vi "Modules - Communications V1.vi"() -> ()   [LabVIEW 2019]
uses:
  Controls/UDP - Command.ctl
  Controls/Communications - State.ctl
  Controls/FTDI - Communication.ctl
  Controls/eFGV States.ctl
  Controls/Communications - Data Structure.ctl
  Controls/Communication - Write Data.ctl
  Controls/UDP - Communication.ctl
  Controls/UDP - Event.ctl
  Controls/UDP - Status.ctl
  Controls/Global - Hold.vi
  Controls/Global - Handle V1.vi
  Controls/Global - IP Address.vi
  <vilib>/Instr/_visa.llb/VISA Serial Break (Instr).vi
  Controls/Global - Device.vi
  Controls/Global - Comport.vi
  Controls/Global - Data UDP.vi
  Controls/Global - Done.vi
  Controls/Global - Channel.vi
  Controls/Global - Unit.vi
  Controls/Global - Rendezvous.vi
panel:
  out "8":T1
  out "Prev 8":bool
  out "Success8":bool
  out "8":T2
  out "loop 8":i32
  out "9":T1
  out "Prev 9":bool
  out "Success9":bool
  out "9":T2
  out "loop 9":i32
  out "10":T1
  out "Prev 10":bool
  out "Success10":bool
  out "10":T2
  out "loop 10":i32
  out "11":T1
  out "Prev 11":bool
  out "Success11":bool
  out "11":T2
  out "loop 11":i32
  out "12":T1
  out "Prev 12":bool
  out "Success12":bool
  out "12":T2
  out "loop 12":i32
  out "13":T1
  out "Prev 13":bool
  out "Success13":bool
  out "13":T2
  out "loop 13":i32
  out "14":T1
  out "Prev 14":bool
  out "Success14":bool
  out "14":T2
  out "loop 14":i32
  out "15":T1
  out "Prev15":bool
  out "Success15":bool
  out "15":T2
  out "loop 15":i32
  out "4":T1
  out "Prev 4":bool
  out "Success4":bool
  out "5":T2
  out "loop 4":i32
  out "5":T1
  out "Prev 5":bool
  out "Success5":bool
  out "5":T2
  out "loop 5":i32
  out "6":T1
  out "Prev 6":bool
  out "Success6":bool
  out "6":T2
  out "loop 6":i32
  out "7":T1
  out "Prev 7":bool
  out "Success7":bool
  out "7":T2
  out "loop 7":i32
  out "UI loop":i32
  out "Success3":bool
  out "Success2":bool
  out "Success1":bool
  out "Success0":bool
  in  "stop":bool
  out "Prev 3":bool
  out "Prev 2":bool
  out "Prev 1":bool
  out "Prev 0":bool
  out "loop 3":i32
  out "loop 2":i32
  out "loop 1":i32
  in  "Enable Termination\nChar (T)":bool=TRUE
  in  "Break":bool
  out "loop 0":i32
  out "3":T2
  out "2":T2
  out "1":T2
  out "0":T2
  out "3":T1
  out "2":T1
  out "1":T1
  out "0":T1
  out "Device":string[](array[string])
  out "SN":string[](array[string])
  out "Stop":bool=TRUE
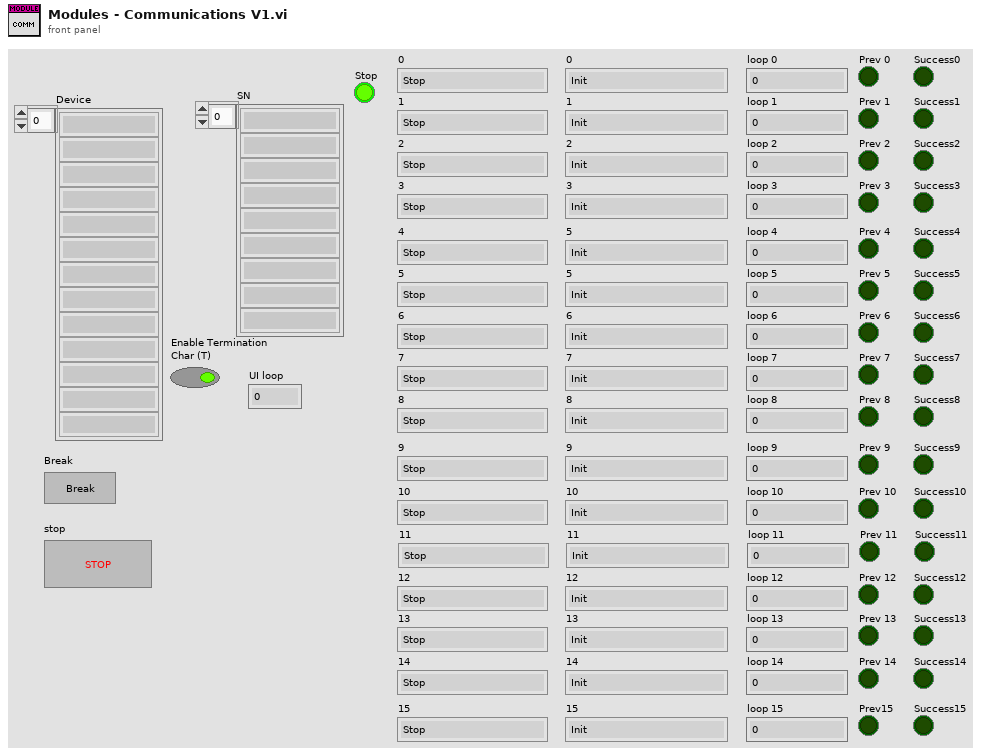
[diagram p1: front panel]
types:
  T1 = typedef "UDP - Command.ctl" = enum16{"Stop", "Jog Up", "Jog Down", "Ramp Up", "Ramp Down", "PID Target", "PID Ramp", "Disp Run", "Read Ch Data", "Zero Channel", "Zero Disp", "Read Sensor", "Write Sensor", "Read ADC", "Write ADC", "Read PID", "Write PID", "Read Test", "Write Test", "Read System", "Write System", "Read Datalog", "Read Datalog Sensor"}
  T2 = typedef "Communications - State.ctl" = enum16{"Init", "Idle", "Command", "Get IP Address", "Release Rendezvous", "Feedback", "Close"}
  T3 = enum32{"Invalid", "Standard", "Closed", "Hidden", "Minimized", "Maximized"}
  T4 = typedef "FTDI - Communication.ctl" = cluster{"IP":string, "CMD":T1, "Port":string, "Datalog?":bool, "Float":dbl}
  T5 = typedef "eFGV States.ctl" = enum16{"Init", "Read", "Write", "Exit"}
  T6 = typedef "Communications - Data Structure.ctl" = cluster{"UDP CMD":T4, "Unit?":bool, "Read Unit":bool[], "Trig?":bool, "UDP Info":cluster{"IP Address":string, "port":string, "UDP ref":refnum<k16>}[], "DataLogger":bool[], "VISA Ref":refnum<event-registration>, "Float":sgl, "Data":T7, "UDP Event Ref":refnum<event-registration>, "UDP ref":refnum<k16>, "Read Sensor":u8}
  T7 = typedef "Communication - Write Data.ctl" = cluster{"Test":cluster{"Target Load":sgl, "Target Disp":sgl, "Rate":sgl, "Speed":sgl}, "Sensor":cluster{"Name":string[], "Unit":string[], "Decimal Point":u8[], "Ch Log":u8[], "H Alarm":u8[], "L Alarm":u8[], "H Limit":sgl[], "L Limit":sgl[], "Filter":u8[], "Gain":u8[], "Calib Type":u32[]}, "PID":cluster{"SP":sgl, "PV":sgl, "kP":sgl, "kI":sgl, "kD":sgl, "FF":sgl, "Err Band":sgl, "Max":i32, "Min":i32, "Ts":u32, "Out":i32, "Mode":u8}, "ADC":cluster{"Active Ch":u8[], "Filter Type":u8, "Post Filter":u8[], "Gain":u8[], "FS":u16, "IntOC":u8, "IntFC":u8, "SysOC":u8, "Cofficient":dbl[], "K":dbl[], "Max":i32}, "System":cluster{"Out Type":u8, "Inverse":u8, "Monitor":u8, "Reserve":u8, "ACC Time":u32, "Pulse Rev":u32, "Stroke":u32, "Auto Off":u32, "Gear Ratio":sgl, "Pitch":sgl, "Max Speed":u32, "Jog Speed":u32, "Disp Coff":sgl, "Max Load":u32}, "Index":enum16{"Ch1", "Ch2", "Ch3", "Ch4", "Ch5", "Ch6", "Ch7", "Ch8", "Ch9", "Ch10", "Ch11", "Ch12", "Ch13", "Ch14", "Ch15", "Ch16"}, "Datalog":enum16{"Ch1-Ch16", "Ch17-Ch32", "Ch32-Ch48", "Ch49-Ch64", "Empty"}}
  T8 = typedef "UDP - Event.ctl" = u16
  T9 = typedef "UDP - Status.ctl" = u16
  T10 = cluster{"Channels":cluster{"Ch1":sgl, "Ch2":sgl, "Ch3":sgl, "Ch4":sgl, "Ch5":sgl, "Ch6":sgl, "Ch7":sgl, "Ch8":sgl, "Ch9":sgl, "Ch10":sgl, "Ch11":sgl, "Ch12":sgl, "Ch13":sgl, "Ch14":sgl, "Ch15":sgl, "Ch16":sgl}, "Event":T8, "Status":T9, "IP":string}
  T11 = cluster{"Name":string[], "Unit":string[], "Decimal Point":u8[], "Ch Log":u8[], "H Alarm":u8[], "L Alarm":u8[], "H Limit":sgl[], "L Limit":sgl[], "Filter":u8[], "Gain":u8[], "Calib Type":u32[]}
  T12 = cluster{"Ch1 Unit":string, "Ch2 Unit":string, "Ch1 Decimal":u8, "Ch2 Decimal":u8, "Ch1 Cal Type":u8, "Ch2 Cal Type":u8}
  T13 = cluster{"Ch1 Status":u8, "Ch2 Status":u8, "DO":bool[], "DI":bool[], "Ch1 Data":sgl, "Ch2 Data":sgl}
  T14 = cluster{"Channels":cluster{"Ch1":sgl, "Ch2":sgl, "Ch3":sgl, "Ch4":sgl, "Ch5":sgl, "Ch6":sgl, "Ch7":sgl, "Ch8":sgl, "Ch9":sgl, "Ch10":sgl, "Ch11":sgl, "Ch12":sgl, "Ch13":sgl, "Ch14":sgl, "Ch15":sgl, "Ch16":sgl}, "Event":T8, "Status":T9, "IP":string}[]
  T15 = cluster{"Name":string[], "Unit":string[], "Decimal Point":u8[], "Ch Log":u8[], "H Alarm":u8[], "L Alarm":u8[], "H Limit":sgl[], "L Limit":sgl[], "Filter":u8[], "Gain":u8[], "Calib Type":u32[]}[]
  T16 = typedef "Rendezvous RefNum" = refnum<k1>
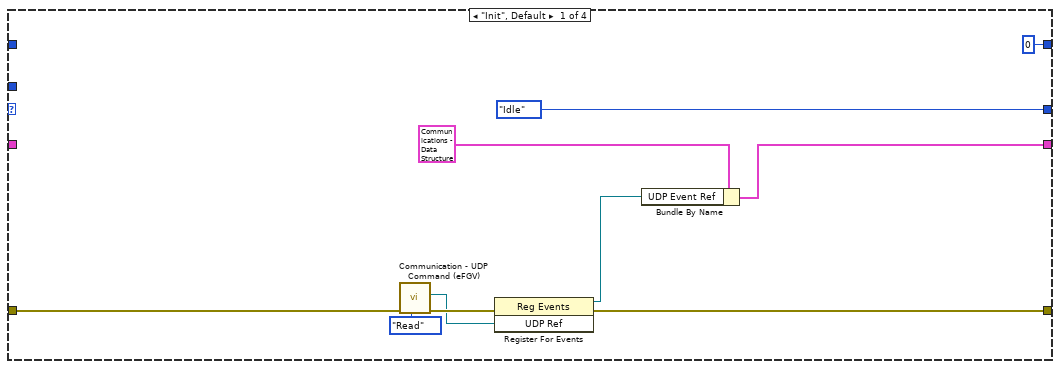
[diagram p2: hidden frame]
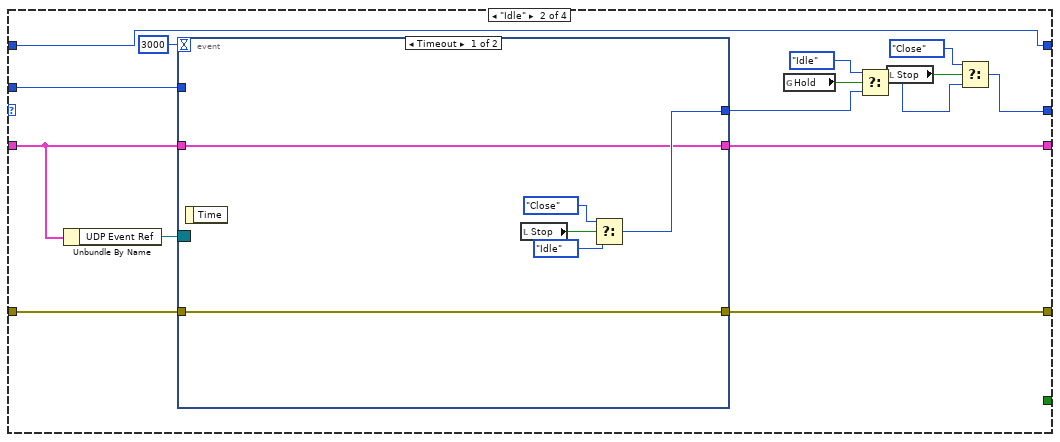
[diagram p3: hidden frame]
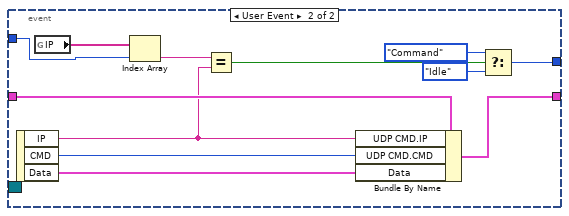
[diagram p4: hidden frame]
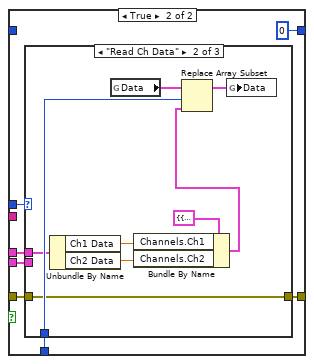
[diagram p6: hidden frame]
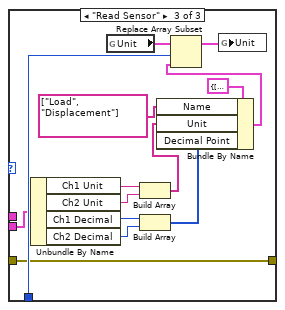
[diagram p8: hidden frame]
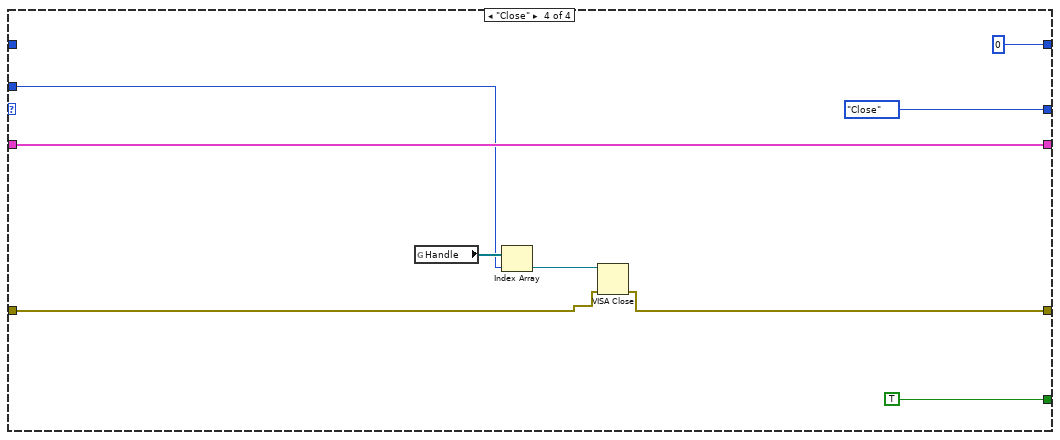
[diagram p9: hidden frame]
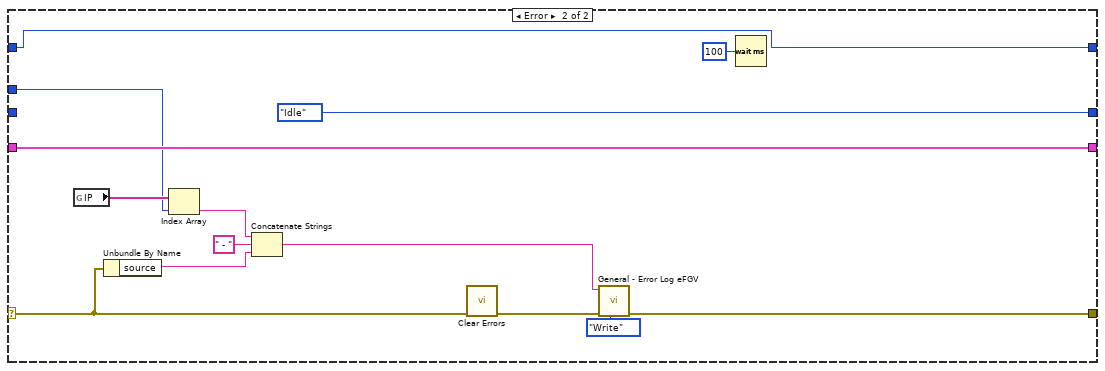
[diagram p10: hidden frame]
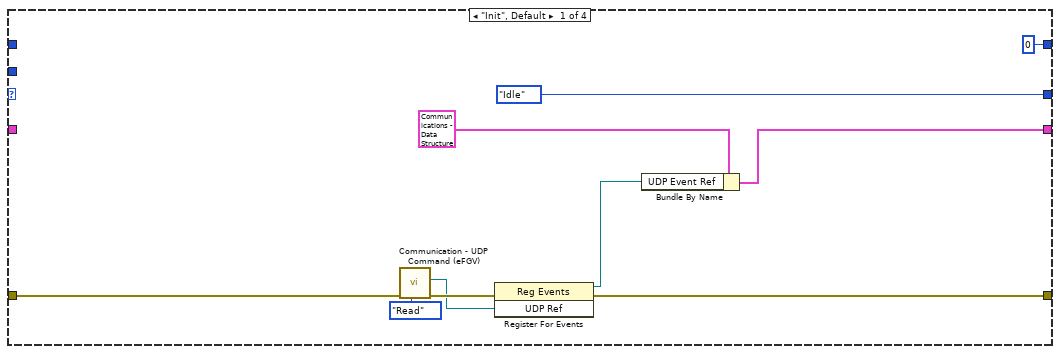
[diagram p11: hidden frame]
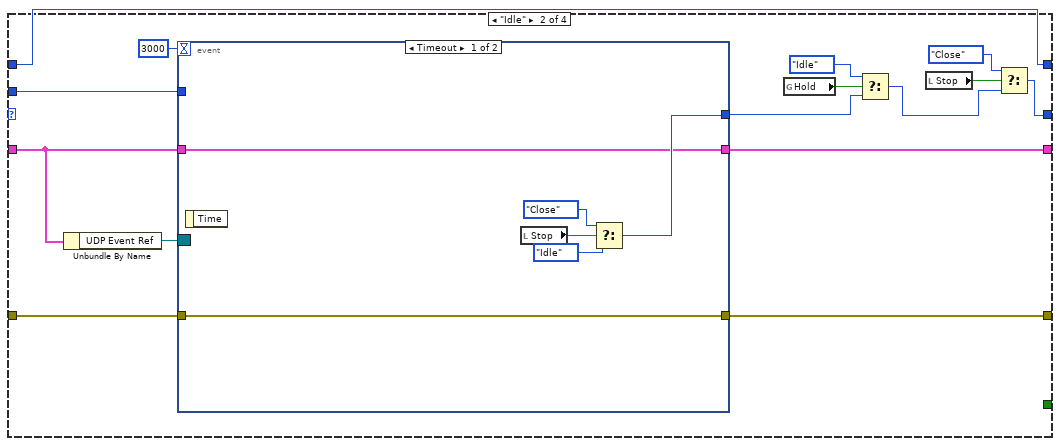
[diagram p12: hidden frame]
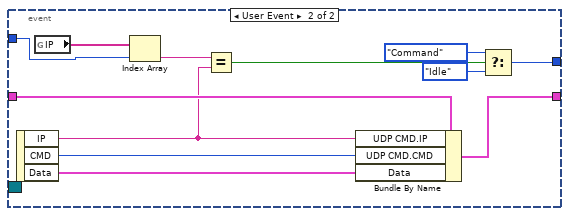
[diagram p13: hidden frame]
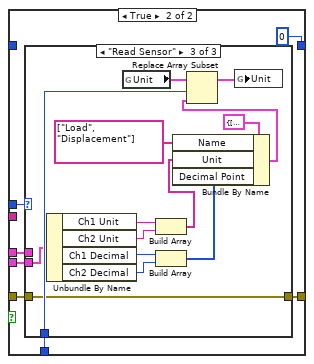
[diagram p15: hidden frame]
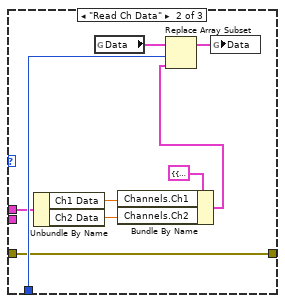
[diagram p17: hidden frame]
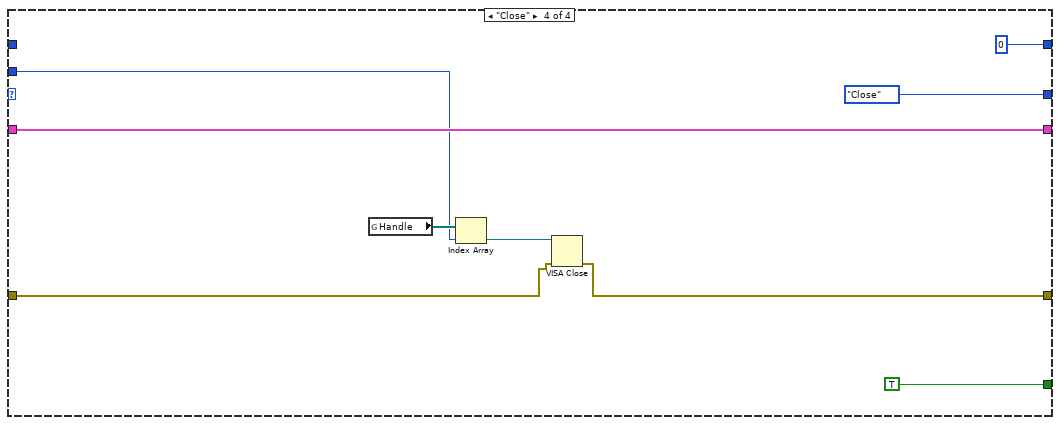
[diagram p18: hidden frame]
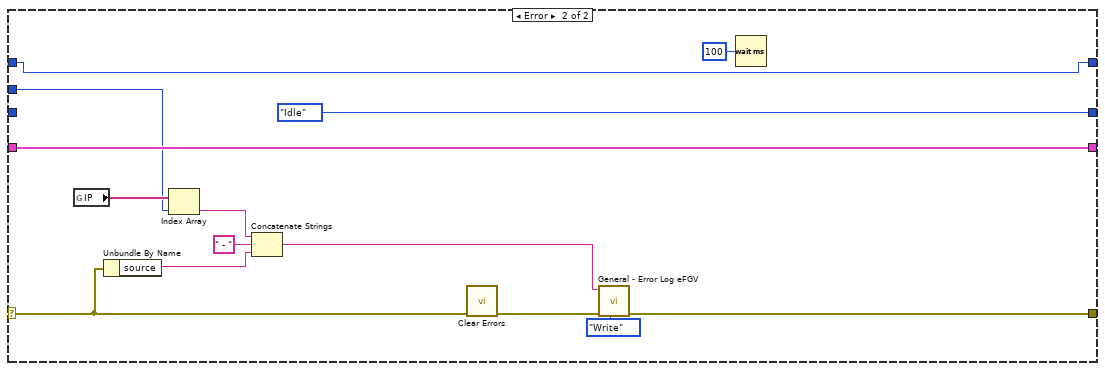
[diagram p19: hidden frame]
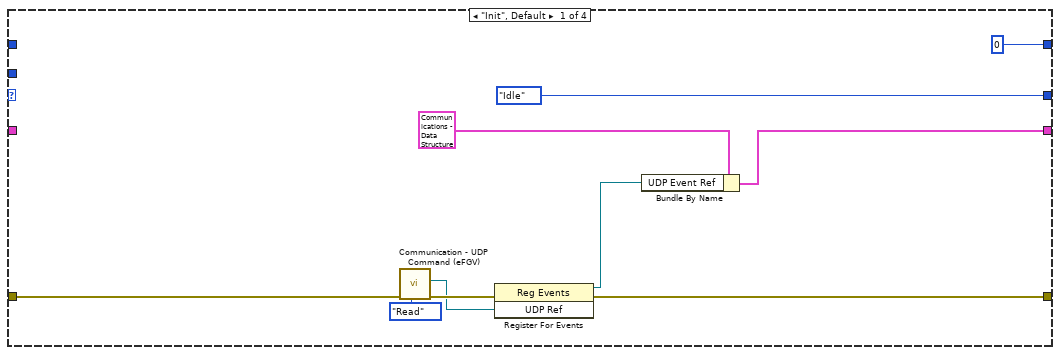
[diagram p20: hidden frame]
diagram:
  (unwired) Communications_-_State."Init"
  (unwired) Communications_-_State."Init"
  (unwired) Communications_-_State."Init"
  (unwired) Communications_-_State."Init"
  (unwired) Communications_-_State."Init"
  (unwired) Communications_-_State."Init"
  (unwired) Communications_-_State."Init"
  (unwired) Communications_-_State."Init"
  (unwired) Communications_-_State."Init"
  (unwired) Communications_-_State."Init"
  (unwired) Communications_-_State."Init"
  (unwired) Communications_-_State."Init"
  (unwired) Communications_-_State."Init"
  (unwired) Communications_-_State."Init"
  (unwired) Communications_-_State."Init"
  (unwired) Communications_-_State."Init"
  (unwired) T4 {"IP"="", "CMD"=enum."Stop", "Port"="", "Datalog?"=FALSE, "Float"=0.0}
  (unwired) Communications_-_State."Init"
  n1 = while {
    shift-right: [w68] -> _
    shift-left: errorcluster {"status"=FALSE, "code"=0, "source"=""} ("error IO") -> [w69]
    shift-right: [w66] -> _
    shift-left: Communications_-_State."Init" -> [w67]
    shift-right: [w64] -> _
    shift-left: _ -> [w63]
    tunnel: 0 ("index") -> [w62]
    shift-right: [w60] -> _
    shift-left: _ -> [w59]
    i -> [w61]
    stop <- w65 stop-if-true
    # "Queue Command Processing Loop"
    n2 = case shown="No Error" w69 {
      selector: w69 -> [w78 w212]
      tunnel: [w79 w206] -> w68
      tunnel: w67 -> [w77 _]
      tunnel: [w76 Communications_-_State."Idle"] -> w66
      tunnel: [w75 _] -> w65
      tunnel: [w74 w214] -> w64
      tunnel: w63 -> [w73 w214]
      tunnel: w62 -> [w72 w203]
      tunnel: [w71 w202] -> w60
      tunnel: w59 -> [w70 w202]
      frame No Error {
        n3 = case shown="\"Command\"" w77 {
          tunnel: [w83 w103 w138 w193] -> w79
          tunnel: w78 -> [w88 w102 w141 w197]
          tunnel: [Communications_-_State."Idle" w91 Communications_-_State."Idle" Communications_-_State."Close"] -> w76
          tunnel: [_ _ _ TRUE] -> w75
          tunnel: [w85 w101 w140 w199] -> w74
          tunnel: w73 -> [_ w100 w140 w199]
          tunnel: w72 -> [_ w95 w127 w195]
          tunnel: [0 ("index") w90 w126 0 ("index")] -> w71
          tunnel: w70 -> [_ w90 w125 _]
          frame "Init", Default {
            n4 = call "Communication - UDP Command (eFGV).vi"("Action"=eFGV_States."Read", "error in"=w88) -> ("error out"=w84:errorcluster, "UDP Ref"=w82:refnum<user-event>)  [unwired: 7 in, 1 out]
            n5 = register-events(error in=w84, w82) -> (reference out=w81:refnum<event-registration>, error out=w83:errorcluster)  [unwired: 1 in]
            n6 = Bundle By Name(cluster=T6 {"UDP CMD"={"IP"="", "CMD"=enum."Stop", "Port"="", "Datalog?"=FALSE, "Float"=0.0}, "Unit?"=FALSE, "Read Unit"=[], "Trig?"=FALSE, "UDP Info"=[], "DataLogger"=[], "VISA Ref"=refnum, "Float"=0.0, "Data"={"Test"={"Target Load"=0.0, "Target Disp"=0.0, "Rate"=0.0, "Speed"=0.0}, "Sensor"={"Name"=[], "Unit"=[], "Decimal Point"=[], "Ch Log"=[], "H Alarm"=[], "L Alarm"=[], "H Limit"=[], "L Limit"=[], "Filter"=[], "Gain"=[], "Calib Type"=[]}, "PID"={"SP"=-2.7823365e-08, "PV"=-3.023652e-13, "kP"=8.5432666e-24, "kI"=2.29252e-41, "kD"=1.570387e-38, "FF"=25.0, "Err Band"=0.0, "Max"=15, "Min"=-7, "Ts"=1886611780, "Out"=0, "Mode"=0}, "ADC"={"Active Ch"=[255, 255, 255, 0, 0, 0, 0, 0], "Filter Type"=2, "Post Filter"=[1, 1, 1, 1, 0, 200, 66, 184], "Gain"=[0, 0, 0, 0, 0, 122, 68, 0], "FS"=32, "IntOC"=0, "IntFC"=255, "SysOC"=255, "Cofficient"=[1.0, 1.0, 1.0, 1.0, 1.0, 1.0, 1.0, 1.0], "K"=[1.2450000047683716, 1.2450000047683716], "Max"=1048576}, "System"={"Out Type"=0, "Inverse"=0, "Monitor"=0, "Reserve"=0, "ACC Time"=0, "Pulse Rev"=0, "Stroke"=0, "Auto Off"=0, "Gear Ratio"=0.0, "Pitch"=0.0, "Max Speed"=0, "Jog Speed"=0, "Disp Coff"=0.0, "Max Load"=0}, "Index"=enum."Ch1", "Datalog"=enum."Empty"}, "UDP Event Ref"=refnum, "UDP ref"=refnum, "Read Sensor"=0}, "UDP Event Ref"=w81) -> (w85:T6)
          }
          frame "Idle" {
            n7 = Unbundle By Name(w100) -> ("UDP Event Ref"=w104:refnum<event-registration>)
            n8 = event shown="[0] Timeout" {
              selector: w104 -> [_ _]
              dyn-events: _ -> [_ _]
              timeout: 3000 -> [_ _]
              tunnel: [w110 w113] -> w98
              tunnel: [w107 _] -> w103
              tunnel: w102 -> [w107 _]
              tunnel: [w105 w122] -> w101
              tunnel: w100 -> [w105 w121]
              tunnel: w95 -> [_ w111]
              event Timeout {
                n9 = event-data() -> ()  [unwired: 1 in, 1 out]
                n10 = local read "Stop"() -> (w109:bool)
                n11 = Select(t=Communications_-_State."Close", s=w109, f=Communications_-_State."Idle") -> (s? t:f=w110:T2)
              }
              event User Event {
                n12 = event-data() -> ("IP"=w116:string, "CMD"=w120:T1, "Data"=w119:T7)  [unwired: 1 in]
                n13 = global read "Global - IP Address.vi" "IP"() -> (w118:string[])
                n14 = Index Array(array=w118, index=w111) -> (element=w117:string)
                n15 = Equal?(x=w117, y=w116) -> (x = y?=w115:bool)
                n16 = Bundle By Name(cluster=w121, "UDP CMD.IP"=w116, "UDP CMD.CMD"=w120, "Data"=w119) -> (w122:T6)
                n17 = Select(t=Communications_-_State."Command" ("f"), s=w115, f=Communications_-_State."Idle") -> (s? t:f=w113:T2)
              }
            }
            n18 = global read "Global - Hold.vi" "Hold"() -> (w99:bool)
            n19 = Select(t=Communications_-_State."Idle", s=w99, f=w98) -> (s? t:f=w92:T2)
            n20 = local read "Stop"() -> (w93:bool)
            n21 = Select(t=Communications_-_State."Close", s=w93, f=w92) -> (s? t:f=w91:T2)
          }
          frame "Command" {
            n22 = Unbundle By Name(w140) -> ("UDP CMD.CMD"=w137:T1, "Data"=w139:T7, "UDP CMD.IP"=w123:string)
            "0" <- w137
            n23 = global read "Global - Handle V1.vi" "Handle"() -> (w131:refnum<visa-resource-name>[])
            n24 = global read "Global - IP Address.vi" "IP"() -> (w132:string[])
            n25 = Search 1D Array(1D array=w132, element=w123) -> ()  [unwired: 1 in, 1 out]
            n26 = Index Array(array=w131, index=w127) -> (element=w133:refnum<visa-resource-name>)
            n27 = call "VISA - Write CMD.vi"("Index"=w127, "error in"=w141, "Data"=w139, "Action"=w137, "VISA ref"=w133) -> ("error out"=w129:errorcluster, "Data Unit"=w135:T12, "Data Channel"=w136:T13, "Success"=w134:bool, "Prev Data?"=→"Prev 0":bool)  [unwired: 2 out]
            "Success0" <- w134
            n28 = flat-sequence {
              tunnel: w127 -> [w147]
              tunnel: [w144] -> w130
              tunnel: w129 -> [w144]
              frame #0 {
                n29 = global read "Global - Done.vi" "Done"() -> (w146:bool[])
                n30 = Replace Array Subset(array=w146, new element=TRUE, index=w147) -> (w145:bool[])
                n31 = global write "Global - Done.vi" "Done"(w145) -> ()
              }
            }
            n32 = global write "Global - Data UDP.vi" "Loop 1"(TRUE ("Loop 1")) -> ()
            n33 = case shown="False" w134 {
              tunnel: w130 -> [w151 w166]
              tunnel: [w152 w165] -> w138
              tunnel: w137 -> [_ w167]
              tunnel: w136 -> [_ w164]
              tunnel: w135 -> [_ w163]
              tunnel: w127 -> [_ w162]
              tunnel: [w148 0 ("index")] -> w126
              tunnel: w125 -> [w153 _]
              tunnel: w123 -> [w149 _]
              frame False {
                n34 = Increment(x=w153) -> (x+1=w150:i32)
                n35 = case shown="0, Default" w150 {
                  selector: w150 -> [w154 _]
                  tunnel: [w155 w160] -> w152
                  tunnel: w151 -> [w155 w159]
                  tunnel: w149 -> [_ w157]
                  tunnel: [w154 0] -> w148
                  frame 0, Default {
                  }
                  frame 5 {
                    n36 = call "Communication - Reconnect eFGV.vi"("eFGV States"=eFGV_States."Write", "error in (no error)"=w159, "Reconnect In"=w157) -> ("error out"=w160:errorcluster)  [unwired: 6 in, 2 out]
                  }
                }
              }
              frame True {
                n37 = case shown="\"Read Ch Data\"" w167 {
                  tunnel: w166 -> [w168 w175 w190]
                  tunnel: [w168 w175 w190] -> w165
                  tunnel: w164 -> [_ w173 _]
                  tunnel: w163 -> [_ _ w186]
                  tunnel: w162 -> [_ w177 w191]
                  frame "Stop", Default {
                  }
                  frame "Read Ch Data" {
                    n38 = Unbundle By Name(w173) -> ("Ch1 Data"=w172:sgl, "Ch2 Data"=w171:sgl)
                    n39 = global read "Global - Channel.vi" "Data"() -> (w176:T14)
                    n40 = Bundle By Name(cluster=T10 {"Channels"={"Ch1"=0.0, "Ch2"=0.0, "Ch3"=0.0, "Ch4"=0.0, "Ch5"=0.0, "Ch6"=0.0, "Ch7"=0.0, "Ch8"=0.0, "Ch9"=0.0, "Ch10"=0.0, "Ch11"=0.0, "Ch12"=0.0, "Ch13"=0.0, "Ch14"=0.0, "Ch15"=0.0, "Ch16"=0.0}, "Event"=0, "Status"=0, "IP"=""} ("Data Channel"), "Channels.Ch1"=w172, "Channels.Ch2"=w171) -> (w170:T10)
                    n41 = Replace Array Subset(array=w176, new element=w170, index=w177) -> (w174:T14)
                    n42 = global write "Global - Channel.vi" "Data"(w174) -> ()
                  }
                  frame "Read Sensor" {
                    n43 = Unbundle By Name(w186) -> ("Ch1 Unit"=w185:string, "Ch2 Unit"=w184:string, "Ch1 Decimal"=w183:u8, "Ch2 Decimal"=w182:u8)
                    n44 = global read "Global - Unit.vi" "Unit"() -> (w188:T15)
                    n45 = Build Array(w185, w184) -> (w181:string[])
                    n46 = Build Array(w183, w182) -> (w180:u8[])
                    n47 = Bundle By Name(cluster=T11 {"Name"=[], "Unit"=[], "Decimal Point"=[], "Ch Log"=[], "H Alarm"=[], "L Alarm"=[], "H Limit"=[], "L Limit"=[], "Filter"=[], "Gain"=[], "Calib Type"=[]} ("Sensor"), "Name"=string[] ["Load", "Displacement"], "Unit"=w181, "Decimal Point"=w180) -> (w179:T11)
                    n48 = Replace Array Subset(array=w188, new element=w179, index=w191) -> (w189:T15)
                    n49 = global write "Global - Unit.vi" "Unit"(w189) -> ()
                  }
                }
              }
            }
          }
          frame "Close" {
            n50 = global read "Global - Handle V1.vi" "Handle"() -> (w196:refnum<visa-resource-name>[])
            n51 = Index Array(array=w196, index=w195) -> (element=w194:refnum<visa-resource-name>)
            n52 = VISA Close(VISA resource name=w194, error in (no error)=w197) -> (error out=w198:errorcluster)
            n53 = call <vilib>:"Clear Errors.vi"("error in (no error)"=w198) -> ("error out"=w193:errorcluster)  [unwired: 5 in, 1 out]
          }
        }
      }
      frame Error {
        n54 = global read "Global - IP Address.vi" "IP"() -> (w211:string[])
        n55 = Unbundle By Name(w212) -> ("source"=w208:string)
        n56 = Index Array(array=w211, index=w203) -> (element=w210:string)
        n57 = Concatenate Strings(w210, " - " ("string"), w208) -> (w204:string)
        n58 = call <vilib>:"Clear Errors.vi"("error in (no error)"=w212) -> ("error out"=w207:errorcluster)  [unwired: 5 in, 1 out]
        n59 = call "General - Error Log eFGV.vi"("eFGV States"=eFGV_States."Write", "error in (no error)"=w207, "Error In"=w204) -> ("error out"=w206:errorcluster)  [unwired: 6 in, 2 out]
        n60 = Wait (ms)(milliseconds to wait=u32 100) -> ()  [unwired: 1 out]
      }
    }
    "0" <- w67
    "loop 0" <- w61
  }
  n61 = while {
    shift-right: [w225] -> _
    shift-left: errorcluster {"status"=FALSE, "code"=0, "source"=""} ("error IO") -> [w226]
    shift-right: [w223] -> _
    shift-left: Communications_-_State."Init" -> [w224]
    shift-right: [w221] -> _
    shift-left: _ -> [w220]
    tunnel: 2 ("index") -> [w219]
    shift-right: [w217] -> _
    shift-left: _ -> [w216]
    i -> [w218]
    stop <- w222 stop-if-true
    # "Queue Command Processing Loop"
    n62 = case shown="No Error" w226 {
      selector: w226 -> [w235 w368]
      tunnel: [w236 w362] -> w225
      tunnel: w224 -> [w234 _]
      tunnel: [w233 Communications_-_State."Idle"] -> w223
      tunnel: [w232 _] -> w222
      tunnel: [w231 w370] -> w221
      tunnel: w220 -> [w230 w370]
      tunnel: w219 -> [w229 w359]
      tunnel: [w228 w358] -> w217
      tunnel: w216 -> [w227 w358]
      frame No Error {
        n63 = case shown="\"Command\"" w234 {
          tunnel: [w240 w260 w295 w352] -> w236
          tunnel: w235 -> [w245 w259 w298 w351]
          tunnel: [Communications_-_State."Idle" w248 Communications_-_State."Idle" Communications_-_State."Close"] -> w233
          tunnel: [_ _ _ TRUE] -> w232
          tunnel: [w242 w258 w297 w355] -> w231
          tunnel: w230 -> [_ w257 w297 w355]
          tunnel: w229 -> [_ w252 w284 w350]
          tunnel: [0 w247 w282 0] -> w228
          tunnel: w227 -> [_ w247 w281 _]
          frame "Init", Default {
            n64 = call "Communication - UDP Command (eFGV).vi"("Action"=eFGV_States."Read", "error in"=w245) -> ("error out"=w241:errorcluster, "UDP Ref"=w239:refnum<user-event>)  [unwired: 7 in, 1 out]
            n65 = register-events(error in=w241, w239) -> (reference out=w238:refnum<event-registration>, error out=w240:errorcluster)  [unwired: 1 in]
            n66 = Bundle By Name(cluster=T6 {"UDP CMD"={"IP"="", "CMD"=enum."Stop", "Port"="", "Datalog?"=FALSE, "Float"=0.0}, "Unit?"=FALSE, "Read Unit"=[], "Trig?"=FALSE, "UDP Info"=[], "DataLogger"=[], "VISA Ref"=refnum, "Float"=0.0, "Data"={"Test"={"Target Load"=0.0, "Target Disp"=0.0, "Rate"=0.0, "Speed"=0.0}, "Sensor"={"Name"=[], "Unit"=[], "Decimal Point"=[], "Ch Log"=[], "H Alarm"=[], "L Alarm"=[], "H Limit"=[], "L Limit"=[], "Filter"=[], "Gain"=[], "Calib Type"=[]}, "PID"={"SP"=-2.7823365e-08, "PV"=-3.023652e-13, "kP"=8.5432666e-24, "kI"=2.29252e-41, "kD"=1.570387e-38, "FF"=25.0, "Err Band"=0.0, "Max"=15, "Min"=-7, "Ts"=1886611780, "Out"=0, "Mode"=0}, "ADC"={"Active Ch"=[255, 255, 255, 0, 0, 0, 0, 0], "Filter Type"=2, "Post Filter"=[1, 1, 1, 1, 0, 200, 66, 184], "Gain"=[0, 0, 0, 0, 0, 122, 68, 0], "FS"=32, "IntOC"=0, "IntFC"=255, "SysOC"=255, "Cofficient"=[1.0, 1.0, 1.0, 1.0, 1.0, 1.0, 1.0, 1.0], "K"=[1.2450000047683716, 1.2450000047683716], "Max"=1048576}, "System"={"Out Type"=0, "Inverse"=0, "Monitor"=0, "Reserve"=0, "ACC Time"=0, "Pulse Rev"=0, "Stroke"=0, "Auto Off"=0, "Gear Ratio"=0.0, "Pitch"=0.0, "Max Speed"=0, "Jog Speed"=0, "Disp Coff"=0.0, "Max Load"=0}, "Index"=enum."Ch1", "Datalog"=enum."Empty"}, "UDP Event Ref"=refnum, "UDP ref"=refnum, "Read Sensor"=0}, "UDP Event Ref"=w238) -> (w242:T6)
          }
          frame "Idle" {
            n67 = Unbundle By Name(w257) -> ("UDP Event Ref"=w261:refnum<event-registration>)
            n68 = event shown="[0] Timeout" {
              selector: w261 -> [_ _]
              dyn-events: _ -> [_ _]
              timeout: 3000 -> [_ _]
              tunnel: [w267 w270] -> w255
              tunnel: [w264 _] -> w260
              tunnel: w259 -> [w264 _]
              tunnel: [w262 w279] -> w258
              tunnel: w257 -> [w262 w278]
              tunnel: w252 -> [_ w268]
              event Timeout {
                n69 = event-data() -> ()  [unwired: 1 in, 1 out]
                n70 = local read "Stop"() -> (w266:bool)
                n71 = Select(t=Communications_-_State."Close", s=w266, f=Communications_-_State."Idle") -> (s? t:f=w267:T2)
              }
              event User Event {
                n72 = event-data() -> ("IP"=w273:string, "CMD"=w277:T1, "Data"=w276:T7)  [unwired: 1 in]
                n73 = global read "Global - IP Address.vi" "IP"() -> (w275:string[])
                n74 = Index Array(array=w275, index=w268) -> (element=w274:string)
                n75 = Equal?(x=w274, y=w273) -> (x = y?=w272:bool)
                n76 = Bundle By Name(cluster=w278, "UDP CMD.IP"=w273, "UDP CMD.CMD"=w277, "Data"=w276) -> (w279:T6)
                n77 = Select(t=Communications_-_State."Command" ("f"), s=w272, f=Communications_-_State."Idle") -> (s? t:f=w270:T2)
              }
            }
            n78 = global read "Global - Hold.vi" "Hold"() -> (w256:bool)
            n79 = Select(t=Communications_-_State."Idle", s=w256, f=w255) -> (s? t:f=w249:T2)
            n80 = local read "Stop"() -> (w250:bool)
            n81 = Select(t=Communications_-_State."Close", s=w250, f=w249) -> (s? t:f=w248:T2)
          }
          frame "Command" {
            n82 = Unbundle By Name(w297) -> ("UDP CMD.CMD"=w294:T1, "Data"=w296:T7, "UDP CMD.IP"=w280:string)
            "2" <- w294
            n83 = global read "Global - Handle V1.vi" "Handle"() -> (w288:refnum<visa-resource-name>[])
            n84 = global read "Global - IP Address.vi" "IP"() -> (w289:string[])
            n85 = Search 1D Array(1D array=w289, element=w280) -> ()  [unwired: 1 in, 1 out]
            n86 = Index Array(array=w288, index=w284) -> (element=w290:refnum<visa-resource-name>)
            n87 = call "VISA - Write CMD.vi"("Index"=w284, "error in"=w298, "Data"=w296, "Action"=w294, "VISA ref"=w290) -> ("error out"=w286:errorcluster, "Data Unit"=w292:T12, "Data Channel"=w293:T13, "Success"=w291:bool, "Prev Data?"=→"Prev 2":bool)  [unwired: 2 out]
            "Success2" <- w291
            n88 = flat-sequence {
              tunnel: w284 -> [w304]
              tunnel: [w301] -> w287
              tunnel: w286 -> [w301]
              frame #0 {
                n89 = global read "Global - Done.vi" "Done"() -> (w303:bool[])
                n90 = Replace Array Subset(array=w303, new element=TRUE, index=w304) -> (w302:bool[])
                n91 = global write "Global - Done.vi" "Done"(w302) -> ()
              }
            }
            n92 = global write "Global - Data UDP.vi" "Loop 3"(TRUE ("Loop 3")) -> ()
            n93 = case shown="False" w291 {
              tunnel: w287 -> [w308 w323]
              tunnel: [w309 w322] -> w295
              tunnel: w294 -> [_ w324]
              tunnel: w293 -> [_ w321]
              tunnel: w292 -> [_ w320]
              tunnel: w284 -> [_ w319]
              tunnel: [w305 0] -> w282
              tunnel: w281 -> [w310 _]
              tunnel: w280 -> [w307 _]
              frame False {
                n94 = Increment(x=w310) -> (x+1=w306:i32)
                n95 = case shown="5" w306 {
                  selector: w306 -> [w311 _]
                  tunnel: [w312 w316] -> w309
                  tunnel: w308 -> [w312 w315]
                  tunnel: w307 -> [_ w314]
                  tunnel: [w311 0] -> w305
                  frame 0, Default {
                  }
                  frame 5 {
                    n96 = call "Communication - Reconnect eFGV.vi"("eFGV States"=eFGV_States."Write", "error in (no error)"=w315, "Reconnect In"=w314) -> ("error out"=w316:errorcluster)  [unwired: 6 in, 2 out]
                  }
                }
              }
              frame True {
                n97 = case shown="\"Read Sensor\"" w324 {
                  tunnel: w323 -> [w325 w332 w347]
                  tunnel: [w325 w332 w347] -> w322
                  tunnel: w321 -> [_ w330 _]
                  tunnel: w320 -> [_ _ w343]
                  tunnel: w319 -> [_ w334 w348]
                  frame "Stop", Default {
                  }
                  frame "Read Ch Data" {
                    n98 = Unbundle By Name(w330) -> ("Ch1 Data"=w329:sgl, "Ch2 Data"=w328:sgl)
                    n99 = global read "Global - Channel.vi" "Data"() -> (w333:T14)
                    n100 = Bundle By Name(cluster=T10 {"Channels"={"Ch1"=0.0, "Ch2"=0.0, "Ch3"=0.0, "Ch4"=0.0, "Ch5"=0.0, "Ch6"=0.0, "Ch7"=0.0, "Ch8"=0.0, "Ch9"=0.0, "Ch10"=0.0, "Ch11"=0.0, "Ch12"=0.0, "Ch13"=0.0, "Ch14"=0.0, "Ch15"=0.0, "Ch16"=0.0}, "Event"=0, "Status"=0, "IP"=""} ("Data Channel"), "Channels.Ch1"=w329, "Channels.Ch2"=w328) -> (w327:T10)
                    n101 = Replace Array Subset(array=w333, new element=w327, index=w334) -> (w331:T14)
                    n102 = global write "Global - Channel.vi" "Data"(w331) -> ()
                  }
                  frame "Read Sensor" {
                    n103 = Unbundle By Name(w343) -> ("Ch1 Unit"=w342:string, "Ch2 Unit"=w341:string, "Ch1 Decimal"=w340:u8, "Ch2 Decimal"=w339:u8)
                    n104 = global read "Global - Unit.vi" "Unit"() -> (w345:T15)
                    n105 = Build Array(w342, w341) -> (w338:string[])
                    n106 = Build Array(w340, w339) -> (w337:u8[])
                    n107 = Bundle By Name(cluster=T11 {"Name"=[], "Unit"=[], "Decimal Point"=[], "Ch Log"=[], "H Alarm"=[], "L Alarm"=[], "H Limit"=[], "L Limit"=[], "Filter"=[], "Gain"=[], "Calib Type"=[]} ("Sensor"), "Name"=string[] ["Load", "Displacement"], "Unit"=w338, "Decimal Point"=w337) -> (w336:T11)
                    n108 = Replace Array Subset(array=w345, new element=w336, index=w348) -> (w346:T15)
                    n109 = global write "Global - Unit.vi" "Unit"(w346) -> ()
                  }
                }
              }
            }
          }
          frame "Close" {
            n110 = global read "Global - Handle V1.vi" "Handle"() -> (w354:refnum<visa-resource-name>[])
            n111 = Index Array(array=w354, index=w350) -> (element=w353:refnum<visa-resource-name>)
            n112 = VISA Close(VISA resource name=w353, error in (no error)=w351) -> (error out=w352:errorcluster)
          }
        }
      }
      frame Error {
        n113 = global read "Global - IP Address.vi" "IP"() -> (w367:string[])
        n114 = Unbundle By Name(w368) -> ("source"=w364:string)
        n115 = Index Array(array=w367, index=w359) -> (element=w366:string)
        n116 = Concatenate Strings(w366, " - " ("string"), w364) -> (w360:string)
        n117 = call <vilib>:"Clear Errors.vi"("error in (no error)"=w368) -> ("error out"=w363:errorcluster)  [unwired: 5 in, 1 out]
        n118 = call "General - Error Log eFGV.vi"("eFGV States"=eFGV_States."Write", "error in (no error)"=w363, "Error In"=w360) -> ("error out"=w362:errorcluster)  [unwired: 6 in, 2 out]
        n119 = Wait (ms)(milliseconds to wait=u32 100) -> ()  [unwired: 1 out]
      }
    }
    "2" <- w224
    "loop 2" <- w218
  }
  n120 = while {
    shift-right: [w381] -> _
    shift-left: errorcluster {"status"=FALSE, "code"=0, "source"=""} ("error IO") -> [w382]
    shift-right: [w379] -> _
    shift-left: Communications_-_State."Init" -> [w380]
    shift-right: [w377] -> _
    shift-left: _ -> [w376]
    tunnel: 4 ("index") -> [w375]
    shift-right: [w373] -> _
    shift-left: _ -> [w372]
    i -> [w374]
    stop <- w378 stop-if-true
    # "Queue Command Processing Loop"
    n121 = case shown="No Error" w382 {
      selector: w382 -> [w391 w525]
      tunnel: [w392 w519] -> w381
      tunnel: w380 -> [w390 _]
      tunnel: [w389 Communications_-_State."Idle"] -> w379
      tunnel: [w388 _] -> w378
      tunnel: [w387 w527] -> w377
      tunnel: w376 -> [w386 w527]
      tunnel: w375 -> [w385 w516]
      tunnel: [w384 w515] -> w373
      tunnel: w372 -> [w383 w515]
      frame No Error {
        n122 = case shown="\"Command\"" w390 {
          tunnel: [w396 w416 w451 w506] -> w392
          tunnel: w391 -> [w401 w415 w454 w510]
          tunnel: [Communications_-_State."Idle" w404 Communications_-_State."Idle" Communications_-_State."Close"] -> w389
          tunnel: [_ _ _ TRUE] -> w388
          tunnel: [w398 w414 w453 w512] -> w387
          tunnel: w386 -> [_ w413 w453 w512]
          tunnel: w385 -> [_ w408 w440 w508]
          tunnel: [0 ("index") w403 w439 0 ("index")] -> w384
          tunnel: w383 -> [_ w403 w438 _]
          frame "Init", Default {
            n123 = call "Communication - UDP Command (eFGV).vi"("Action"=eFGV_States."Read", "error in"=w401) -> ("error out"=w397:errorcluster, "UDP Ref"=w395:refnum<user-event>)  [unwired: 7 in, 1 out]
            n124 = register-events(error in=w397, w395) -> (reference out=w394:refnum<event-registration>, error out=w396:errorcluster)  [unwired: 1 in]
            n125 = Bundle By Name(cluster=T6 {"UDP CMD"={"IP"="", "CMD"=enum."Stop", "Port"="", "Datalog?"=FALSE, "Float"=0.0}, "Unit?"=FALSE, "Read Unit"=[], "Trig?"=FALSE, "UDP Info"=[], "DataLogger"=[], "VISA Ref"=refnum, "Float"=0.0, "Data"={"Test"={"Target Load"=0.0, "Target Disp"=0.0, "Rate"=0.0, "Speed"=0.0}, "Sensor"={"Name"=[], "Unit"=[], "Decimal Point"=[], "Ch Log"=[], "H Alarm"=[], "L Alarm"=[], "H Limit"=[], "L Limit"=[], "Filter"=[], "Gain"=[], "Calib Type"=[]}, "PID"={"SP"=-2.7823365e-08, "PV"=-3.023652e-13, "kP"=8.5432666e-24, "kI"=2.29252e-41, "kD"=1.570387e-38, "FF"=25.0, "Err Band"=0.0, "Max"=15, "Min"=-7, "Ts"=1886611780, "Out"=0, "Mode"=0}, "ADC"={"Active Ch"=[255, 255, 255, 0, 0, 0, 0, 0], "Filter Type"=2, "Post Filter"=[1, 1, 1, 1, 0, 200, 66, 184], "Gain"=[0, 0, 0, 0, 0, 122, 68, 0], "FS"=32, "IntOC"=0, "IntFC"=255, "SysOC"=255, "Cofficient"=[1.0, 1.0, 1.0, 1.0, 1.0, 1.0, 1.0, 1.0], "K"=[1.2450000047683716, 1.2450000047683716], "Max"=1048576}, "System"={"Out Type"=0, "Inverse"=0, "Monitor"=0, "Reserve"=0, "ACC Time"=0, "Pulse Rev"=0, "Stroke"=0, "Auto Off"=0, "Gear Ratio"=0.0, "Pitch"=0.0, "Max Speed"=0, "Jog Speed"=0, "Disp Coff"=0.0, "Max Load"=0}, "Index"=enum."Ch1", "Datalog"=enum."Empty"}, "UDP Event Ref"=refnum, "UDP ref"=refnum, "Read Sensor"=0}, "UDP Event Ref"=w394) -> (w398:T6)
          }
          frame "Idle" {
            n126 = Unbundle By Name(w413) -> ("UDP Event Ref"=w417:refnum<event-registration>)
            n127 = event shown="[0] Timeout" {
              selector: w417 -> [_ _]
              dyn-events: _ -> [_ _]
              timeout: 3000 -> [_ _]
              tunnel: [w423 w426] -> w411
              tunnel: [w420 _] -> w416
              tunnel: w415 -> [w420 _]
              tunnel: [w418 w435] -> w414
              tunnel: w413 -> [w418 w434]
              tunnel: w408 -> [_ w424]
              event Timeout {
                n128 = event-data() -> ()  [unwired: 1 in, 1 out]
                n129 = local read "Stop"() -> (w422:bool)
                n130 = Select(t=Communications_-_State."Close", s=w422, f=Communications_-_State."Idle") -> (s? t:f=w423:T2)
              }
              event User Event {
                n131 = event-data() -> ("IP"=w429:string, "CMD"=w433:T1, "Data"=w432:T7)  [unwired: 1 in]
                n132 = global read "Global - IP Address.vi" "IP"() -> (w431:string[])
                n133 = Index Array(array=w431, index=w424) -> (element=w430:string)
                n134 = Equal?(x=w430, y=w429) -> (x = y?=w428:bool)
                n135 = Bundle By Name(cluster=w434, "UDP CMD.IP"=w429, "UDP CMD.CMD"=w433, "Data"=w432) -> (w435:T6)
                n136 = Select(t=Communications_-_State."Command" ("f"), s=w428, f=Communications_-_State."Idle") -> (s? t:f=w426:T2)
              }
            }
            n137 = global read "Global - Hold.vi" "Hold"() -> (w412:bool)
            n138 = Select(t=Communications_-_State."Idle", s=w412, f=w411) -> (s? t:f=w405:T2)
            n139 = local read "Stop"() -> (w406:bool)
            n140 = Select(t=Communications_-_State."Close", s=w406, f=w405) -> (s? t:f=w404:T2)
          }
          frame "Command" {
            n141 = Unbundle By Name(w453) -> ("UDP CMD.CMD"=w450:T1, "Data"=w452:T7, "UDP CMD.IP"=w436:string)
            "4" <- w450
            n142 = global read "Global - Handle V1.vi" "Handle"() -> (w444:refnum<visa-resource-name>[])
            n143 = global read "Global - IP Address.vi" "IP"() -> (w445:string[])
            n144 = Search 1D Array(1D array=w445, element=w436) -> ()  [unwired: 1 in, 1 out]
            n145 = Index Array(array=w444, index=w440) -> (element=w446:refnum<visa-resource-name>)
            n146 = call "VISA - Write CMD.vi"("Index"=w440, "error in"=w454, "Data"=w452, "Action"=w450, "VISA ref"=w446) -> ("error out"=w442:errorcluster, "Data Unit"=w448:T12, "Data Channel"=w449:T13, "Success"=w447:bool, "Prev Data?"=→"Prev 4":bool)  [unwired: 2 out]
            "Success4" <- w447
            n147 = flat-sequence {
              tunnel: w440 -> [w460]
              tunnel: [w457] -> w443
              tunnel: w442 -> [w457]
              frame #0 {
                n148 = global read "Global - Done.vi" "Done"() -> (w459:bool[])
                n149 = Replace Array Subset(array=w459, new element=TRUE, index=w460) -> (w458:bool[])
                n150 = global write "Global - Done.vi" "Done"(w458) -> ()
              }
            }
            n151 = global write "Global - Data UDP.vi" "Loop 5"(TRUE ("Loop 1")) -> ()
            n152 = case shown="False" w447 {
              tunnel: w443 -> [w464 w479]
              tunnel: [w465 w478] -> w451
              tunnel: w450 -> [_ w480]
              tunnel: w449 -> [_ w477]
              tunnel: w448 -> [_ w476]
              tunnel: w440 -> [_ w475]
              tunnel: [w461 0 ("index")] -> w439
              tunnel: w438 -> [w466 _]
              tunnel: w436 -> [w462 _]
              frame False {
                n153 = Increment(x=w466) -> (x+1=w463:i32)
                n154 = case shown="5" w463 {
                  selector: w463 -> [w467 _]
                  tunnel: [w468 w473] -> w465
                  tunnel: w464 -> [w468 w472]
                  tunnel: w462 -> [_ w470]
                  tunnel: [w467 0] -> w461
                  frame 0, Default {
                  }
                  frame 5 {
                    n155 = call "Communication - Reconnect eFGV.vi"("eFGV States"=eFGV_States."Write", "error in (no error)"=w472, "Reconnect In"=w470) -> ("error out"=w473:errorcluster)  [unwired: 6 in, 2 out]
                  }
                }
              }
              frame True {
                n156 = case shown="\"Read Ch Data\"" w480 {
                  tunnel: w479 -> [w481 w488 w503]
                  tunnel: [w481 w488 w503] -> w478
                  tunnel: w477 -> [_ w486 _]
                  tunnel: w476 -> [_ _ w499]
                  tunnel: w475 -> [_ w490 w504]
                  frame "Stop", Default {
                  }
                  frame "Read Ch Data" {
                    n157 = Unbundle By Name(w486) -> ("Ch1 Data"=w485:sgl, "Ch2 Data"=w484:sgl)
                    n158 = global read "Global - Channel.vi" "Data"() -> (w489:T14)
                    n159 = Bundle By Name(cluster=T10 {"Channels"={"Ch1"=0.0, "Ch2"=0.0, "Ch3"=0.0, "Ch4"=0.0, "Ch5"=0.0, "Ch6"=0.0, "Ch7"=0.0, "Ch8"=0.0, "Ch9"=0.0, "Ch10"=0.0, "Ch11"=0.0, "Ch12"=0.0, "Ch13"=0.0, "Ch14"=0.0, "Ch15"=0.0, "Ch16"=0.0}, "Event"=0, "Status"=0, "IP"=""} ("Data Channel"), "Channels.Ch1"=w485, "Channels.Ch2"=w484) -> (w483:T10)
                    n160 = Replace Array Subset(array=w489, new element=w483, index=w490) -> (w487:T14)
                    n161 = global write "Global - Channel.vi" "Data"(w487) -> ()
                  }
                  frame "Read Sensor" {
                    n162 = Unbundle By Name(w499) -> ("Ch1 Unit"=w498:string, "Ch2 Unit"=w497:string, "Ch1 Decimal"=w496:u8, "Ch2 Decimal"=w495:u8)
                    n163 = global read "Global - Unit.vi" "Unit"() -> (w501:T15)
                    n164 = Build Array(w498, w497) -> (w494:string[])
                    n165 = Build Array(w496, w495) -> (w493:u8[])
                    n166 = Bundle By Name(cluster=T11 {"Name"=[], "Unit"=[], "Decimal Point"=[], "Ch Log"=[], "H Alarm"=[], "L Alarm"=[], "H Limit"=[], "L Limit"=[], "Filter"=[], "Gain"=[], "Calib Type"=[]} ("Sensor"), "Name"=string[] ["Load", "Displacement"], "Unit"=w494, "Decimal Point"=w493) -> (w492:T11)
                    n167 = Replace Array Subset(array=w501, new element=w492, index=w504) -> (w502:T15)
                    n168 = global write "Global - Unit.vi" "Unit"(w502) -> ()
                  }
                }
              }
            }
          }
          frame "Close" {
            n169 = global read "Global - Handle V1.vi" "Handle"() -> (w509:refnum<visa-resource-name>[])
            n170 = Index Array(array=w509, index=w508) -> (element=w507:refnum<visa-resource-name>)
            n171 = VISA Close(VISA resource name=w507, error in (no error)=w510) -> (error out=w511:errorcluster)
            n172 = call <vilib>:"Clear Errors.vi"("error in (no error)"=w511) -> ("error out"=w506:errorcluster)  [unwired: 5 in, 1 out]
          }
        }
      }
      frame Error {
        n173 = global read "Global - IP Address.vi" "IP"() -> (w524:string[])
        n174 = Unbundle By Name(w525) -> ("source"=w521:string)
        n175 = Index Array(array=w524, index=w516) -> (element=w523:string)
        n176 = Concatenate Strings(w523, " - " ("string"), w521) -> (w517:string)
        n177 = call <vilib>:"Clear Errors.vi"("error in (no error)"=w525) -> ("error out"=w520:errorcluster)  [unwired: 5 in, 1 out]
        n178 = call "General - Error Log eFGV.vi"("eFGV States"=eFGV_States."Write", "error in (no error)"=w520, "Error In"=w517) -> ("error out"=w519:errorcluster)  [unwired: 6 in, 2 out]
        n179 = Wait (ms)(milliseconds to wait=u32 100) -> ()  [unwired: 1 out]
      }
    }
    "5" <- w380
    "loop 4" <- w374
  }
  n180 = while {
    shift-right: [w538] -> _
    shift-left: errorcluster {"status"=FALSE, "code"=0, "source"=""} ("error IO") -> [w539]
    shift-right: [w536] -> _
    shift-left: Communications_-_State."Init" -> [w537]
    shift-right: [w534] -> _
    shift-left: _ -> [w533]
    tunnel: 6 ("index") -> [w532]
    shift-right: [w530] -> _
    shift-left: _ -> [w529]
    i -> [w531]
    stop <- w535 stop-if-true
    # "Queue Command Processing Loop"
    n181 = case shown="No Error" w539 {
      selector: w539 -> [w548 w681]
      tunnel: [w549 w675] -> w538
      tunnel: w537 -> [w547 _]
      tunnel: [w546 Communications_-_State."Idle"] -> w536
      tunnel: [w545 _] -> w535
      tunnel: [w544 w683] -> w534
      tunnel: w533 -> [w543 w683]
      tunnel: w532 -> [w542 w672]
      tunnel: [w541 w671] -> w530
      tunnel: w529 -> [w540 w671]
      frame No Error {
        n182 = case shown="\"Command\"" w547 {
          tunnel: [w553 w573 w608 w665] -> w549
          tunnel: w548 -> [w558 w572 w611 w664]
          tunnel: [Communications_-_State."Idle" w561 Communications_-_State."Idle" Communications_-_State."Close"] -> w546
          tunnel: [_ _ _ TRUE] -> w545
          tunnel: [w555 w571 w610 w668] -> w544
          tunnel: w543 -> [_ w570 w610 w668]
          tunnel: w542 -> [_ w565 w597 w663]
          tunnel: [0 w560 w595 0] -> w541
          tunnel: w540 -> [_ w560 w594 _]
          frame "Init", Default {
            n183 = call "Communication - UDP Command (eFGV).vi"("Action"=eFGV_States."Read", "error in"=w558) -> ("error out"=w554:errorcluster, "UDP Ref"=w552:refnum<user-event>)  [unwired: 7 in, 1 out]
            n184 = register-events(error in=w554, w552) -> (reference out=w551:refnum<event-registration>, error out=w553:errorcluster)  [unwired: 1 in]
            n185 = Bundle By Name(cluster=T6 {"UDP CMD"={"IP"="", "CMD"=enum."Stop", "Port"="", "Datalog?"=FALSE, "Float"=0.0}, "Unit?"=FALSE, "Read Unit"=[], "Trig?"=FALSE, "UDP Info"=[], "DataLogger"=[], "VISA Ref"=refnum, "Float"=0.0, "Data"={"Test"={"Target Load"=0.0, "Target Disp"=0.0, "Rate"=0.0, "Speed"=0.0}, "Sensor"={"Name"=[], "Unit"=[], "Decimal Point"=[], "Ch Log"=[], "H Alarm"=[], "L Alarm"=[], "H Limit"=[], "L Limit"=[], "Filter"=[], "Gain"=[], "Calib Type"=[]}, "PID"={"SP"=-2.7823365e-08, "PV"=-3.023652e-13, "kP"=8.5432666e-24, "kI"=2.29252e-41, "kD"=1.570387e-38, "FF"=25.0, "Err Band"=0.0, "Max"=15, "Min"=-7, "Ts"=1886611780, "Out"=0, "Mode"=0}, "ADC"={"Active Ch"=[255, 255, 255, 0, 0, 0, 0, 0], "Filter Type"=2, "Post Filter"=[1, 1, 1, 1, 0, 200, 66, 184], "Gain"=[0, 0, 0, 0, 0, 122, 68, 0], "FS"=32, "IntOC"=0, "IntFC"=255, "SysOC"=255, "Cofficient"=[1.0, 1.0, 1.0, 1.0, 1.0, 1.0, 1.0, 1.0], "K"=[1.2450000047683716, 1.2450000047683716], "Max"=1048576}, "System"={"Out Type"=0, "Inverse"=0, "Monitor"=0, "Reserve"=0, "ACC Time"=0, "Pulse Rev"=0, "Stroke"=0, "Auto Off"=0, "Gear Ratio"=0.0, "Pitch"=0.0, "Max Speed"=0, "Jog Speed"=0, "Disp Coff"=0.0, "Max Load"=0}, "Index"=enum."Ch1", "Datalog"=enum."Empty"}, "UDP Event Ref"=refnum, "UDP ref"=refnum, "Read Sensor"=0}, "UDP Event Ref"=w551) -> (w555:T6)
          }
          frame "Idle" {
            n186 = Unbundle By Name(w570) -> ("UDP Event Ref"=w574:refnum<event-registration>)
            n187 = event shown="[0] Timeout" {
              selector: w574 -> [_ _]
              dyn-events: _ -> [_ _]
              timeout: 3000 -> [_ _]
              tunnel: [w580 w583] -> w568
              tunnel: [w577 _] -> w573
              tunnel: w572 -> [w577 _]
              tunnel: [w575 w592] -> w571
              tunnel: w570 -> [w575 w591]
              tunnel: w565 -> [_ w581]
              event Timeout {
                n188 = event-data() -> ()  [unwired: 1 in, 1 out]
                n189 = local read "Stop"() -> (w579:bool)
                n190 = Select(t=Communications_-_State."Close", s=w579, f=Communications_-_State."Idle") -> (s? t:f=w580:T2)
              }
              event User Event {
                n191 = event-data() -> ("IP"=w586:string, "CMD"=w590:T1, "Data"=w589:T7)  [unwired: 1 in]
                n192 = global read "Global - IP Address.vi" "IP"() -> (w588:string[])
                n193 = Index Array(array=w588, index=w581) -> (element=w587:string)
                n194 = Equal?(x=w587, y=w586) -> (x = y?=w585:bool)
                n195 = Bundle By Name(cluster=w591, "UDP CMD.IP"=w586, "UDP CMD.CMD"=w590, "Data"=w589) -> (w592:T6)
                n196 = Select(t=Communications_-_State."Command" ("f"), s=w585, f=Communications_-_State."Idle") -> (s? t:f=w583:T2)
              }
            }
            n197 = global read "Global - Hold.vi" "Hold"() -> (w569:bool)
            n198 = Select(t=Communications_-_State."Idle", s=w569, f=w568) -> (s? t:f=w562:T2)
            n199 = local read "Stop"() -> (w563:bool)
            n200 = Select(t=Communications_-_State."Close", s=w563, f=w562) -> (s? t:f=w561:T2)
          }
          frame "Command" {
            n201 = Unbundle By Name(w610) -> ("UDP CMD.CMD"=w607:T1, "Data"=w609:T7, "UDP CMD.IP"=w593:string)
            "6" <- w607
            n202 = global read "Global - Handle V1.vi" "Handle"() -> (w601:refnum<visa-resource-name>[])
            n203 = global read "Global - IP Address.vi" "IP"() -> (w602:string[])
            n204 = Search 1D Array(1D array=w602, element=w593) -> ()  [unwired: 1 in, 1 out]
            n205 = Index Array(array=w601, index=w597) -> (element=w603:refnum<visa-resource-name>)
            n206 = call "VISA - Write CMD.vi"("Index"=w597, "error in"=w611, "Data"=w609, "Action"=w607, "VISA ref"=w603) -> ("error out"=w599:errorcluster, "Data Unit"=w605:T12, "Data Channel"=w606:T13, "Success"=w604:bool, "Prev Data?"=→"Prev 6":bool)  [unwired: 2 out]
            "Success6" <- w604
            n207 = flat-sequence {
              tunnel: w597 -> [w617]
              tunnel: [w614] -> w600
              tunnel: w599 -> [w614]
              frame #0 {
                n208 = global read "Global - Done.vi" "Done"() -> (w616:bool[])
                n209 = Replace Array Subset(array=w616, new element=TRUE, index=w617) -> (w615:bool[])
                n210 = global write "Global - Done.vi" "Done"(w615) -> ()
              }
            }
            n211 = global write "Global - Data UDP.vi" "Loop 7"(TRUE ("Loop 3")) -> ()
            n212 = case shown="False" w604 {
              tunnel: w600 -> [w621 w636]
              tunnel: [w622 w635] -> w608
              tunnel: w607 -> [_ w637]
              tunnel: w606 -> [_ w634]
              tunnel: w605 -> [_ w633]
              tunnel: w597 -> [_ w632]
              tunnel: [w618 0] -> w595
              tunnel: w594 -> [w623 _]
              tunnel: w593 -> [w620 _]
              frame False {
                n213 = Increment(x=w623) -> (x+1=w619:i32)
                n214 = case shown="5" w619 {
                  selector: w619 -> [w624 _]
                  tunnel: [w625 w629] -> w622
                  tunnel: w621 -> [w625 w628]
                  tunnel: w620 -> [_ w627]
                  tunnel: [w624 0] -> w618
                  frame 0, Default {
                  }
                  frame 5 {
                    n215 = call "Communication - Reconnect eFGV.vi"("eFGV States"=eFGV_States."Write", "error in (no error)"=w628, "Reconnect In"=w627) -> ("error out"=w629:errorcluster)  [unwired: 6 in, 2 out]
                  }
                }
              }
              frame True {
                n216 = case shown="\"Read Sensor\"" w637 {
                  tunnel: w636 -> [w638 w645 w660]
                  tunnel: [w638 w645 w660] -> w635
                  tunnel: w634 -> [_ w643 _]
                  tunnel: w633 -> [_ _ w656]
                  tunnel: w632 -> [_ w647 w661]
                  frame "Stop", Default {
                  }
                  frame "Read Ch Data" {
                    n217 = Unbundle By Name(w643) -> ("Ch1 Data"=w642:sgl, "Ch2 Data"=w641:sgl)
                    n218 = global read "Global - Channel.vi" "Data"() -> (w646:T14)
                    n219 = Bundle By Name(cluster=T10 {"Channels"={"Ch1"=0.0, "Ch2"=0.0, "Ch3"=0.0, "Ch4"=0.0, "Ch5"=0.0, "Ch6"=0.0, "Ch7"=0.0, "Ch8"=0.0, "Ch9"=0.0, "Ch10"=0.0, "Ch11"=0.0, "Ch12"=0.0, "Ch13"=0.0, "Ch14"=0.0, "Ch15"=0.0, "Ch16"=0.0}, "Event"=0, "Status"=0, "IP"=""} ("Data Channel"), "Channels.Ch1"=w642, "Channels.Ch2"=w641) -> (w640:T10)
                    n220 = Replace Array Subset(array=w646, new element=w640, index=w647) -> (w644:T14)
                    n221 = global write "Global - Channel.vi" "Data"(w644) -> ()
                  }
                  frame "Read Sensor" {
                    n222 = Unbundle By Name(w656) -> ("Ch1 Unit"=w655:string, "Ch2 Unit"=w654:string, "Ch1 Decimal"=w653:u8, "Ch2 Decimal"=w652:u8)
                    n223 = global read "Global - Unit.vi" "Unit"() -> (w658:T15)
                    n224 = Build Array(w655, w654) -> (w651:string[])
                    n225 = Build Array(w653, w652) -> (w650:u8[])
                    n226 = Bundle By Name(cluster=T11 {"Name"=[], "Unit"=[], "Decimal Point"=[], "Ch Log"=[], "H Alarm"=[], "L Alarm"=[], "H Limit"=[], "L Limit"=[], "Filter"=[], "Gain"=[], "Calib Type"=[]} ("Sensor"), "Name"=string[] ["Load", "Displacement"], "Unit"=w651, "Decimal Point"=w650) -> (w649:T11)
                    n227 = Replace Array Subset(array=w658, new element=w649, index=w661) -> (w659:T15)
                    n228 = global write "Global - Unit.vi" "Unit"(w659) -> ()
                  }
                }
              }
            }
          }
          frame "Close" {
            n229 = global read "Global - Handle V1.vi" "Handle"() -> (w667:refnum<visa-resource-name>[])
            n230 = Index Array(array=w667, index=w663) -> (element=w666:refnum<visa-resource-name>)
            n231 = VISA Close(VISA resource name=w666, error in (no error)=w664) -> (error out=w665:errorcluster)
          }
        }
      }
      frame Error {
        n232 = global read "Global - IP Address.vi" "IP"() -> (w680:string[])
        n233 = Unbundle By Name(w681) -> ("source"=w677:string)
        n234 = Index Array(array=w680, index=w672) -> (element=w679:string)
        n235 = Concatenate Strings(w679, " - " ("string"), w677) -> (w673:string)
        n236 = call <vilib>:"Clear Errors.vi"("error in (no error)"=w681) -> ("error out"=w676:errorcluster)  [unwired: 5 in, 1 out]
        n237 = call "General - Error Log eFGV.vi"("eFGV States"=eFGV_States."Write", "error in (no error)"=w676, "Error In"=w673) -> ("error out"=w675:errorcluster)  [unwired: 6 in, 2 out]
        n238 = Wait (ms)(milliseconds to wait=u32 100) -> ()  [unwired: 1 out]
      }
    }
    "6" <- w537
    "loop 6" <- w531
  }
  n239 = while {
    shift-right: [w694] -> _
    shift-left: errorcluster {"status"=FALSE, "code"=0, "source"=""} ("error IO") -> [w695]
    shift-right: [w692] -> _
    shift-left: Communications_-_State."Init" -> [w693]
    shift-right: [w690] -> _
    shift-left: _ -> [w689]
    tunnel: 8 ("index") -> [w688]
    shift-right: [w686] -> _
    shift-left: _ -> [w685]
    i -> [w687]
    stop <- w691 stop-if-true
    # "Queue Command Processing Loop"
    n240 = case shown="No Error" w695 {
      selector: w695 -> [w704 w838]
      tunnel: [w705 w832] -> w694
      tunnel: w693 -> [w703 _]
      tunnel: [w702 Communications_-_State."Idle"] -> w692
      tunnel: [w701 _] -> w691
      tunnel: [w700 w840] -> w690
      tunnel: w689 -> [w699 w840]
      tunnel: w688 -> [w698 w829]
      tunnel: [w697 w828] -> w686
      tunnel: w685 -> [w696 w828]
      frame No Error {
        n241 = case shown="\"Command\"" w703 {
          tunnel: [w709 w729 w764 w819] -> w705
          tunnel: w704 -> [w714 w728 w767 w823]
          tunnel: [Communications_-_State."Idle" w717 Communications_-_State."Idle" Communications_-_State."Close"] -> w702
          tunnel: [_ _ _ TRUE] -> w701
          tunnel: [w711 w727 w766 w825] -> w700
          tunnel: w699 -> [_ w726 w766 w825]
          tunnel: w698 -> [_ w721 w753 w821]
          tunnel: [0 ("index") w716 w752 0 ("index")] -> w697
          tunnel: w696 -> [_ w716 w751 _]
          frame "Init", Default {
            n242 = call "Communication - UDP Command (eFGV).vi"("Action"=eFGV_States."Read", "error in"=w714) -> ("error out"=w710:errorcluster, "UDP Ref"=w708:refnum<user-event>)  [unwired: 7 in, 1 out]
            n243 = register-events(error in=w710, w708) -> (reference out=w707:refnum<event-registration>, error out=w709:errorcluster)  [unwired: 1 in]
            n244 = Bundle By Name(cluster=T6 {"UDP CMD"={"IP"="", "CMD"=enum."Stop", "Port"="", "Datalog?"=FALSE, "Float"=0.0}, "Unit?"=FALSE, "Read Unit"=[], "Trig?"=FALSE, "UDP Info"=[], "DataLogger"=[], "VISA Ref"=refnum, "Float"=0.0, "Data"={"Test"={"Target Load"=0.0, "Target Disp"=0.0, "Rate"=0.0, "Speed"=0.0}, "Sensor"={"Name"=[], "Unit"=[], "Decimal Point"=[], "Ch Log"=[], "H Alarm"=[], "L Alarm"=[], "H Limit"=[], "L Limit"=[], "Filter"=[], "Gain"=[], "Calib Type"=[]}, "PID"={"SP"=-2.7823365e-08, "PV"=-3.023652e-13, "kP"=8.5432666e-24, "kI"=2.29252e-41, "kD"=1.570387e-38, "FF"=25.0, "Err Band"=0.0, "Max"=15, "Min"=-7, "Ts"=1886611780, "Out"=0, "Mode"=0}, "ADC"={"Active Ch"=[255, 255, 255, 0, 0, 0, 0, 0], "Filter Type"=2, "Post Filter"=[1, 1, 1, 1, 0, 200, 66, 184], "Gain"=[0, 0, 0, 0, 0, 122, 68, 0], "FS"=32, "IntOC"=0, "IntFC"=255, "SysOC"=255, "Cofficient"=[1.0, 1.0, 1.0, 1.0, 1.0, 1.0, 1.0, 1.0], "K"=[1.2450000047683716, 1.2450000047683716], "Max"=1048576}, "System"={"Out Type"=0, "Inverse"=0, "Monitor"=0, "Reserve"=0, "ACC Time"=0, "Pulse Rev"=0, "Stroke"=0, "Auto Off"=0, "Gear Ratio"=0.0, "Pitch"=0.0, "Max Speed"=0, "Jog Speed"=0, "Disp Coff"=0.0, "Max Load"=0}, "Index"=enum."Ch1", "Datalog"=enum."Empty"}, "UDP Event Ref"=refnum, "UDP ref"=refnum, "Read Sensor"=0}, "UDP Event Ref"=w707) -> (w711:T6)
          }
          frame "Idle" {
            n245 = Unbundle By Name(w726) -> ("UDP Event Ref"=w730:refnum<event-registration>)
            n246 = event shown="[0] Timeout" {
              selector: w730 -> [_ _]
              dyn-events: _ -> [_ _]
              timeout: 3000 -> [_ _]
              tunnel: [w736 w739] -> w724
              tunnel: [w733 _] -> w729
              tunnel: w728 -> [w733 _]
              tunnel: [w731 w748] -> w727
              tunnel: w726 -> [w731 w747]
              tunnel: w721 -> [_ w737]
              event Timeout {
                n247 = event-data() -> ()  [unwired: 1 in, 1 out]
                n248 = local read "Stop"() -> (w735:bool)
                n249 = Select(t=Communications_-_State."Close", s=w735, f=Communications_-_State."Idle") -> (s? t:f=w736:T2)
              }
              event User Event {
                n250 = event-data() -> ("IP"=w742:string, "CMD"=w746:T1, "Data"=w745:T7)  [unwired: 1 in]
                n251 = global read "Global - IP Address.vi" "IP"() -> (w744:string[])
                n252 = Index Array(array=w744, index=w737) -> (element=w743:string)
                n253 = Equal?(x=w743, y=w742) -> (x = y?=w741:bool)
                n254 = Bundle By Name(cluster=w747, "UDP CMD.IP"=w742, "UDP CMD.CMD"=w746, "Data"=w745) -> (w748:T6)
                n255 = Select(t=Communications_-_State."Command" ("f"), s=w741, f=Communications_-_State."Idle") -> (s? t:f=w739:T2)
              }
            }
            n256 = global read "Global - Hold.vi" "Hold"() -> (w725:bool)
            n257 = Select(t=Communications_-_State."Idle", s=w725, f=w724) -> (s? t:f=w718:T2)
            n258 = local read "Stop"() -> (w719:bool)
            n259 = Select(t=Communications_-_State."Close", s=w719, f=w718) -> (s? t:f=w717:T2)
          }
          frame "Command" {
            n260 = Unbundle By Name(w766) -> ("UDP CMD.CMD"=w763:T1, "Data"=w765:T7, "UDP CMD.IP"=w749:string)
            "8" <- w763
            n261 = global read "Global - Handle V1.vi" "Handle"() -> (w757:refnum<visa-resource-name>[])
            n262 = global read "Global - IP Address.vi" "IP"() -> (w758:string[])
            n263 = Search 1D Array(1D array=w758, element=w749) -> ()  [unwired: 1 in, 1 out]
            n264 = Index Array(array=w757, index=w753) -> (element=w759:refnum<visa-resource-name>)
            n265 = call "VISA - Write CMD.vi"("Index"=w753, "error in"=w767, "Data"=w765, "Action"=w763, "VISA ref"=w759) -> ("error out"=w755:errorcluster, "Data Unit"=w761:T12, "Data Channel"=w762:T13, "Success"=w760:bool, "Prev Data?"=→"Prev 8":bool)  [unwired: 2 out]
            "Success8" <- w760
            n266 = flat-sequence {
              tunnel: w753 -> [w773]
              tunnel: [w770] -> w756
              tunnel: w755 -> [w770]
              frame #0 {
                n267 = global read "Global - Done.vi" "Done"() -> (w772:bool[])
                n268 = Replace Array Subset(array=w772, new element=TRUE, index=w773) -> (w771:bool[])
                n269 = global write "Global - Done.vi" "Done"(w771) -> ()
              }
            }
            n270 = global write "Global - Data UDP.vi" "Loop 9"(TRUE ("Loop 1")) -> ()
            n271 = case shown="False" w760 {
              tunnel: w756 -> [w777 w792]
              tunnel: [w778 w791] -> w764
              tunnel: w763 -> [_ w793]
              tunnel: w762 -> [_ w790]
              tunnel: w761 -> [_ w789]
              tunnel: w753 -> [_ w788]
              tunnel: [w774 0 ("index")] -> w752
              tunnel: w751 -> [w779 _]
              tunnel: w749 -> [w775 _]
              frame False {
                n272 = Increment(x=w779) -> (x+1=w776:i32)
                n273 = case shown="0, Default" w776 {
                  selector: w776 -> [w780 _]
                  tunnel: [w781 w786] -> w778
                  tunnel: w777 -> [w781 w785]
                  tunnel: w775 -> [_ w783]
                  tunnel: [w780 0] -> w774
                  frame 0, Default {
                  }
                  frame 5 {
                    n274 = call "Communication - Reconnect eFGV.vi"("eFGV States"=eFGV_States."Write", "error in (no error)"=w785, "Reconnect In"=w783) -> ("error out"=w786:errorcluster)  [unwired: 6 in, 2 out]
                  }
                }
              }
              frame True {
                n275 = case shown="\"Read Ch Data\"" w793 {
                  tunnel: w792 -> [w794 w801 w816]
                  tunnel: [w794 w801 w816] -> w791
                  tunnel: w790 -> [_ w799 _]
                  tunnel: w789 -> [_ _ w812]
                  tunnel: w788 -> [_ w803 w817]
                  frame "Stop", Default {
                  }
                  frame "Read Ch Data" {
                    n276 = Unbundle By Name(w799) -> ("Ch1 Data"=w798:sgl, "Ch2 Data"=w797:sgl)
                    n277 = global read "Global - Channel.vi" "Data"() -> (w802:T14)
                    n278 = Bundle By Name(cluster=T10 {"Channels"={"Ch1"=0.0, "Ch2"=0.0, "Ch3"=0.0, "Ch4"=0.0, "Ch5"=0.0, "Ch6"=0.0, "Ch7"=0.0, "Ch8"=0.0, "Ch9"=0.0, "Ch10"=0.0, "Ch11"=0.0, "Ch12"=0.0, "Ch13"=0.0, "Ch14"=0.0, "Ch15"=0.0, "Ch16"=0.0}, "Event"=0, "Status"=0, "IP"=""} ("Data Channel"), "Channels.Ch1"=w798, "Channels.Ch2"=w797) -> (w796:T10)
                    n279 = Replace Array Subset(array=w802, new element=w796, index=w803) -> (w800:T14)
                    n280 = global write "Global - Channel.vi" "Data"(w800) -> ()
                  }
                  frame "Read Sensor" {
                    n281 = Unbundle By Name(w812) -> ("Ch1 Unit"=w811:string, "Ch2 Unit"=w810:string, "Ch1 Decimal"=w809:u8, "Ch2 Decimal"=w808:u8)
                    n282 = global read "Global - Unit.vi" "Unit"() -> (w814:T15)
                    n283 = Build Array(w811, w810) -> (w807:string[])
                    n284 = Build Array(w809, w808) -> (w806:u8[])
                    n285 = Bundle By Name(cluster=T11 {"Name"=[], "Unit"=[], "Decimal Point"=[], "Ch Log"=[], "H Alarm"=[], "L Alarm"=[], "H Limit"=[], "L Limit"=[], "Filter"=[], "Gain"=[], "Calib Type"=[]} ("Sensor"), "Name"=string[] ["Load", "Displacement"], "Unit"=w807, "Decimal Point"=w806) -> (w805:T11)
                    n286 = Replace Array Subset(array=w814, new element=w805, index=w817) -> (w815:T15)
                    n287 = global write "Global - Unit.vi" "Unit"(w815) -> ()
                  }
                }
              }
            }
          }
          frame "Close" {
            n288 = global read "Global - Handle V1.vi" "Handle"() -> (w822:refnum<visa-resource-name>[])
            n289 = Index Array(array=w822, index=w821) -> (element=w820:refnum<visa-resource-name>)
            n290 = VISA Close(VISA resource name=w820, error in (no error)=w823) -> (error out=w824:errorcluster)
            n291 = call <vilib>:"Clear Errors.vi"("error in (no error)"=w824) -> ("error out"=w819:errorcluster)  [unwired: 5 in, 1 out]
          }
        }
      }
      frame Error {
        n292 = global read "Global - IP Address.vi" "IP"() -> (w837:string[])
        n293 = Unbundle By Name(w838) -> ("source"=w834:string)
        n294 = Index Array(array=w837, index=w829) -> (element=w836:string)
        n295 = Concatenate Strings(w836, " - " ("string"), w834) -> (w830:string)
        n296 = call <vilib>:"Clear Errors.vi"("error in (no error)"=w838) -> ("error out"=w833:errorcluster)  [unwired: 5 in, 1 out]
        n297 = call "General - Error Log eFGV.vi"("eFGV States"=eFGV_States."Write", "error in (no error)"=w833, "Error In"=w830) -> ("error out"=w832:errorcluster)  [unwired: 6 in, 2 out]
        n298 = Wait (ms)(milliseconds to wait=u32 100) -> ()  [unwired: 1 out]
      }
    }
    "8" <- w693
    "loop 8" <- w687
  }
  n299 = while {
    shift-right: [w851] -> _
    shift-left: errorcluster {"status"=FALSE, "code"=0, "source"=""} ("error IO") -> [w852]
    shift-right: [w849] -> _
    shift-left: Communications_-_State."Init" -> [w850]
    shift-right: [w847] -> _
    shift-left: _ -> [w846]
    tunnel: 10 ("index") -> [w845]
    shift-right: [w843] -> _
    shift-left: _ -> [w842]
    i -> [w844]
    stop <- w848 stop-if-true
    # "Queue Command Processing Loop"
    n300 = case shown="No Error" w852 {
      selector: w852 -> [w861 w994]
      tunnel: [w862 w988] -> w851
      tunnel: w850 -> [w860 _]
      tunnel: [w859 Communications_-_State."Idle"] -> w849
      tunnel: [w858 _] -> w848
      tunnel: [w857 w996] -> w847
      tunnel: w846 -> [w856 w996]
      tunnel: w845 -> [w855 w985]
      tunnel: [w854 w984] -> w843
      tunnel: w842 -> [w853 w984]
      frame No Error {
        n301 = case shown="\"Command\"" w860 {
          tunnel: [w866 w886 w921 w978] -> w862
          tunnel: w861 -> [w871 w885 w924 w977]
          tunnel: [Communications_-_State."Idle" w874 Communications_-_State."Idle" Communications_-_State."Close"] -> w859
          tunnel: [_ _ _ TRUE] -> w858
          tunnel: [w868 w884 w923 w981] -> w857
          tunnel: w856 -> [_ w883 w923 w981]
          tunnel: w855 -> [_ w878 w910 w976]
          tunnel: [0 w873 w908 0] -> w854
          tunnel: w853 -> [_ w873 w907 _]
          frame "Init", Default {
            n302 = call "Communication - UDP Command (eFGV).vi"("Action"=eFGV_States."Read", "error in"=w871) -> ("error out"=w867:errorcluster, "UDP Ref"=w865:refnum<user-event>)  [unwired: 7 in, 1 out]
            n303 = register-events(error in=w867, w865) -> (reference out=w864:refnum<event-registration>, error out=w866:errorcluster)  [unwired: 1 in]
            n304 = Bundle By Name(cluster=T6 {"UDP CMD"={"IP"="", "CMD"=enum."Stop", "Port"="", "Datalog?"=FALSE, "Float"=0.0}, "Unit?"=FALSE, "Read Unit"=[], "Trig?"=FALSE, "UDP Info"=[], "DataLogger"=[], "VISA Ref"=refnum, "Float"=0.0, "Data"={"Test"={"Target Load"=0.0, "Target Disp"=0.0, "Rate"=0.0, "Speed"=0.0}, "Sensor"={"Name"=[], "Unit"=[], "Decimal Point"=[], "Ch Log"=[], "H Alarm"=[], "L Alarm"=[], "H Limit"=[], "L Limit"=[], "Filter"=[], "Gain"=[], "Calib Type"=[]}, "PID"={"SP"=-2.7823365e-08, "PV"=-3.023652e-13, "kP"=8.5432666e-24, "kI"=2.29252e-41, "kD"=1.570387e-38, "FF"=25.0, "Err Band"=0.0, "Max"=15, "Min"=-7, "Ts"=1886611780, "Out"=0, "Mode"=0}, "ADC"={"Active Ch"=[255, 255, 255, 0, 0, 0, 0, 0], "Filter Type"=2, "Post Filter"=[1, 1, 1, 1, 0, 200, 66, 184], "Gain"=[0, 0, 0, 0, 0, 122, 68, 0], "FS"=32, "IntOC"=0, "IntFC"=255, "SysOC"=255, "Cofficient"=[1.0, 1.0, 1.0, 1.0, 1.0, 1.0, 1.0, 1.0], "K"=[1.2450000047683716, 1.2450000047683716], "Max"=1048576}, "System"={"Out Type"=0, "Inverse"=0, "Monitor"=0, "Reserve"=0, "ACC Time"=0, "Pulse Rev"=0, "Stroke"=0, "Auto Off"=0, "Gear Ratio"=0.0, "Pitch"=0.0, "Max Speed"=0, "Jog Speed"=0, "Disp Coff"=0.0, "Max Load"=0}, "Index"=enum."Ch1", "Datalog"=enum."Empty"}, "UDP Event Ref"=refnum, "UDP ref"=refnum, "Read Sensor"=0}, "UDP Event Ref"=w864) -> (w868:T6)
          }
          frame "Idle" {
            n305 = Unbundle By Name(w883) -> ("UDP Event Ref"=w887:refnum<event-registration>)
            n306 = event shown="[0] Timeout" {
              selector: w887 -> [_ _]
              dyn-events: _ -> [_ _]
              timeout: 3000 -> [_ _]
              tunnel: [w893 w896] -> w881
              tunnel: [w890 _] -> w886
              tunnel: w885 -> [w890 _]
              tunnel: [w888 w905] -> w884
              tunnel: w883 -> [w888 w904]
              tunnel: w878 -> [_ w894]
              event Timeout {
                n307 = event-data() -> ()  [unwired: 1 in, 1 out]
                n308 = local read "Stop"() -> (w892:bool)
                n309 = Select(t=Communications_-_State."Close", s=w892, f=Communications_-_State."Idle") -> (s? t:f=w893:T2)
              }
              event User Event {
                n310 = event-data() -> ("IP"=w899:string, "CMD"=w903:T1, "Data"=w902:T7)  [unwired: 1 in]
                n311 = global read "Global - IP Address.vi" "IP"() -> (w901:string[])
                n312 = Index Array(array=w901, index=w894) -> (element=w900:string)
                n313 = Equal?(x=w900, y=w899) -> (x = y?=w898:bool)
                n314 = Bundle By Name(cluster=w904, "UDP CMD.IP"=w899, "UDP CMD.CMD"=w903, "Data"=w902) -> (w905:T6)
                n315 = Select(t=Communications_-_State."Command" ("f"), s=w898, f=Communications_-_State."Idle") -> (s? t:f=w896:T2)
              }
            }
            n316 = global read "Global - Hold.vi" "Hold"() -> (w882:bool)
            n317 = Select(t=Communications_-_State."Idle", s=w882, f=w881) -> (s? t:f=w875:T2)
            n318 = local read "Stop"() -> (w876:bool)
            n319 = Select(t=Communications_-_State."Close", s=w876, f=w875) -> (s? t:f=w874:T2)
          }
          frame "Command" {
            n320 = Unbundle By Name(w923) -> ("UDP CMD.CMD"=w920:T1, "Data"=w922:T7, "UDP CMD.IP"=w906:string)
            "10" <- w920
            n321 = global read "Global - Handle V1.vi" "Handle"() -> (w914:refnum<visa-resource-name>[])
            n322 = global read "Global - IP Address.vi" "IP"() -> (w915:string[])
            n323 = Search 1D Array(1D array=w915, element=w906) -> ()  [unwired: 1 in, 1 out]
            n324 = Index Array(array=w914, index=w910) -> (element=w916:refnum<visa-resource-name>)
            n325 = call "VISA - Write CMD.vi"("Index"=w910, "error in"=w924, "Data"=w922, "Action"=w920, "VISA ref"=w916) -> ("error out"=w912:errorcluster, "Data Unit"=w918:T12, "Data Channel"=w919:T13, "Success"=w917:bool, "Prev Data?"=→"Prev 10":bool)  [unwired: 2 out]
            "Success10" <- w917
            n326 = flat-sequence {
              tunnel: w910 -> [w930]
              tunnel: [w927] -> w913
              tunnel: w912 -> [w927]
              frame #0 {
                n327 = global read "Global - Done.vi" "Done"() -> (w929:bool[])
                n328 = Replace Array Subset(array=w929, new element=TRUE, index=w930) -> (w928:bool[])
                n329 = global write "Global - Done.vi" "Done"(w928) -> ()
              }
            }
            n330 = global write "Global - Data UDP.vi" "Loop 11"(TRUE ("Loop 3")) -> ()
            n331 = case shown="False" w917 {
              tunnel: w913 -> [w934 w949]
              tunnel: [w935 w948] -> w921
              tunnel: w920 -> [_ w950]
              tunnel: w919 -> [_ w947]
              tunnel: w918 -> [_ w946]
              tunnel: w910 -> [_ w945]
              tunnel: [w931 0] -> w908
              tunnel: w907 -> [w936 _]
              tunnel: w906 -> [w933 _]
              frame False {
                n332 = Increment(x=w936) -> (x+1=w932:i32)
                n333 = case shown="5" w932 {
                  selector: w932 -> [w937 _]
                  tunnel: [w938 w942] -> w935
                  tunnel: w934 -> [w938 w941]
                  tunnel: w933 -> [_ w940]
                  tunnel: [w937 0] -> w931
                  frame 0, Default {
                  }
                  frame 5 {
                    n334 = call "Communication - Reconnect eFGV.vi"("eFGV States"=eFGV_States."Write", "error in (no error)"=w941, "Reconnect In"=w940) -> ("error out"=w942:errorcluster)  [unwired: 6 in, 2 out]
                  }
                }
              }
              frame True {
                n335 = case shown="\"Read Sensor\"" w950 {
                  tunnel: w949 -> [w951 w958 w973]
                  tunnel: [w951 w958 w973] -> w948
                  tunnel: w947 -> [_ w956 _]
                  tunnel: w946 -> [_ _ w969]
                  tunnel: w945 -> [_ w960 w974]
                  frame "Stop", Default {
                  }
                  frame "Read Ch Data" {
                    n336 = Unbundle By Name(w956) -> ("Ch1 Data"=w955:sgl, "Ch2 Data"=w954:sgl)
                    n337 = global read "Global - Channel.vi" "Data"() -> (w959:T14)
                    n338 = Bundle By Name(cluster=T10 {"Channels"={"Ch1"=0.0, "Ch2"=0.0, "Ch3"=0.0, "Ch4"=0.0, "Ch5"=0.0, "Ch6"=0.0, "Ch7"=0.0, "Ch8"=0.0, "Ch9"=0.0, "Ch10"=0.0, "Ch11"=0.0, "Ch12"=0.0, "Ch13"=0.0, "Ch14"=0.0, "Ch15"=0.0, "Ch16"=0.0}, "Event"=0, "Status"=0, "IP"=""} ("Data Channel"), "Channels.Ch1"=w955, "Channels.Ch2"=w954) -> (w953:T10)
                    n339 = Replace Array Subset(array=w959, new element=w953, index=w960) -> (w957:T14)
                    n340 = global write "Global - Channel.vi" "Data"(w957) -> ()
                  }
                  frame "Read Sensor" {
                    n341 = Unbundle By Name(w969) -> ("Ch1 Unit"=w968:string, "Ch2 Unit"=w967:string, "Ch1 Decimal"=w966:u8, "Ch2 Decimal"=w965:u8)
                    n342 = global read "Global - Unit.vi" "Unit"() -> (w971:T15)
                    n343 = Build Array(w968, w967) -> (w964:string[])
                    n344 = Build Array(w966, w965) -> (w963:u8[])
                    n345 = Bundle By Name(cluster=T11 {"Name"=[], "Unit"=[], "Decimal Point"=[], "Ch Log"=[], "H Alarm"=[], "L Alarm"=[], "H Limit"=[], "L Limit"=[], "Filter"=[], "Gain"=[], "Calib Type"=[]} ("Sensor"), "Name"=string[] ["Load", "Displacement"], "Unit"=w964, "Decimal Point"=w963) -> (w962:T11)
                    n346 = Replace Array Subset(array=w971, new element=w962, index=w974) -> (w972:T15)
                    n347 = global write "Global - Unit.vi" "Unit"(w972) -> ()
                  }
                }
              }
            }
          }
          frame "Close" {
            n348 = global read "Global - Handle V1.vi" "Handle"() -> (w980:refnum<visa-resource-name>[])
            n349 = Index Array(array=w980, index=w976) -> (element=w979:refnum<visa-resource-name>)
            n350 = VISA Close(VISA resource name=w979, error in (no error)=w977) -> (error out=w978:errorcluster)
          }
        }
      }
      frame Error {
        n351 = global read "Global - IP Address.vi" "IP"() -> (w993:string[])
        n352 = Unbundle By Name(w994) -> ("source"=w990:string)
        n353 = Index Array(array=w993, index=w985) -> (element=w992:string)
        n354 = Concatenate Strings(w992, " - " ("string"), w990) -> (w986:string)
        n355 = call <vilib>:"Clear Errors.vi"("error in (no error)"=w994) -> ("error out"=w989:errorcluster)  [unwired: 5 in, 1 out]
        n356 = call "General - Error Log eFGV.vi"("eFGV States"=eFGV_States."Write", "error in (no error)"=w989, "Error In"=w986) -> ("error out"=w988:errorcluster)  [unwired: 6 in, 2 out]
        n357 = Wait (ms)(milliseconds to wait=u32 100) -> ()  [unwired: 1 out]
      }
    }
    "10" <- w850
    "loop 10" <- w844
  }
  n358 = while {
    shift-right: [w1007] -> _
    shift-left: errorcluster {"status"=FALSE, "code"=0, "source"=""} ("error IO") -> [w1008]
    shift-right: [w1005] -> _
    shift-left: Communications_-_State."Init" -> [w1006]
    shift-right: [w1003] -> _
    shift-left: _ -> [w1002]
    tunnel: 12 ("index") -> [w1001]
    shift-right: [w999] -> _
    shift-left: _ -> [w998]
    i -> [w1000]
    stop <- w1004 stop-if-true
    # "Queue Command Processing Loop"
    n359 = case shown="No Error" w1008 {
      selector: w1008 -> [w1017 w1151]
      tunnel: [w1018 w1145] -> w1007
      tunnel: w1006 -> [w1016 _]
      tunnel: [w1015 Communications_-_State."Idle"] -> w1005
      tunnel: [w1014 _] -> w1004
      tunnel: [w1013 w1153] -> w1003
      tunnel: w1002 -> [w1012 w1153]
      tunnel: w1001 -> [w1011 w1142]
      tunnel: [w1010 w1141] -> w999
      tunnel: w998 -> [w1009 w1141]
      frame No Error {
        n360 = case shown="\"Command\"" w1016 {
          tunnel: [w1022 w1042 w1077 w1132] -> w1018
          tunnel: w1017 -> [w1027 w1041 w1080 w1136]
          tunnel: [Communications_-_State."Idle" w1030 Communications_-_State."Idle" Communications_-_State."Close"] -> w1015
          tunnel: [_ _ _ TRUE] -> w1014
          tunnel: [w1024 w1040 w1079 w1138] -> w1013
          tunnel: w1012 -> [_ w1039 w1079 w1138]
          tunnel: w1011 -> [_ w1034 w1066 w1134]
          tunnel: [0 ("index") w1029 w1065 0 ("index")] -> w1010
          tunnel: w1009 -> [_ w1029 w1064 _]
          frame "Init", Default {
            n361 = call "Communication - UDP Command (eFGV).vi"("Action"=eFGV_States."Read", "error in"=w1027) -> ("error out"=w1023:errorcluster, "UDP Ref"=w1021:refnum<user-event>)  [unwired: 7 in, 1 out]
            n362 = register-events(error in=w1023, w1021) -> (reference out=w1020:refnum<event-registration>, error out=w1022:errorcluster)  [unwired: 1 in]
            n363 = Bundle By Name(cluster=T6 {"UDP CMD"={"IP"="", "CMD"=enum."Stop", "Port"="", "Datalog?"=FALSE, "Float"=0.0}, "Unit?"=FALSE, "Read Unit"=[], "Trig?"=FALSE, "UDP Info"=[], "DataLogger"=[], "VISA Ref"=refnum, "Float"=0.0, "Data"={"Test"={"Target Load"=0.0, "Target Disp"=0.0, "Rate"=0.0, "Speed"=0.0}, "Sensor"={"Name"=[], "Unit"=[], "Decimal Point"=[], "Ch Log"=[], "H Alarm"=[], "L Alarm"=[], "H Limit"=[], "L Limit"=[], "Filter"=[], "Gain"=[], "Calib Type"=[]}, "PID"={"SP"=-2.7823365e-08, "PV"=-3.023652e-13, "kP"=8.5432666e-24, "kI"=2.29252e-41, "kD"=1.570387e-38, "FF"=25.0, "Err Band"=0.0, "Max"=15, "Min"=-7, "Ts"=1886611780, "Out"=0, "Mode"=0}, "ADC"={"Active Ch"=[255, 255, 255, 0, 0, 0, 0, 0], "Filter Type"=2, "Post Filter"=[1, 1, 1, 1, 0, 200, 66, 184], "Gain"=[0, 0, 0, 0, 0, 122, 68, 0], "FS"=32, "IntOC"=0, "IntFC"=255, "SysOC"=255, "Cofficient"=[1.0, 1.0, 1.0, 1.0, 1.0, 1.0, 1.0, 1.0], "K"=[1.2450000047683716, 1.2450000047683716], "Max"=1048576}, "System"={"Out Type"=0, "Inverse"=0, "Monitor"=0, "Reserve"=0, "ACC Time"=0, "Pulse Rev"=0, "Stroke"=0, "Auto Off"=0, "Gear Ratio"=0.0, "Pitch"=0.0, "Max Speed"=0, "Jog Speed"=0, "Disp Coff"=0.0, "Max Load"=0}, "Index"=enum."Ch1", "Datalog"=enum."Empty"}, "UDP Event Ref"=refnum, "UDP ref"=refnum, "Read Sensor"=0}, "UDP Event Ref"=w1020) -> (w1024:T6)
          }
          frame "Idle" {
            n364 = Unbundle By Name(w1039) -> ("UDP Event Ref"=w1043:refnum<event-registration>)
            n365 = event shown="[0] Timeout" {
              selector: w1043 -> [_ _]
              dyn-events: _ -> [_ _]
              timeout: 3000 -> [_ _]
              tunnel: [w1049 w1052] -> w1037
              tunnel: [w1046 _] -> w1042
              tunnel: w1041 -> [w1046 _]
              tunnel: [w1044 w1061] -> w1040
              tunnel: w1039 -> [w1044 w1060]
              tunnel: w1034 -> [_ w1050]
              event Timeout {
                n366 = event-data() -> ()  [unwired: 1 in, 1 out]
                n367 = local read "Stop"() -> (w1048:bool)
                n368 = Select(t=Communications_-_State."Close", s=w1048, f=Communications_-_State."Idle") -> (s? t:f=w1049:T2)
              }
              event User Event {
                n369 = event-data() -> ("IP"=w1055:string, "CMD"=w1059:T1, "Data"=w1058:T7)  [unwired: 1 in]
                n370 = global read "Global - IP Address.vi" "IP"() -> (w1057:string[])
                n371 = Index Array(array=w1057, index=w1050) -> (element=w1056:string)
                n372 = Equal?(x=w1056, y=w1055) -> (x = y?=w1054:bool)
                n373 = Bundle By Name(cluster=w1060, "UDP CMD.IP"=w1055, "UDP CMD.CMD"=w1059, "Data"=w1058) -> (w1061:T6)
                n374 = Select(t=Communications_-_State."Command" ("f"), s=w1054, f=Communications_-_State."Idle") -> (s? t:f=w1052:T2)
              }
            }
            n375 = global read "Global - Hold.vi" "Hold"() -> (w1038:bool)
            n376 = Select(t=Communications_-_State."Idle", s=w1038, f=w1037) -> (s? t:f=w1031:T2)
            n377 = local read "Stop"() -> (w1032:bool)
            n378 = Select(t=Communications_-_State."Close", s=w1032, f=w1031) -> (s? t:f=w1030:T2)
          }
          frame "Command" {
            n379 = Unbundle By Name(w1079) -> ("UDP CMD.CMD"=w1076:T1, "Data"=w1078:T7, "UDP CMD.IP"=w1062:string)
            "12" <- w1076
            n380 = global read "Global - Handle V1.vi" "Handle"() -> (w1070:refnum<visa-resource-name>[])
            n381 = global read "Global - IP Address.vi" "IP"() -> (w1071:string[])
            n382 = Search 1D Array(1D array=w1071, element=w1062) -> ()  [unwired: 1 in, 1 out]
            n383 = Index Array(array=w1070, index=w1066) -> (element=w1072:refnum<visa-resource-name>)
            n384 = call "VISA - Write CMD.vi"("Index"=w1066, "error in"=w1080, "Data"=w1078, "Action"=w1076, "VISA ref"=w1072) -> ("error out"=w1068:errorcluster, "Data Unit"=w1074:T12, "Data Channel"=w1075:T13, "Success"=w1073:bool, "Prev Data?"=→"Prev 12":bool)  [unwired: 2 out]
            "Success12" <- w1073
            n385 = flat-sequence {
              tunnel: w1066 -> [w1086]
              tunnel: [w1083] -> w1069
              tunnel: w1068 -> [w1083]
              frame #0 {
                n386 = global read "Global - Done.vi" "Done"() -> (w1085:bool[])
                n387 = Replace Array Subset(array=w1085, new element=TRUE, index=w1086) -> (w1084:bool[])
                n388 = global write "Global - Done.vi" "Done"(w1084) -> ()
              }
            }
            n389 = global write "Global - Data UDP.vi" "Loop 13"(TRUE ("Loop 1")) -> ()
            n390 = case shown="False" w1073 {
              tunnel: w1069 -> [w1090 w1105]
              tunnel: [w1091 w1104] -> w1077
              tunnel: w1076 -> [_ w1106]
              tunnel: w1075 -> [_ w1103]
              tunnel: w1074 -> [_ w1102]
              tunnel: w1066 -> [_ w1101]
              tunnel: [w1087 0 ("index")] -> w1065
              tunnel: w1064 -> [w1092 _]
              tunnel: w1062 -> [w1088 _]
              frame False {
                n391 = Increment(x=w1092) -> (x+1=w1089:i32)
                n392 = case shown="5" w1089 {
                  selector: w1089 -> [w1093 _]
                  tunnel: [w1094 w1099] -> w1091
                  tunnel: w1090 -> [w1094 w1098]
                  tunnel: w1088 -> [_ w1096]
                  tunnel: [w1093 0] -> w1087
                  frame 0, Default {
                  }
                  frame 5 {
                    n393 = call "Communication - Reconnect eFGV.vi"("eFGV States"=eFGV_States."Write", "error in (no error)"=w1098, "Reconnect In"=w1096) -> ("error out"=w1099:errorcluster)  [unwired: 6 in, 2 out]
                  }
                }
              }
              frame True {
                n394 = case shown="\"Read Ch Data\"" w1106 {
                  tunnel: w1105 -> [w1107 w1114 w1129]
                  tunnel: [w1107 w1114 w1129] -> w1104
                  tunnel: w1103 -> [_ w1112 _]
                  tunnel: w1102 -> [_ _ w1125]
                  tunnel: w1101 -> [_ w1116 w1130]
                  frame "Stop", Default {
                  }
                  frame "Read Ch Data" {
                    n395 = Unbundle By Name(w1112) -> ("Ch1 Data"=w1111:sgl, "Ch2 Data"=w1110:sgl)
                    n396 = global read "Global - Channel.vi" "Data"() -> (w1115:T14)
                    n397 = Bundle By Name(cluster=T10 {"Channels"={"Ch1"=0.0, "Ch2"=0.0, "Ch3"=0.0, "Ch4"=0.0, "Ch5"=0.0, "Ch6"=0.0, "Ch7"=0.0, "Ch8"=0.0, "Ch9"=0.0, "Ch10"=0.0, "Ch11"=0.0, "Ch12"=0.0, "Ch13"=0.0, "Ch14"=0.0, "Ch15"=0.0, "Ch16"=0.0}, "Event"=0, "Status"=0, "IP"=""} ("Data Channel"), "Channels.Ch1"=w1111, "Channels.Ch2"=w1110) -> (w1109:T10)
                    n398 = Replace Array Subset(array=w1115, new element=w1109, index=w1116) -> (w1113:T14)
                    n399 = global write "Global - Channel.vi" "Data"(w1113) -> ()
                  }
                  frame "Read Sensor" {
                    n400 = Unbundle By Name(w1125) -> ("Ch1 Unit"=w1124:string, "Ch2 Unit"=w1123:string, "Ch1 Decimal"=w1122:u8, "Ch2 Decimal"=w1121:u8)
                    n401 = global read "Global - Unit.vi" "Unit"() -> (w1127:T15)
                    n402 = Build Array(w1124, w1123) -> (w1120:string[])
                    n403 = Build Array(w1122, w1121) -> (w1119:u8[])
                    n404 = Bundle By Name(cluster=T11 {"Name"=[], "Unit"=[], "Decimal Point"=[], "Ch Log"=[], "H Alarm"=[], "L Alarm"=[], "H Limit"=[], "L Limit"=[], "Filter"=[], "Gain"=[], "Calib Type"=[]} ("Sensor"), "Name"=string[] ["Load", "Displacement"], "Unit"=w1120, "Decimal Point"=w1119) -> (w1118:T11)
                    n405 = Replace Array Subset(array=w1127, new element=w1118, index=w1130) -> (w1128:T15)
                    n406 = global write "Global - Unit.vi" "Unit"(w1128) -> ()
                  }
                }
              }
            }
          }
          frame "Close" {
            n407 = global read "Global - Handle V1.vi" "Handle"() -> (w1135:refnum<visa-resource-name>[])
            n408 = Index Array(array=w1135, index=w1134) -> (element=w1133:refnum<visa-resource-name>)
            n409 = VISA Close(VISA resource name=w1133, error in (no error)=w1136) -> (error out=w1137:errorcluster)
            n410 = call <vilib>:"Clear Errors.vi"("error in (no error)"=w1137) -> ("error out"=w1132:errorcluster)  [unwired: 5 in, 1 out]
          }
        }
      }
      frame Error {
        n411 = global read "Global - IP Address.vi" "IP"() -> (w1150:string[])
        n412 = Unbundle By Name(w1151) -> ("source"=w1147:string)
        n413 = Index Array(array=w1150, index=w1142) -> (element=w1149:string)
        n414 = Concatenate Strings(w1149, " - " ("string"), w1147) -> (w1143:string)
        n415 = call <vilib>:"Clear Errors.vi"("error in (no error)"=w1151) -> ("error out"=w1146:errorcluster)  [unwired: 5 in, 1 out]
        n416 = call "General - Error Log eFGV.vi"("eFGV States"=eFGV_States."Write", "error in (no error)"=w1146, "Error In"=w1143) -> ("error out"=w1145:errorcluster)  [unwired: 6 in, 2 out]
        n417 = Wait (ms)(milliseconds to wait=u32 100) -> ()  [unwired: 1 out]
      }
    }
    "12" <- w1006
    "loop 12" <- w1000
  }
  n418 = while {
    shift-right: [w1164] -> _
    shift-left: errorcluster {"status"=FALSE, "code"=0, "source"=""} ("error IO") -> [w1165]
    shift-right: [w1162] -> _
    shift-left: Communications_-_State."Init" -> [w1163]
    shift-right: [w1160] -> _
    shift-left: _ -> [w1159]
    tunnel: 14 ("index") -> [w1158]
    shift-right: [w1156] -> _
    shift-left: _ -> [w1155]
    i -> [w1157]
    stop <- w1161 stop-if-true
    # "Queue Command Processing Loop"
    n419 = case shown="No Error" w1165 {
      selector: w1165 -> [w1174 w1307]
      tunnel: [w1175 w1301] -> w1164
      tunnel: w1163 -> [w1173 _]
      tunnel: [w1172 Communications_-_State."Idle"] -> w1162
      tunnel: [w1171 _] -> w1161
      tunnel: [w1170 w1309] -> w1160
      tunnel: w1159 -> [w1169 w1309]
      tunnel: w1158 -> [w1168 w1298]
      tunnel: [w1167 w1297] -> w1156
      tunnel: w1155 -> [w1166 w1297]
      frame No Error {
        n420 = case shown="\"Command\"" w1173 {
          tunnel: [w1179 w1199 w1234 w1291] -> w1175
          tunnel: w1174 -> [w1184 w1198 w1237 w1290]
          tunnel: [Communications_-_State."Idle" w1187 Communications_-_State."Idle" Communications_-_State."Close"] -> w1172
          tunnel: [_ _ _ TRUE] -> w1171
          tunnel: [w1181 w1197 w1236 w1294] -> w1170
          tunnel: w1169 -> [_ w1196 w1236 w1294]
          tunnel: w1168 -> [_ w1191 w1223 w1289]
          tunnel: [0 w1186 w1221 0] -> w1167
          tunnel: w1166 -> [_ w1186 w1220 _]
          frame "Init", Default {
            n421 = call "Communication - UDP Command (eFGV).vi"("Action"=eFGV_States."Read", "error in"=w1184) -> ("error out"=w1180:errorcluster, "UDP Ref"=w1178:refnum<user-event>)  [unwired: 7 in, 1 out]
            n422 = register-events(error in=w1180, w1178) -> (reference out=w1177:refnum<event-registration>, error out=w1179:errorcluster)  [unwired: 1 in]
            n423 = Bundle By Name(cluster=T6 {"UDP CMD"={"IP"="", "CMD"=enum."Stop", "Port"="", "Datalog?"=FALSE, "Float"=0.0}, "Unit?"=FALSE, "Read Unit"=[], "Trig?"=FALSE, "UDP Info"=[], "DataLogger"=[], "VISA Ref"=refnum, "Float"=0.0, "Data"={"Test"={"Target Load"=0.0, "Target Disp"=0.0, "Rate"=0.0, "Speed"=0.0}, "Sensor"={"Name"=[], "Unit"=[], "Decimal Point"=[], "Ch Log"=[], "H Alarm"=[], "L Alarm"=[], "H Limit"=[], "L Limit"=[], "Filter"=[], "Gain"=[], "Calib Type"=[]}, "PID"={"SP"=-2.7823365e-08, "PV"=-3.023652e-13, "kP"=8.5432666e-24, "kI"=2.29252e-41, "kD"=1.570387e-38, "FF"=25.0, "Err Band"=0.0, "Max"=15, "Min"=-7, "Ts"=1886611780, "Out"=0, "Mode"=0}, "ADC"={"Active Ch"=[255, 255, 255, 0, 0, 0, 0, 0], "Filter Type"=2, "Post Filter"=[1, 1, 1, 1, 0, 200, 66, 184], "Gain"=[0, 0, 0, 0, 0, 122, 68, 0], "FS"=32, "IntOC"=0, "IntFC"=255, "SysOC"=255, "Cofficient"=[1.0, 1.0, 1.0, 1.0, 1.0, 1.0, 1.0, 1.0], "K"=[1.2450000047683716, 1.2450000047683716], "Max"=1048576}, "System"={"Out Type"=0, "Inverse"=0, "Monitor"=0, "Reserve"=0, "ACC Time"=0, "Pulse Rev"=0, "Stroke"=0, "Auto Off"=0, "Gear Ratio"=0.0, "Pitch"=0.0, "Max Speed"=0, "Jog Speed"=0, "Disp Coff"=0.0, "Max Load"=0}, "Index"=enum."Ch1", "Datalog"=enum."Empty"}, "UDP Event Ref"=refnum, "UDP ref"=refnum, "Read Sensor"=0}, "UDP Event Ref"=w1177) -> (w1181:T6)
          }
          frame "Idle" {
            n424 = Unbundle By Name(w1196) -> ("UDP Event Ref"=w1200:refnum<event-registration>)
            n425 = event shown="[0] Timeout" {
              selector: w1200 -> [_ _]
              dyn-events: _ -> [_ _]
              timeout: 3000 -> [_ _]
              tunnel: [w1206 w1209] -> w1194
              tunnel: [w1203 _] -> w1199
              tunnel: w1198 -> [w1203 _]
              tunnel: [w1201 w1218] -> w1197
              tunnel: w1196 -> [w1201 w1217]
              tunnel: w1191 -> [_ w1207]
              event Timeout {
                n426 = event-data() -> ()  [unwired: 1 in, 1 out]
                n427 = local read "Stop"() -> (w1205:bool)
                n428 = Select(t=Communications_-_State."Close", s=w1205, f=Communications_-_State."Idle") -> (s? t:f=w1206:T2)
              }
              event User Event {
                n429 = event-data() -> ("IP"=w1212:string, "CMD"=w1216:T1, "Data"=w1215:T7)  [unwired: 1 in]
                n430 = global read "Global - IP Address.vi" "IP"() -> (w1214:string[])
                n431 = Index Array(array=w1214, index=w1207) -> (element=w1213:string)
                n432 = Equal?(x=w1213, y=w1212) -> (x = y?=w1211:bool)
                n433 = Bundle By Name(cluster=w1217, "UDP CMD.IP"=w1212, "UDP CMD.CMD"=w1216, "Data"=w1215) -> (w1218:T6)
                n434 = Select(t=Communications_-_State."Command" ("f"), s=w1211, f=Communications_-_State."Idle") -> (s? t:f=w1209:T2)
              }
            }
            n435 = global read "Global - Hold.vi" "Hold"() -> (w1195:bool)
            n436 = Select(t=Communications_-_State."Idle", s=w1195, f=w1194) -> (s? t:f=w1188:T2)
            n437 = local read "Stop"() -> (w1189:bool)
            n438 = Select(t=Communications_-_State."Close", s=w1189, f=w1188) -> (s? t:f=w1187:T2)
          }
          frame "Command" {
            n439 = Unbundle By Name(w1236) -> ("UDP CMD.CMD"=w1233:T1, "Data"=w1235:T7, "UDP CMD.IP"=w1219:string)
            "14" <- w1233
            n440 = global read "Global - Handle V1.vi" "Handle"() -> (w1227:refnum<visa-resource-name>[])
            n441 = global read "Global - IP Address.vi" "IP"() -> (w1228:string[])
            n442 = Search 1D Array(1D array=w1228, element=w1219) -> ()  [unwired: 1 in, 1 out]
            n443 = Index Array(array=w1227, index=w1223) -> (element=w1229:refnum<visa-resource-name>)
            n444 = call "VISA - Write CMD.vi"("Index"=w1223, "error in"=w1237, "Data"=w1235, "Action"=w1233, "VISA ref"=w1229) -> ("error out"=w1225:errorcluster, "Data Unit"=w1231:T12, "Data Channel"=w1232:T13, "Success"=w1230:bool, "Prev Data?"=→"Prev 14":bool)  [unwired: 2 out]
            "Success14" <- w1230
            n445 = flat-sequence {
              tunnel: w1223 -> [w1243]
              tunnel: [w1240] -> w1226
              tunnel: w1225 -> [w1240]
              frame #0 {
                n446 = global read "Global - Done.vi" "Done"() -> (w1242:bool[])
                n447 = Replace Array Subset(array=w1242, new element=TRUE, index=w1243) -> (w1241:bool[])
                n448 = global write "Global - Done.vi" "Done"(w1241) -> ()
              }
            }
            n449 = global write "Global - Data UDP.vi" "Loop 15"(TRUE ("Loop 3")) -> ()
            n450 = case shown="False" w1230 {
              tunnel: w1226 -> [w1247 w1262]
              tunnel: [w1248 w1261] -> w1234
              tunnel: w1233 -> [_ w1263]
              tunnel: w1232 -> [_ w1260]
              tunnel: w1231 -> [_ w1259]
              tunnel: w1223 -> [_ w1258]
              tunnel: [w1244 0] -> w1221
              tunnel: w1220 -> [w1249 _]
              tunnel: w1219 -> [w1246 _]
              frame False {
                n451 = Increment(x=w1249) -> (x+1=w1245:i32)
                n452 = case shown="5" w1245 {
                  selector: w1245 -> [w1250 _]
                  tunnel: [w1251 w1255] -> w1248
                  tunnel: w1247 -> [w1251 w1254]
                  tunnel: w1246 -> [_ w1253]
                  tunnel: [w1250 0] -> w1244
                  frame 0, Default {
                  }
                  frame 5 {
                    n453 = call "Communication - Reconnect eFGV.vi"("eFGV States"=eFGV_States."Write", "error in (no error)"=w1254, "Reconnect In"=w1253) -> ("error out"=w1255:errorcluster)  [unwired: 6 in, 2 out]
                  }
                }
              }
              frame True {
                n454 = case shown="\"Read Sensor\"" w1263 {
                  tunnel: w1262 -> [w1264 w1271 w1286]
                  tunnel: [w1264 w1271 w1286] -> w1261
                  tunnel: w1260 -> [_ w1269 _]
                  tunnel: w1259 -> [_ _ w1282]
                  tunnel: w1258 -> [_ w1273 w1287]
                  frame "Stop", Default {
                  }
                  frame "Read Ch Data" {
                    n455 = Unbundle By Name(w1269) -> ("Ch1 Data"=w1268:sgl, "Ch2 Data"=w1267:sgl)
                    n456 = global read "Global - Channel.vi" "Data"() -> (w1272:T14)
                    n457 = Bundle By Name(cluster=T10 {"Channels"={"Ch1"=0.0, "Ch2"=0.0, "Ch3"=0.0, "Ch4"=0.0, "Ch5"=0.0, "Ch6"=0.0, "Ch7"=0.0, "Ch8"=0.0, "Ch9"=0.0, "Ch10"=0.0, "Ch11"=0.0, "Ch12"=0.0, "Ch13"=0.0, "Ch14"=0.0, "Ch15"=0.0, "Ch16"=0.0}, "Event"=0, "Status"=0, "IP"=""} ("Data Channel"), "Channels.Ch1"=w1268, "Channels.Ch2"=w1267) -> (w1266:T10)
                    n458 = Replace Array Subset(array=w1272, new element=w1266, index=w1273) -> (w1270:T14)
                    n459 = global write "Global - Channel.vi" "Data"(w1270) -> ()
                  }
                  frame "Read Sensor" {
                    n460 = Unbundle By Name(w1282) -> ("Ch1 Unit"=w1281:string, "Ch2 Unit"=w1280:string, "Ch1 Decimal"=w1279:u8, "Ch2 Decimal"=w1278:u8)
                    n461 = global read "Global - Unit.vi" "Unit"() -> (w1284:T15)
                    n462 = Build Array(w1281, w1280) -> (w1277:string[])
                    n463 = Build Array(w1279, w1278) -> (w1276:u8[])
                    n464 = Bundle By Name(cluster=T11 {"Name"=[], "Unit"=[], "Decimal Point"=[], "Ch Log"=[], "H Alarm"=[], "L Alarm"=[], "H Limit"=[], "L Limit"=[], "Filter"=[], "Gain"=[], "Calib Type"=[]} ("Sensor"), "Name"=string[] ["Load", "Displacement"], "Unit"=w1277, "Decimal Point"=w1276) -> (w1275:T11)
                    n465 = Replace Array Subset(array=w1284, new element=w1275, index=w1287) -> (w1285:T15)
                    n466 = global write "Global - Unit.vi" "Unit"(w1285) -> ()
                  }
                }
              }
            }
          }
          frame "Close" {
            n467 = global read "Global - Handle V1.vi" "Handle"() -> (w1293:refnum<visa-resource-name>[])
            n468 = Index Array(array=w1293, index=w1289) -> (element=w1292:refnum<visa-resource-name>)
            n469 = VISA Close(VISA resource name=w1292, error in (no error)=w1290) -> (error out=w1291:errorcluster)
          }
        }
      }
      frame Error {
        n470 = global read "Global - IP Address.vi" "IP"() -> (w1306:string[])
        n471 = Unbundle By Name(w1307) -> ("source"=w1303:string)
        n472 = Index Array(array=w1306, index=w1298) -> (element=w1305:string)
        n473 = Concatenate Strings(w1305, " - " ("string"), w1303) -> (w1299:string)
        n474 = call <vilib>:"Clear Errors.vi"("error in (no error)"=w1307) -> ("error out"=w1302:errorcluster)  [unwired: 5 in, 1 out]
        n475 = call "General - Error Log eFGV.vi"("eFGV States"=eFGV_States."Write", "error in (no error)"=w1302, "Error In"=w1299) -> ("error out"=w1301:errorcluster)  [unwired: 6 in, 2 out]
        n476 = Wait (ms)(milliseconds to wait=u32 100) -> ()  [unwired: 1 out]
      }
    }
    "14" <- w1163
    "loop 14" <- w1157
  }
  n477 = control-ref of="This VI"() -> (w44:refnum<vi>)
  n478 = invoke class="VI" method="FP.Open"(reference=w44, "Activate"=TRUE ("Activate?"), "State"=T3."Minimized") -> ()  [unwired: 2 in, 5 out]
  n479 = local write "Stop"(FALSE ("Stop")) -> ()
  n480 = while {
    shift-right: [w1319] -> w1
    shift-left: errorcluster {"status"=FALSE, "code"=0, "source"=""} ("error IO") -> [w1320]
    shift-right: [w1317] -> _
    shift-left: Communications_-_State."Init" -> [w1318]
    shift-right: [w1316] -> _
    shift-left: _ -> [w1315]
    shift-right: [w1313] -> _
    shift-left: _ -> [w1312]
    i -> [w1311]
    stop <- w1314 stop-if-true
    # "UI Loop"
    n481 = case shown="No Error" w1320 {
      selector: w1320 -> [w1328 w1509]
      tunnel: [w1329 w1510] -> w1319
      tunnel: w1318 -> [w1327 _]
      tunnel: [w1326 Communications_-_State."Idle"] -> w1317
      tunnel: [w1325 w1515] -> w1316
      tunnel: w1315 -> [w1324 w1515]
      tunnel: [w1323 _] -> w1314
      tunnel: [w1322 w1514] -> w1313
      tunnel: w1312 -> [w1321 w1514]
      frame No Error {
        n482 = case shown="\"Close\"" w1327 {
          tunnel: [w1330 w1348 w1379 w1456 w1483 w1491] -> w1329
          tunnel: w1328 -> [w1334 w1347 w1393 w1458 w1482 w1492]
          tunnel: [Communications_-_State."Get IP Address" w1346 Communications_-_State."Command" w1451 Communications_-_State."Idle" Communications_-_State."Close"] -> w1326
          tunnel: [w1337 w1344 w1396 w1459 w1486 w1496] -> w1325
          tunnel: w1324 -> [_ w1345 w1396 w1459 w1486 w1496]
          tunnel: [_ _ _ _ _ w1494] -> w1323
          tunnel: [T6 {"UDP CMD"={"IP"="", "CMD"=enum."Stop", "Port"="", "Datalog?"=FALSE, "Float"=0.0}, "Unit?"=FALSE, "Read Unit"=[], "Trig?"=FALSE, "UDP Info"=[], "DataLogger"=[], "VISA Ref"=refnum, "Float"=0.0, "Data"={"Test"={"Target Load"=0.0, "Target Disp"=0.0, "Rate"=0.0, "Speed"=0.0}, "Sensor"={"Name"=[], "Unit"=[], "Decimal Point"=[], "Ch Log"=[], "H Alarm"=[], "L Alarm"=[], "H Limit"=[], "L Limit"=[], "Filter"=[], "Gain"=[], "Calib Type"=[]}, "PID"={"SP"=-2.7823365e-08, "PV"=-3.023652e-13, "kP"=8.5432666e-24, "kI"=2.29252e-41, "kD"=1.570387e-38, "FF"=25.0, "Err Band"=0.0, "Max"=15, "Min"=-7, "Ts"=1886611780, "Out"=0, "Mode"=0}, "ADC"={"Active Ch"=[255, 255, 255, 0, 0, 0, 0, 0], "Filter Type"=2, "Post Filter"=[1, 1, 1, 1, 0, 200, 66, 184], "Gain"=[0, 0, 0, 0, 0, 122, 68, 0], "FS"=32, "IntOC"=0, "IntFC"=255, "SysOC"=255, "Cofficient"=[1.0, 1.0, 1.0, 1.0, 1.0, 1.0, 1.0, 1.0], "K"=[1.2450000047683716, 1.2450000047683716], "Max"=1048576}, "System"={"Out Type"=0, "Inverse"=0, "Monitor"=0, "Reserve"=0, "ACC Time"=0, "Pulse Rev"=0, "Stroke"=0, "Auto Off"=0, "Gear Ratio"=0.0, "Pitch"=0.0, "Max Speed"=0, "Jog Speed"=0, "Disp Coff"=0.0, "Max Load"=0}, "Index"=enum."Ch1", "Datalog"=enum."Empty"}, "UDP Event Ref"=refnum, "UDP ref"=refnum, "Read Sensor"=0} w1343 w1381 w1450 w1485 w1493] -> w1322
          tunnel: w1321 -> [_ w1342 w1380 w1449 w1485 w1493]
          frame "Init", Default {
            w1333 = eFGV_States."Read" ("Action")
            n483 = call "Communication - Trigger Read IP Address(FGV).vi"("Action"=w1333, "error in"=w1334) -> ("error out"=w1335:errorcluster, "Trigger ref"=w1332:refnum<user-event>)  [unwired: 7 in, 1 out]
            n484 = call "General - Exit eFGV.vi"("eFGV States"=w1333, "error in (no error)"=w1335) -> ("error out"=w1339:errorcluster, "Exit"=w1338:refnum<user-event>)  [unwired: 7 in, 1 out]
            n485 = register-events(error in=w1339, w1338, w1332) -> (reference out=w1337:refnum<event-registration>, error out=w1330:errorcluster)  [unwired: 1 in]
            n486 = global write "Global - Hold.vi" "Hold"(FALSE ("Hold")) -> ()
          }
          frame "Idle" {
            n487 = event shown="[4] \"stop\": Value Change" {
              selector: w1345 -> [_ _ _ _ _]
              dyn-events: [_ _ _ _ _] -> w1344
              timeout: 1000 -> [_ _ _ _ _]
              tunnel: [w1355 w1362 w1363 w1370 w1377] -> w1348
              tunnel: w1347 -> [w1354 w1362 w1363 w1370 w1377]
              tunnel: [w1349 Communications_-_State."Get IP Address" Communications_-_State."Close" Communications_-_State."Idle" Communications_-_State."Close"] -> w1346
              tunnel: [w1356 w1360 w1364 w1369 w1376] -> w1343
              tunnel: w1342 -> [w1356 w1359 w1364 w1369 w1376]
              event Timeout {
                n488 = event-data() -> ()  [unwired: 1 in, 3 out]
                n489 = call "General - Exit eFGV.vi"("eFGV States"=eFGV_States."Read", "error in (no error)"=w1354) -> ("error out"=w1355:errorcluster, "Exit Out"=w1352:bool)  [unwired: 7 in, 1 out]
                n490 = Select(t=Communications_-_State."Close", s=w1352, f=Communications_-_State."Get IP Address") -> (s? t:f=w1349:T2)
              }
              event User Event {
                n491 = event-data() -> ()  [unwired: 1 in, 1 out]
                n492 = Bundle By Name(cluster=w1359, "Trig?"=TRUE) -> (w1360:T6)
                n493 = global write "Global - Hold.vi" "Hold"(FALSE ("Hold")) -> ()
              }
              event User Event {
                n494 = event-data() -> ()  [unwired: 1 in, 5 out]
              }
              event "Break": Value Change {
                n495 = event-data() -> ()  [unwired: 1 in, 6 out]
                n496 = global read "Global - Handle V1.vi" "Handle"() -> (w1366:refnum<visa-resource-name>[])
                n497 = global read "Global - IP Address.vi" "IP"() -> (w1367:string[])
                n498 = for {
                  tunnel: w1367 -> [w1373] mode=indexing
                  tunnel: w1366 -> [w1371] mode=indexing
                  n499 = Empty String/Path?(string/path=w1373) -> (empty?=w1372:bool)
                  n500 = case shown="False" w1372 {
                    tunnel: w1371 -> [w1374 _]
                    frame False {
                      n501 = call-poly <vilib>:"VISA Serial Break.vi"("VISA resource name"=w1374) -> ()  [unwired: 3 in, 2 out]
                    }
                    frame True {
                    }
                  }
                }
              }
              event "stop": Value Change {
                n502 = event-data() -> ()  [unwired: 1 in, 6 out]
              }
            }
          }
          frame "Get IP Address" {
            n503 = global read "Global - Comport.vi" "Port"() -> (w1384:string[])
            n504 = global read "Global - Data UDP.vi" "V1"() -> (w1378:bool)
            n505 = global read "Global - Handle V1.vi" "Handle"() -> (w1387:refnum<visa-resource-name>[])
            n506 = global read "Global - Device.vi" "Device"() -> (w1386:string[])
            n507 = call "Machine - Config File.vi"("Action"=enum16{"Write", "Read", "Read All", "Remove"}."Read All", "V1"=w1378, "error in (no error)"=w1393) -> ("error out"=w1394:errorcluster, "Value Out"=w1392:cluster{"IP/SN":string, "Key Value":string[]}[])  [unwired: 7 in]
            n508 = global read "Global - IP Address.vi" "IP"() -> (w1388:string[])
            n509 = for {
              tunnel: w1394 -> [w1420]
              tunnel: [w1421] -> w1379
              tunnel: [w1408] -> w1391 mode=indexing
              tunnel: [w1405] -> w1390 mode=indexing
              tunnel: w1392 -> [w1419] mode=indexing
              tunnel: [w1398] -> w1389 mode=indexing
              tunnel: w1388 -> [w1415]
              tunnel: w1387 -> [w1411]
              tunnel: w1386 -> [w1414]
              tunnel: [w1402] -> w1385 mode=indexing
              tunnel: w1384 -> [w1413]
              tunnel: [w1412] -> w1382 mode=indexing
              n510 = Unbundle By Name(w1419) -> ("IP/SN"=w1417:string, "Key Value"=w1418:string[])
              n511 = Search 1D Array(1D array=w1415, element=w1417) -> (index of element=w1410:i32)  [unwired: 1 in]
              n512 = Greater Or Equal To 0?(x=w1410) -> (x >= 0?=w1416:bool)
              n513 = case shown="False" w1416 {
                tunnel: [w1429 w1447] -> w1421
                tunnel: w1420 -> [w1430 w1447]
                tunnel: w1418 -> [w1433 _]
                tunnel: [w1431 w1442] -> w1399
                tunnel: [w1426 w1444] -> w1406
                tunnel: [w1423 w1435] -> w1400
                tunnel: w1417 -> [w1432 _]
                tunnel: [w1432 w1436] -> w1409
                tunnel: w1415 -> [_ w1446]
                tunnel: w1410 -> [_ w1441]
                tunnel: w1411 -> [_ w1445]
                tunnel: w1414 -> [_ w1443]
                tunnel: [w1428 w1439] -> w1403
                tunnel: w1413 -> [_ w1440]
                tunnel: [w1423 FALSE] -> w1412
                frame False {
                  n514 = Index Array(array=w1433) -> (element #1=w1428:string, element #2=w1431:string)  [unwired: 2 in]
                  n515 = Empty String/Path?(string/path=w1432) -> (empty?=w1434:bool)
                  n516 = call "VISA - Open Connection.vi"("Enable Termination\nChar (T)"="Enable Termination\nChar (T)", "error in"=w1430, "VISA resource name"=w1428) -> ("error out"=w1429:errorcluster, "VISA Ref"=w1426:refnum<visa-resource-name>)  [unwired: 7 in]
                  n517 = Not(x=w1434) -> (.not. x?=w1425:bool)
                  n518 = Empty String/Path?(string/path=w1426) -> (empty?=w1427:bool)
                  n519 = Not(x=w1427) -> (.not. x?=w1424:bool)
                  n520 = And(x=w1425, y=w1424) -> (x .and. y?=w1423:bool)
                }
                frame True {
                  n521 = Index Array(array=w1443, index=w1441) -> (element=w1442:string)
                  n522 = Index Array(array=w1446, index=w1441) -> (element=w1436:string)
                  n523 = Index Array(array=w1445, index=w1441) -> (element=w1444:refnum<visa-resource-name>)
                  n524 = Index Array(array=w1440, index=w1441) -> (element=w1439:string)
                  n525 = Empty String/Path?(string/path=w1436) -> (empty?=w1437:bool)
                  n526 = Not(x=w1437) -> (.not. x?=w1435:bool)
                }
              }
              n527 = Select(t=w1409, s=w1400, f="") -> (s? t:f=w1408:string)
              n528 = Select(t=w1406, s=w1400, f=refnum<visa-resource-name> refnum) -> (s? t:f=w1405:refnum<visa-resource-name>)
              n529 = Select(t=w1403, s=w1400, f="") -> (s? t:f=w1402:string)
              n530 = Select(t=w1399, s=w1400, f="") -> (s? t:f=w1398:string)
            }
            "SN" <- w1391
            "Device" <- w1389
            n531 = global write "Global - Handle V1.vi" "Handle"(w1390) -> ()
            n532 = global write "Global - Device.vi" "Device"(w1389) -> ()
            n533 = global write "Global - IP Address.vi" "IP"(w1391) -> ()
            n534 = global write "Global - Comport.vi" "Port"(w1385) -> ()
            n535 = Bundle By Name(cluster=w1380, "Read Unit"=w1382) -> (w1381:T6)
          }
          frame "Command" {
            n536 = Unbundle By Name(w1449) -> ("Trig?"=w1454:bool, "Read Unit"=w1457:bool[])
            n537 = global read "Global - IP Address.vi" "IP"() -> (w1448:string[])
            n538 = for {
              shift-right: [w1468] -> w1455
              shift-left: w1458 -> [w1470]
              tunnel: w1448 -> [w1467] mode=indexing
              tunnel: w1457 -> [w1466] mode=indexing
              i -> [w1469]
              n539 = Wait (ms)(milliseconds to wait=u32 1000) -> ()  [unwired: 1 out]
              n540 = case shown="True" w1466 {
                tunnel: w1470 -> [w1471 w1474]
                tunnel: w1469 -> [_ _]
                tunnel: [w1471 w1473] -> w1468
                tunnel: w1467 -> [_ w1472]
                frame False {
                }
                frame True {
                  n541 = case shown="\"True\", Default" w1472 {
                    selector: w1472 -> [_ w1476]
                    tunnel: w1474 -> [w1475 w1481]
                    tunnel: [w1475 w1480] -> w1473
                    frame "" {
                    }
                    frame "True", Default {
                      n542 = call "Communication - Send Command Read.vi"("Fron?"=TRUE, "Bypass?"=TRUE, "error in (no error)"=w1481, "Action"=UDP_-_Command."Read Sensor", "Device IP Address"=w1476) -> ("error out"=w1480:errorcluster)  [unwired: 6 in]
                    }
                  }
                }
              }
            }
            n543 = Select(t=Communications_-_State."Idle", s=w1454, f=Communications_-_State."Release Rendezvous") -> (s? t:f=w1451:T2)
            n544 = flat-sequence {
              tunnel: [w1463] -> w1456
              tunnel: w1455 -> [w1463]
              tunnel: w1449 -> [w1462]
              tunnel: [w1460] -> w1450
              frame #0 {
                n545 = global write "Global - Hold.vi" "Hold"(FALSE ("Hold")) -> ()
                n546 = Bundle By Name(cluster=w1462, "Trig?"=FALSE) -> (w1460:T6)
              }
            }
          }
          frame "Release Rendezvous" {
            n547 = disable-structure shown="Disabled" {
              disable-tunnel: [w1489 w1490] -> w1483
              disable-tunnel: w1482 -> [w1488 w1490]
              frame Disabled {
                n548 = global read "Global - Rendezvous.vi" "rendezvous"() -> (w1487:T16)
                n549 = call <vilib>:"Wait at Rendezvous.vi"("error in (no error)"=w1488, "rendezvous"=w1487) -> ("error out"=w1489:errorcluster)  [unwired: 3 in, 2 out]
              }
              frame Enabled {
              }
            }
          }
          frame "Close" {
            w1494 = TRUE
            n550 = disable-structure shown="Enabled" {
              disable-tunnel: w1492 -> [w1500 w1504]
              disable-tunnel: [w1497 w1504] -> w1491
              frame Disabled {
                n551 = global read "Global - Handle V1.vi" "Handle"() -> (w1499:refnum<visa-resource-name>[])
                n552 = for {
                  tunnel: w1499 -> [w1501] mode=indexing
                  shift-right: [w1502] -> w1498
                  shift-left: w1500 -> [w1503]
                  n553 = VISA Close(VISA resource name=w1501, error in (no error)=w1503) -> (error out=w1502:errorcluster)
                }
                n554 = call <vilib>:"Clear Errors.vi"("error in (no error)"=w1498) -> ("error out"=w1497:errorcluster)  [unwired: 5 in, 1 out]
              }
              frame Enabled {
              }
            }
            "Stop" <- w1494
          }
        }
      }
      frame Error {
        n555 = Unbundle By Name(w1509) -> ("source"=w1507:string)
        n556 = Concatenate Strings("UI Loop (Comm)" ("string"), " - " ("string"), w1507) -> (w1505:string)
        n557 = Wait (ms)(milliseconds to wait=u32 100) -> ()  [unwired: 1 out]
        n558 = call <vilib>:"Clear Errors.vi"("error in (no error)"=w1509) -> ("error out"=w1511:errorcluster)  [unwired: 5 in, 1 out]
        n559 = call "General - Error Log eFGV.vi"("eFGV States"=eFGV_States."Write", "error in (no error)"=w1511, "Error In"=w1505) -> ("error out"=w1510:errorcluster)  [unwired: 6 in, 2 out]
      }
    }
    "UI loop" <- w1311
  }
  n560 = while {
    shift-right: [w1526] -> _
    shift-left: errorcluster {"status"=FALSE, "code"=0, "source"=""} ("error IO") -> [w1527]
    shift-right: [w1524] -> _
    shift-left: Communications_-_State."Init" -> [w1525]
    shift-right: [w1522] -> _
    shift-left: _ -> [w1521]
    tunnel: 1 ("index") -> [w1520]
    shift-right: [w1518] -> _
    shift-left: _ -> [w1517]
    i -> [w1519]
    stop <- w1523 stop-if-true
    # "Queue Command Processing Loop"
    n561 = case shown="No Error" w1527 {
      selector: w1527 -> [w1536 w1669]
      tunnel: [w1537 w1664] -> w1526
      tunnel: w1525 -> [w1535 _]
      tunnel: [w1534 Communications_-_State."Idle"] -> w1524
      tunnel: [w1533 _] -> w1523
      tunnel: [w1532 w1671] -> w1522
      tunnel: w1521 -> [w1531 w1671]
      tunnel: w1520 -> [w1530 w1661]
      tunnel: [w1529 w1659] -> w1518
      tunnel: w1517 -> [w1528 w1659]
      frame No Error {
        n562 = case shown="\"Command\"" w1535 {
          tunnel: [w1541 w1561 w1596 w1653] -> w1537
          tunnel: w1536 -> [w1546 w1560 w1599 w1652]
          tunnel: [Communications_-_State."Idle" w1549 Communications_-_State."Idle" Communications_-_State."Close"] -> w1534
          tunnel: [_ _ _ TRUE] -> w1533
          tunnel: [w1543 w1559 w1598 w1656] -> w1532
          tunnel: w1531 -> [_ w1558 w1598 w1656]
          tunnel: w1530 -> [_ w1553 w1585 w1651]
          tunnel: [0 w1548 w1583 0] -> w1529
          tunnel: w1528 -> [_ w1548 w1582 _]
          frame "Init", Default {
            n563 = call "Communication - UDP Command (eFGV).vi"("Action"=eFGV_States."Read", "error in"=w1546) -> ("error out"=w1542:errorcluster, "UDP Ref"=w1540:refnum<user-event>)  [unwired: 7 in, 1 out]
            n564 = register-events(error in=w1542, w1540) -> (reference out=w1539:refnum<event-registration>, error out=w1541:errorcluster)  [unwired: 1 in]
            n565 = Bundle By Name(cluster=T6 {"UDP CMD"={"IP"="", "CMD"=enum."Stop", "Port"="", "Datalog?"=FALSE, "Float"=0.0}, "Unit?"=FALSE, "Read Unit"=[], "Trig?"=FALSE, "UDP Info"=[], "DataLogger"=[], "VISA Ref"=refnum, "Float"=0.0, "Data"={"Test"={"Target Load"=0.0, "Target Disp"=0.0, "Rate"=0.0, "Speed"=0.0}, "Sensor"={"Name"=[], "Unit"=[], "Decimal Point"=[], "Ch Log"=[], "H Alarm"=[], "L Alarm"=[], "H Limit"=[], "L Limit"=[], "Filter"=[], "Gain"=[], "Calib Type"=[]}, "PID"={"SP"=-2.7823365e-08, "PV"=-3.023652e-13, "kP"=8.5432666e-24, "kI"=2.29252e-41, "kD"=1.570387e-38, "FF"=25.0, "Err Band"=0.0, "Max"=15, "Min"=-7, "Ts"=1886611780, "Out"=0, "Mode"=0}, "ADC"={"Active Ch"=[255, 255, 255, 0, 0, 0, 0, 0], "Filter Type"=2, "Post Filter"=[1, 1, 1, 1, 0, 200, 66, 184], "Gain"=[0, 0, 0, 0, 0, 122, 68, 0], "FS"=32, "IntOC"=0, "IntFC"=255, "SysOC"=255, "Cofficient"=[1.0, 1.0, 1.0, 1.0, 1.0, 1.0, 1.0, 1.0], "K"=[1.2450000047683716, 1.2450000047683716], "Max"=1048576}, "System"={"Out Type"=0, "Inverse"=0, "Monitor"=0, "Reserve"=0, "ACC Time"=0, "Pulse Rev"=0, "Stroke"=0, "Auto Off"=0, "Gear Ratio"=0.0, "Pitch"=0.0, "Max Speed"=0, "Jog Speed"=0, "Disp Coff"=0.0, "Max Load"=0}, "Index"=enum."Ch1", "Datalog"=enum."Empty"}, "UDP Event Ref"=refnum, "UDP ref"=refnum, "Read Sensor"=0}, "UDP Event Ref"=w1539) -> (w1543:T6)
          }
          frame "Idle" {
            n566 = Unbundle By Name(w1558) -> ("UDP Event Ref"=w1562:refnum<event-registration>)
            n567 = event shown="[1] <UDP Ref>: User Event" {
              selector: w1562 -> [_ _]
              dyn-events: _ -> [_ _]
              timeout: 3000 -> [_ _]
              tunnel: [w1568 w1571] -> w1556
              tunnel: [w1565 _] -> w1561
              tunnel: w1560 -> [w1565 _]
              tunnel: [w1563 w1580] -> w1559
              tunnel: w1558 -> [w1563 w1579]
              tunnel: w1553 -> [_ w1569]
              event Timeout {
                n568 = event-data() -> ()  [unwired: 1 in, 1 out]
                n569 = local read "Stop"() -> (w1567:bool)
                n570 = Select(t=Communications_-_State."Close", s=w1567, f=Communications_-_State."Idle") -> (s? t:f=w1568:T2)
              }
              event User Event {
                n571 = event-data() -> ("IP"=w1574:string, "CMD"=w1578:T1, "Data"=w1577:T7)  [unwired: 1 in]
                n572 = global read "Global - IP Address.vi" "IP"() -> (w1576:string[])
                n573 = Index Array(array=w1576, index=w1569) -> (element=w1575:string)
                n574 = Equal?(x=w1575, y=w1574) -> (x = y?=w1573:bool)
                n575 = Bundle By Name(cluster=w1579, "UDP CMD.IP"=w1574, "UDP CMD.CMD"=w1578, "Data"=w1577) -> (w1580:T6)
                n576 = Select(t=Communications_-_State."Command" ("f"), s=w1573, f=Communications_-_State."Idle") -> (s? t:f=w1571:T2)
              }
            }
            n577 = global read "Global - Hold.vi" "Hold"() -> (w1557:bool)
            n578 = Select(t=Communications_-_State."Idle", s=w1557, f=w1556) -> (s? t:f=w1550:T2)
            n579 = local read "Stop"() -> (w1551:bool)
            n580 = Select(t=Communications_-_State."Close", s=w1551, f=w1550) -> (s? t:f=w1549:T2)
          }
          frame "Command" {
            n581 = Unbundle By Name(w1598) -> ("UDP CMD.CMD"=w1595:T1, "Data"=w1597:T7, "UDP CMD.IP"=w1581:string)
            "1" <- w1595
            n582 = global read "Global - Handle V1.vi" "Handle"() -> (w1589:refnum<visa-resource-name>[])
            n583 = global read "Global - IP Address.vi" "IP"() -> (w1590:string[])
            n584 = Search 1D Array(1D array=w1590, element=w1581) -> ()  [unwired: 1 in, 1 out]
            n585 = Index Array(array=w1589, index=w1585) -> (element=w1591:refnum<visa-resource-name>)
            n586 = call "VISA - Write CMD.vi"("Index"=w1585, "error in"=w1599, "Data"=w1597, "Action"=w1595, "VISA ref"=w1591) -> ("error out"=w1587:errorcluster, "Data Unit"=w1593:T12, "Data Channel"=w1594:T13, "Success"=w1592:bool, "Prev Data?"=→"Prev 1":bool)  [unwired: 2 out]
            "Success1" <- w1592
            n587 = flat-sequence {
              tunnel: w1585 -> [w1605]
              tunnel: [w1602] -> w1588
              tunnel: w1587 -> [w1602]
              frame #0 {
                n588 = global read "Global - Done.vi" "Done"() -> (w1604:bool[])
                n589 = Replace Array Subset(array=w1604, new element=TRUE, index=w1605) -> (w1603:bool[])
                n590 = global write "Global - Done.vi" "Done"(w1603) -> ()
              }
            }
            n591 = global write "Global - Data UDP.vi" "Loop 2"(TRUE ("Loop 2")) -> ()
            n592 = case shown="False" w1592 {
              tunnel: w1588 -> [w1609 w1624]
              tunnel: [w1610 w1623] -> w1596
              tunnel: w1595 -> [_ w1625]
              tunnel: w1594 -> [_ w1622]
              tunnel: w1593 -> [_ w1621]
              tunnel: w1585 -> [_ w1620]
              tunnel: [w1606 0] -> w1583
              tunnel: w1582 -> [w1611 _]
              tunnel: w1581 -> [w1608 _]
              frame False {
                n593 = Increment(x=w1611) -> (x+1=w1607:i32)
                n594 = case shown="5" w1607 {
                  selector: w1607 -> [w1612 _]
                  tunnel: [w1613 w1617] -> w1610
                  tunnel: w1609 -> [w1613 w1616]
                  tunnel: w1608 -> [_ w1615]
                  tunnel: [w1612 0] -> w1606
                  frame 0, Default {
                  }
                  frame 5 {
                    n595 = call "Communication - Reconnect eFGV.vi"("eFGV States"=eFGV_States."Write", "error in (no error)"=w1616, "Reconnect In"=w1615) -> ("error out"=w1617:errorcluster)  [unwired: 6 in, 2 out]
                  }
                }
              }
              frame True {
                n596 = case shown="\"Read Ch Data\"" w1625 {
                  tunnel: w1624 -> [w1626 w1633 w1648]
                  tunnel: [w1626 w1633 w1648] -> w1623
                  tunnel: w1622 -> [_ w1631 _]
                  tunnel: w1621 -> [_ _ w1644]
                  tunnel: w1620 -> [_ w1635 w1649]
                  frame "Stop", Default {
                  }
                  frame "Read Ch Data" {
                    n597 = Unbundle By Name(w1631) -> ("Ch1 Data"=w1630:sgl, "Ch2 Data"=w1629:sgl)
                    n598 = global read "Global - Channel.vi" "Data"() -> (w1634:T14)
                    n599 = Bundle By Name(cluster=T10 {"Channels"={"Ch1"=0.0, "Ch2"=0.0, "Ch3"=0.0, "Ch4"=0.0, "Ch5"=0.0, "Ch6"=0.0, "Ch7"=0.0, "Ch8"=0.0, "Ch9"=0.0, "Ch10"=0.0, "Ch11"=0.0, "Ch12"=0.0, "Ch13"=0.0, "Ch14"=0.0, "Ch15"=0.0, "Ch16"=0.0}, "Event"=0, "Status"=0, "IP"=""} ("Data Channel"), "Channels.Ch1"=w1630, "Channels.Ch2"=w1629) -> (w1628:T10)
                    n600 = Replace Array Subset(array=w1634, new element=w1628, index=w1635) -> (w1632:T14)
                    n601 = global write "Global - Channel.vi" "Data"(w1632) -> ()
                  }
                  frame "Read Sensor" {
                    n602 = Unbundle By Name(w1644) -> ("Ch1 Unit"=w1643:string, "Ch2 Unit"=w1642:string, "Ch1 Decimal"=w1641:u8, "Ch2 Decimal"=w1640:u8)
                    n603 = global read "Global - Unit.vi" "Unit"() -> (w1646:T15)
                    n604 = Build Array(w1643, w1642) -> (w1639:string[])
                    n605 = Build Array(w1641, w1640) -> (w1638:u8[])
                    n606 = Bundle By Name(cluster=T11 {"Name"=[], "Unit"=[], "Decimal Point"=[], "Ch Log"=[], "H Alarm"=[], "L Alarm"=[], "H Limit"=[], "L Limit"=[], "Filter"=[], "Gain"=[], "Calib Type"=[]} ("Sensor"), "Name"=string[] ["Load", "Displacement"], "Unit"=w1639, "Decimal Point"=w1638) -> (w1637:T11)
                    n607 = Replace Array Subset(array=w1646, new element=w1637, index=w1649) -> (w1647:T15)
                    n608 = global write "Global - Unit.vi" "Unit"(w1647) -> ()
                  }
                }
              }
            }
          }
          frame "Close" {
            n609 = global read "Global - Handle V1.vi" "Handle"() -> (w1655:refnum<visa-resource-name>[])
            n610 = Index Array(array=w1655, index=w1651) -> (element=w1654:refnum<visa-resource-name>)
            n611 = VISA Close(VISA resource name=w1654, error in (no error)=w1652) -> (error out=w1653:errorcluster)
          }
        }
      }
      frame Error {
        n612 = global read "Global - IP Address.vi" "IP"() -> (w1668:string[])
        n613 = Unbundle By Name(w1669) -> ("source"=w1666:string)
        n614 = Index Array(array=w1668, index=w1661) -> (element=w1667:string)
        n615 = Concatenate Strings(w1667, " - " ("string"), w1666) -> (w1662:string)
        n616 = call <vilib>:"Clear Errors.vi"("error in (no error)"=w1669) -> ("error out"=w1665:errorcluster)  [unwired: 5 in, 1 out]
        n617 = call "General - Error Log eFGV.vi"("eFGV States"=eFGV_States."Write", "error in (no error)"=w1665, "Error In"=w1662) -> ("error out"=w1664:errorcluster)  [unwired: 6 in, 2 out]
        n618 = Wait (ms)(milliseconds to wait=u32 100) -> ()  [unwired: 1 out]
      }
    }
    "1" <- w1525
    "loop 1" <- w1519
  }
  n619 = while {
    shift-right: [w1682] -> _
    shift-left: errorcluster {"status"=FALSE, "code"=0, "source"=""} ("error IO") -> [w1683]
    shift-right: [w1680] -> _
    shift-left: Communications_-_State."Init" -> [w1681]
    shift-right: [w1678] -> _
    shift-left: _ -> [w1677]
    tunnel: 3 ("index") -> [w1676]
    shift-right: [w1674] -> _
    shift-left: _ -> [w1673]
    i -> [w1675]
    stop <- w1679 stop-if-true
    # "Queue Command Processing Loop"
    n620 = case shown="No Error" w1683 {
      selector: w1683 -> [w1692 w1825]
      tunnel: [w1693 w1819] -> w1682
      tunnel: w1681 -> [w1691 _]
      tunnel: [w1690 Communications_-_State."Idle"] -> w1680
      tunnel: [w1689 _] -> w1679
      tunnel: [w1688 w1827] -> w1678
      tunnel: w1677 -> [w1687 w1827]
      tunnel: w1676 -> [w1686 w1816]
      tunnel: [w1685 w1815] -> w1674
      tunnel: w1673 -> [w1684 w1815]
      frame No Error {
        n621 = case shown="\"Command\"" w1691 {
          tunnel: [w1697 w1717 w1752 w1809] -> w1693
          tunnel: w1692 -> [w1702 w1716 w1755 w1808]
          tunnel: [Communications_-_State."Idle" w1705 Communications_-_State."Idle" Communications_-_State."Close"] -> w1690
          tunnel: [_ _ _ TRUE] -> w1689
          tunnel: [w1699 w1715 w1754 w1812] -> w1688
          tunnel: w1687 -> [_ w1714 w1754 w1812]
          tunnel: w1686 -> [_ w1709 w1741 w1807]
          tunnel: [0 w1704 w1739 0] -> w1685
          tunnel: w1684 -> [_ w1704 w1738 _]
          frame "Init", Default {
            n622 = call "Communication - UDP Command (eFGV).vi"("Action"=eFGV_States."Read", "error in"=w1702) -> ("error out"=w1698:errorcluster, "UDP Ref"=w1696:refnum<user-event>)  [unwired: 7 in, 1 out]
            n623 = register-events(error in=w1698, w1696) -> (reference out=w1695:refnum<event-registration>, error out=w1697:errorcluster)  [unwired: 1 in]
            n624 = Bundle By Name(cluster=T6 {"UDP CMD"={"IP"="", "CMD"=enum."Stop", "Port"="", "Datalog?"=FALSE, "Float"=0.0}, "Unit?"=FALSE, "Read Unit"=[], "Trig?"=FALSE, "UDP Info"=[], "DataLogger"=[], "VISA Ref"=refnum, "Float"=0.0, "Data"={"Test"={"Target Load"=0.0, "Target Disp"=0.0, "Rate"=0.0, "Speed"=0.0}, "Sensor"={"Name"=[], "Unit"=[], "Decimal Point"=[], "Ch Log"=[], "H Alarm"=[], "L Alarm"=[], "H Limit"=[], "L Limit"=[], "Filter"=[], "Gain"=[], "Calib Type"=[]}, "PID"={"SP"=-2.7823365e-08, "PV"=-3.023652e-13, "kP"=8.5432666e-24, "kI"=2.29252e-41, "kD"=1.570387e-38, "FF"=25.0, "Err Band"=0.0, "Max"=15, "Min"=-7, "Ts"=1886611780, "Out"=0, "Mode"=0}, "ADC"={"Active Ch"=[255, 255, 255, 0, 0, 0, 0, 0], "Filter Type"=2, "Post Filter"=[1, 1, 1, 1, 0, 200, 66, 184], "Gain"=[0, 0, 0, 0, 0, 122, 68, 0], "FS"=32, "IntOC"=0, "IntFC"=255, "SysOC"=255, "Cofficient"=[1.0, 1.0, 1.0, 1.0, 1.0, 1.0, 1.0, 1.0], "K"=[1.2450000047683716, 1.2450000047683716], "Max"=1048576}, "System"={"Out Type"=0, "Inverse"=0, "Monitor"=0, "Reserve"=0, "ACC Time"=0, "Pulse Rev"=0, "Stroke"=0, "Auto Off"=0, "Gear Ratio"=0.0, "Pitch"=0.0, "Max Speed"=0, "Jog Speed"=0, "Disp Coff"=0.0, "Max Load"=0}, "Index"=enum."Ch1", "Datalog"=enum."Empty"}, "UDP Event Ref"=refnum, "UDP ref"=refnum, "Read Sensor"=0}, "UDP Event Ref"=w1695) -> (w1699:T6)
          }
          frame "Idle" {
            n625 = Unbundle By Name(w1714) -> ("UDP Event Ref"=w1718:refnum<event-registration>)
            n626 = event shown="[0] Timeout" {
              selector: w1718 -> [_ _]
              dyn-events: _ -> [_ _]
              timeout: 3000 -> [_ _]
              tunnel: [w1724 w1727] -> w1712
              tunnel: [w1721 _] -> w1717
              tunnel: w1716 -> [w1721 _]
              tunnel: [w1719 w1736] -> w1715
              tunnel: w1714 -> [w1719 w1735]
              tunnel: w1709 -> [_ w1725]
              event Timeout {
                n627 = event-data() -> ()  [unwired: 1 in, 1 out]
                n628 = local read "Stop"() -> (w1723:bool)
                n629 = Select(t=Communications_-_State."Close", s=w1723, f=Communications_-_State."Idle") -> (s? t:f=w1724:T2)
              }
              event User Event {
                n630 = event-data() -> ("IP"=w1730:string, "CMD"=w1734:T1, "Data"=w1733:T7)  [unwired: 1 in]
                n631 = global read "Global - IP Address.vi" "IP"() -> (w1732:string[])
                n632 = Index Array(array=w1732, index=w1725) -> (element=w1731:string)
                n633 = Equal?(x=w1731, y=w1730) -> (x = y?=w1729:bool)
                n634 = Bundle By Name(cluster=w1735, "UDP CMD.IP"=w1730, "UDP CMD.CMD"=w1734, "Data"=w1733) -> (w1736:T6)
                n635 = Select(t=Communications_-_State."Command" ("f"), s=w1729, f=Communications_-_State."Idle") -> (s? t:f=w1727:T2)
              }
            }
            n636 = global read "Global - Hold.vi" "Hold"() -> (w1713:bool)
            n637 = Select(t=Communications_-_State."Idle", s=w1713, f=w1712) -> (s? t:f=w1706:T2)
            n638 = local read "Stop"() -> (w1707:bool)
            n639 = Select(t=Communications_-_State."Close", s=w1707, f=w1706) -> (s? t:f=w1705:T2)
          }
          frame "Command" {
            n640 = Unbundle By Name(w1754) -> ("UDP CMD.CMD"=w1751:T1, "Data"=w1753:T7, "UDP CMD.IP"=w1737:string)
            "3" <- w1751
            n641 = global read "Global - Handle V1.vi" "Handle"() -> (w1745:refnum<visa-resource-name>[])
            n642 = global read "Global - IP Address.vi" "IP"() -> (w1746:string[])
            n643 = Search 1D Array(1D array=w1746, element=w1737) -> ()  [unwired: 1 in, 1 out]
            n644 = Index Array(array=w1745, index=w1741) -> (element=w1747:refnum<visa-resource-name>)
            n645 = call "VISA - Write CMD.vi"("Index"=w1741, "error in"=w1755, "Data"=w1753, "Action"=w1751, "VISA ref"=w1747) -> ("error out"=w1743:errorcluster, "Data Unit"=w1749:T12, "Data Channel"=w1750:T13, "Success"=w1748:bool, "Prev Data?"=→"Prev 3":bool)  [unwired: 2 out]
            "Success3" <- w1748
            n646 = flat-sequence {
              tunnel: w1741 -> [w1761]
              tunnel: [w1758] -> w1744
              tunnel: w1743 -> [w1758]
              frame #0 {
                n647 = global read "Global - Done.vi" "Done"() -> (w1760:bool[])
                n648 = Replace Array Subset(array=w1760, new element=TRUE, index=w1761) -> (w1759:bool[])
                n649 = global write "Global - Done.vi" "Done"(w1759) -> ()
              }
            }
            n650 = global write "Global - Data UDP.vi" "Loop 4"(TRUE ("Loop 4")) -> ()
            n651 = case shown="False" w1748 {
              tunnel: w1744 -> [w1765 w1780]
              tunnel: [w1766 w1779] -> w1752
              tunnel: w1751 -> [_ w1781]
              tunnel: w1750 -> [_ w1778]
              tunnel: w1749 -> [_ w1777]
              tunnel: w1741 -> [_ w1776]
              tunnel: [w1762 0] -> w1739
              tunnel: w1738 -> [w1767 _]
              tunnel: w1737 -> [w1764 _]
              frame False {
                n652 = Increment(x=w1767) -> (x+1=w1763:i32)
                n653 = case shown="5" w1763 {
                  selector: w1763 -> [w1768 _]
                  tunnel: [w1769 w1773] -> w1766
                  tunnel: w1765 -> [w1769 w1772]
                  tunnel: w1764 -> [_ w1771]
                  tunnel: [w1768 0] -> w1762
                  frame 0, Default {
                  }
                  frame 5 {
                    n654 = call "Communication - Reconnect eFGV.vi"("eFGV States"=eFGV_States."Write", "error in (no error)"=w1772, "Reconnect In"=w1771) -> ("error out"=w1773:errorcluster)  [unwired: 6 in, 2 out]
                  }
                }
              }
              frame True {
                n655 = case shown="\"Read Ch Data\"" w1781 {
                  tunnel: w1780 -> [w1782 w1789 w1804]
                  tunnel: [w1782 w1789 w1804] -> w1779
                  tunnel: w1778 -> [_ w1787 _]
                  tunnel: w1777 -> [_ _ w1800]
                  tunnel: w1776 -> [_ w1791 w1805]
                  frame "Stop", Default {
                  }
                  frame "Read Ch Data" {
                    n656 = Unbundle By Name(w1787) -> ("Ch1 Data"=w1786:sgl, "Ch2 Data"=w1785:sgl)
                    n657 = global read "Global - Channel.vi" "Data"() -> (w1790:T14)
                    n658 = Bundle By Name(cluster=T10 {"Channels"={"Ch1"=0.0, "Ch2"=0.0, "Ch3"=0.0, "Ch4"=0.0, "Ch5"=0.0, "Ch6"=0.0, "Ch7"=0.0, "Ch8"=0.0, "Ch9"=0.0, "Ch10"=0.0, "Ch11"=0.0, "Ch12"=0.0, "Ch13"=0.0, "Ch14"=0.0, "Ch15"=0.0, "Ch16"=0.0}, "Event"=0, "Status"=0, "IP"=""} ("Data Channel"), "Channels.Ch1"=w1786, "Channels.Ch2"=w1785) -> (w1784:T10)
                    n659 = Replace Array Subset(array=w1790, new element=w1784, index=w1791) -> (w1788:T14)
                    n660 = global write "Global - Channel.vi" "Data"(w1788) -> ()
                  }
                  frame "Read Sensor" {
                    n661 = Unbundle By Name(w1800) -> ("Ch1 Unit"=w1799:string, "Ch2 Unit"=w1798:string, "Ch1 Decimal"=w1797:u8, "Ch2 Decimal"=w1796:u8)
                    n662 = global read "Global - Unit.vi" "Unit"() -> (w1802:T15)
                    n663 = Build Array(w1799, w1798) -> (w1795:string[])
                    n664 = Build Array(w1797, w1796) -> (w1794:u8[])
                    n665 = Bundle By Name(cluster=T11 {"Name"=[], "Unit"=[], "Decimal Point"=[], "Ch Log"=[], "H Alarm"=[], "L Alarm"=[], "H Limit"=[], "L Limit"=[], "Filter"=[], "Gain"=[], "Calib Type"=[]} ("Sensor"), "Name"=string[] ["Load", "Displacement"], "Unit"=w1795, "Decimal Point"=w1794) -> (w1793:T11)
                    n666 = Replace Array Subset(array=w1802, new element=w1793, index=w1805) -> (w1803:T15)
                    n667 = global write "Global - Unit.vi" "Unit"(w1803) -> ()
                  }
                }
              }
            }
          }
          frame "Close" {
            n668 = global read "Global - Handle V1.vi" "Handle"() -> (w1811:refnum<visa-resource-name>[])
            n669 = Index Array(array=w1811, index=w1807) -> (element=w1810:refnum<visa-resource-name>)
            n670 = VISA Close(VISA resource name=w1810, error in (no error)=w1808) -> (error out=w1809:errorcluster)
          }
        }
      }
      frame Error {
        n671 = global read "Global - IP Address.vi" "IP"() -> (w1824:string[])
        n672 = Unbundle By Name(w1825) -> ("source"=w1821:string)
        n673 = Index Array(array=w1824, index=w1816) -> (element=w1823:string)
        n674 = Concatenate Strings(w1823, " - " ("string"), w1821) -> (w1817:string)
        n675 = call <vilib>:"Clear Errors.vi"("error in (no error)"=w1825) -> ("error out"=w1820:errorcluster)  [unwired: 5 in, 1 out]
        n676 = call "General - Error Log eFGV.vi"("eFGV States"=eFGV_States."Write", "error in (no error)"=w1820, "Error In"=w1817) -> ("error out"=w1819:errorcluster)  [unwired: 6 in, 2 out]
        n677 = Wait (ms)(milliseconds to wait=u32 100) -> ()  [unwired: 1 out]
      }
    }
    "3" <- w1681
    "loop 3" <- w1675
  }
  n678 = while {
    shift-right: [w1838] -> _
    shift-left: errorcluster {"status"=FALSE, "code"=0, "source"=""} ("error IO") -> [w1839]
    shift-right: [w1836] -> _
    shift-left: Communications_-_State."Init" -> [w1837]
    shift-right: [w1834] -> _
    shift-left: _ -> [w1833]
    tunnel: 5 ("index") -> [w1832]
    shift-right: [w1830] -> _
    shift-left: _ -> [w1829]
    i -> [w1831]
    stop <- w1835 stop-if-true
    # "Queue Command Processing Loop"
    n679 = case shown="No Error" w1839 {
      selector: w1839 -> [w1848 w1981]
      tunnel: [w1849 w1976] -> w1838
      tunnel: w1837 -> [w1847 _]
      tunnel: [w1846 Communications_-_State."Idle"] -> w1836
      tunnel: [w1845 _] -> w1835
      tunnel: [w1844 w1983] -> w1834
      tunnel: w1833 -> [w1843 w1983]
      tunnel: w1832 -> [w1842 w1973]
      tunnel: [w1841 w1971] -> w1830
      tunnel: w1829 -> [w1840 w1971]
      frame No Error {
        n680 = case shown="\"Command\"" w1847 {
          tunnel: [w1853 w1873 w1908 w1965] -> w1849
          tunnel: w1848 -> [w1858 w1872 w1911 w1964]
          tunnel: [Communications_-_State."Idle" w1861 Communications_-_State."Idle" Communications_-_State."Close"] -> w1846
          tunnel: [_ _ _ TRUE] -> w1845
          tunnel: [w1855 w1871 w1910 w1968] -> w1844
          tunnel: w1843 -> [_ w1870 w1910 w1968]
          tunnel: w1842 -> [_ w1865 w1897 w1963]
          tunnel: [0 w1860 w1895 0] -> w1841
          tunnel: w1840 -> [_ w1860 w1894 _]
          frame "Init", Default {
            n681 = call "Communication - UDP Command (eFGV).vi"("Action"=eFGV_States."Read", "error in"=w1858) -> ("error out"=w1854:errorcluster, "UDP Ref"=w1852:refnum<user-event>)  [unwired: 7 in, 1 out]
            n682 = register-events(error in=w1854, w1852) -> (reference out=w1851:refnum<event-registration>, error out=w1853:errorcluster)  [unwired: 1 in]
            n683 = Bundle By Name(cluster=T6 {"UDP CMD"={"IP"="", "CMD"=enum."Stop", "Port"="", "Datalog?"=FALSE, "Float"=0.0}, "Unit?"=FALSE, "Read Unit"=[], "Trig?"=FALSE, "UDP Info"=[], "DataLogger"=[], "VISA Ref"=refnum, "Float"=0.0, "Data"={"Test"={"Target Load"=0.0, "Target Disp"=0.0, "Rate"=0.0, "Speed"=0.0}, "Sensor"={"Name"=[], "Unit"=[], "Decimal Point"=[], "Ch Log"=[], "H Alarm"=[], "L Alarm"=[], "H Limit"=[], "L Limit"=[], "Filter"=[], "Gain"=[], "Calib Type"=[]}, "PID"={"SP"=-2.7823365e-08, "PV"=-3.023652e-13, "kP"=8.5432666e-24, "kI"=2.29252e-41, "kD"=1.570387e-38, "FF"=25.0, "Err Band"=0.0, "Max"=15, "Min"=-7, "Ts"=1886611780, "Out"=0, "Mode"=0}, "ADC"={"Active Ch"=[255, 255, 255, 0, 0, 0, 0, 0], "Filter Type"=2, "Post Filter"=[1, 1, 1, 1, 0, 200, 66, 184], "Gain"=[0, 0, 0, 0, 0, 122, 68, 0], "FS"=32, "IntOC"=0, "IntFC"=255, "SysOC"=255, "Cofficient"=[1.0, 1.0, 1.0, 1.0, 1.0, 1.0, 1.0, 1.0], "K"=[1.2450000047683716, 1.2450000047683716], "Max"=1048576}, "System"={"Out Type"=0, "Inverse"=0, "Monitor"=0, "Reserve"=0, "ACC Time"=0, "Pulse Rev"=0, "Stroke"=0, "Auto Off"=0, "Gear Ratio"=0.0, "Pitch"=0.0, "Max Speed"=0, "Jog Speed"=0, "Disp Coff"=0.0, "Max Load"=0}, "Index"=enum."Ch1", "Datalog"=enum."Empty"}, "UDP Event Ref"=refnum, "UDP ref"=refnum, "Read Sensor"=0}, "UDP Event Ref"=w1851) -> (w1855:T6)
          }
          frame "Idle" {
            n684 = Unbundle By Name(w1870) -> ("UDP Event Ref"=w1874:refnum<event-registration>)
            n685 = event shown="[1] <UDP Ref>: User Event" {
              selector: w1874 -> [_ _]
              dyn-events: _ -> [_ _]
              timeout: 3000 -> [_ _]
              tunnel: [w1880 w1883] -> w1868
              tunnel: [w1877 _] -> w1873
              tunnel: w1872 -> [w1877 _]
              tunnel: [w1875 w1892] -> w1871
              tunnel: w1870 -> [w1875 w1891]
              tunnel: w1865 -> [_ w1881]
              event Timeout {
                n686 = event-data() -> ()  [unwired: 1 in, 1 out]
                n687 = local read "Stop"() -> (w1879:bool)
                n688 = Select(t=Communications_-_State."Close", s=w1879, f=Communications_-_State."Idle") -> (s? t:f=w1880:T2)
              }
              event User Event {
                n689 = event-data() -> ("IP"=w1886:string, "CMD"=w1890:T1, "Data"=w1889:T7)  [unwired: 1 in]
                n690 = global read "Global - IP Address.vi" "IP"() -> (w1888:string[])
                n691 = Index Array(array=w1888, index=w1881) -> (element=w1887:string)
                n692 = Equal?(x=w1887, y=w1886) -> (x = y?=w1885:bool)
                n693 = Bundle By Name(cluster=w1891, "UDP CMD.IP"=w1886, "UDP CMD.CMD"=w1890, "Data"=w1889) -> (w1892:T6)
                n694 = Select(t=Communications_-_State."Command" ("f"), s=w1885, f=Communications_-_State."Idle") -> (s? t:f=w1883:T2)
              }
            }
            n695 = global read "Global - Hold.vi" "Hold"() -> (w1869:bool)
            n696 = Select(t=Communications_-_State."Idle", s=w1869, f=w1868) -> (s? t:f=w1862:T2)
            n697 = local read "Stop"() -> (w1863:bool)
            n698 = Select(t=Communications_-_State."Close", s=w1863, f=w1862) -> (s? t:f=w1861:T2)
          }
          frame "Command" {
            n699 = Unbundle By Name(w1910) -> ("UDP CMD.CMD"=w1907:T1, "Data"=w1909:T7, "UDP CMD.IP"=w1893:string)
            "5" <- w1907
            n700 = global read "Global - Handle V1.vi" "Handle"() -> (w1901:refnum<visa-resource-name>[])
            n701 = global read "Global - IP Address.vi" "IP"() -> (w1902:string[])
            n702 = Search 1D Array(1D array=w1902, element=w1893) -> ()  [unwired: 1 in, 1 out]
            n703 = Index Array(array=w1901, index=w1897) -> (element=w1903:refnum<visa-resource-name>)
            n704 = call "VISA - Write CMD.vi"("Index"=w1897, "error in"=w1911, "Data"=w1909, "Action"=w1907, "VISA ref"=w1903) -> ("error out"=w1899:errorcluster, "Data Unit"=w1905:T12, "Data Channel"=w1906:T13, "Success"=w1904:bool, "Prev Data?"=→"Prev 5":bool)  [unwired: 2 out]
            "Success5" <- w1904
            n705 = flat-sequence {
              tunnel: w1897 -> [w1917]
              tunnel: [w1914] -> w1900
              tunnel: w1899 -> [w1914]
              frame #0 {
                n706 = global read "Global - Done.vi" "Done"() -> (w1916:bool[])
                n707 = Replace Array Subset(array=w1916, new element=TRUE, index=w1917) -> (w1915:bool[])
                n708 = global write "Global - Done.vi" "Done"(w1915) -> ()
              }
            }
            n709 = global write "Global - Data UDP.vi" "Loop 6"(TRUE ("Loop 2")) -> ()
            n710 = case shown="False" w1904 {
              tunnel: w1900 -> [w1921 w1936]
              tunnel: [w1922 w1935] -> w1908
              tunnel: w1907 -> [_ w1937]
              tunnel: w1906 -> [_ w1934]
              tunnel: w1905 -> [_ w1933]
              tunnel: w1897 -> [_ w1932]
              tunnel: [w1918 0] -> w1895
              tunnel: w1894 -> [w1923 _]
              tunnel: w1893 -> [w1920 _]
              frame False {
                n711 = Increment(x=w1923) -> (x+1=w1919:i32)
                n712 = case shown="5" w1919 {
                  selector: w1919 -> [w1924 _]
                  tunnel: [w1925 w1929] -> w1922
                  tunnel: w1921 -> [w1925 w1928]
                  tunnel: w1920 -> [_ w1927]
                  tunnel: [w1924 0] -> w1918
                  frame 0, Default {
                  }
                  frame 5 {
                    n713 = call "Communication - Reconnect eFGV.vi"("eFGV States"=eFGV_States."Write", "error in (no error)"=w1928, "Reconnect In"=w1927) -> ("error out"=w1929:errorcluster)  [unwired: 6 in, 2 out]
                  }
                }
              }
              frame True {
                n714 = case shown="\"Read Ch Data\"" w1937 {
                  tunnel: w1936 -> [w1938 w1945 w1960]
                  tunnel: [w1938 w1945 w1960] -> w1935
                  tunnel: w1934 -> [_ w1943 _]
                  tunnel: w1933 -> [_ _ w1956]
                  tunnel: w1932 -> [_ w1947 w1961]
                  frame "Stop", Default {
                  }
                  frame "Read Ch Data" {
                    n715 = Unbundle By Name(w1943) -> ("Ch1 Data"=w1942:sgl, "Ch2 Data"=w1941:sgl)
                    n716 = global read "Global - Channel.vi" "Data"() -> (w1946:T14)
                    n717 = Bundle By Name(cluster=T10 {"Channels"={"Ch1"=0.0, "Ch2"=0.0, "Ch3"=0.0, "Ch4"=0.0, "Ch5"=0.0, "Ch6"=0.0, "Ch7"=0.0, "Ch8"=0.0, "Ch9"=0.0, "Ch10"=0.0, "Ch11"=0.0, "Ch12"=0.0, "Ch13"=0.0, "Ch14"=0.0, "Ch15"=0.0, "Ch16"=0.0}, "Event"=0, "Status"=0, "IP"=""} ("Data Channel"), "Channels.Ch1"=w1942, "Channels.Ch2"=w1941) -> (w1940:T10)
                    n718 = Replace Array Subset(array=w1946, new element=w1940, index=w1947) -> (w1944:T14)
                    n719 = global write "Global - Channel.vi" "Data"(w1944) -> ()
                  }
                  frame "Read Sensor" {
                    n720 = Unbundle By Name(w1956) -> ("Ch1 Unit"=w1955:string, "Ch2 Unit"=w1954:string, "Ch1 Decimal"=w1953:u8, "Ch2 Decimal"=w1952:u8)
                    n721 = global read "Global - Unit.vi" "Unit"() -> (w1958:T15)
                    n722 = Build Array(w1955, w1954) -> (w1951:string[])
                    n723 = Build Array(w1953, w1952) -> (w1950:u8[])
                    n724 = Bundle By Name(cluster=T11 {"Name"=[], "Unit"=[], "Decimal Point"=[], "Ch Log"=[], "H Alarm"=[], "L Alarm"=[], "H Limit"=[], "L Limit"=[], "Filter"=[], "Gain"=[], "Calib Type"=[]} ("Sensor"), "Name"=string[] ["Load", "Displacement"], "Unit"=w1951, "Decimal Point"=w1950) -> (w1949:T11)
                    n725 = Replace Array Subset(array=w1958, new element=w1949, index=w1961) -> (w1959:T15)
                    n726 = global write "Global - Unit.vi" "Unit"(w1959) -> ()
                  }
                }
              }
            }
          }
          frame "Close" {
            n727 = global read "Global - Handle V1.vi" "Handle"() -> (w1967:refnum<visa-resource-name>[])
            n728 = Index Array(array=w1967, index=w1963) -> (element=w1966:refnum<visa-resource-name>)
            n729 = VISA Close(VISA resource name=w1966, error in (no error)=w1964) -> (error out=w1965:errorcluster)
          }
        }
      }
      frame Error {
        n730 = global read "Global - IP Address.vi" "IP"() -> (w1980:string[])
        n731 = Unbundle By Name(w1981) -> ("source"=w1978:string)
        n732 = Index Array(array=w1980, index=w1973) -> (element=w1979:string)
        n733 = Concatenate Strings(w1979, " - " ("string"), w1978) -> (w1974:string)
        n734 = call <vilib>:"Clear Errors.vi"("error in (no error)"=w1981) -> ("error out"=w1977:errorcluster)  [unwired: 5 in, 1 out]
        n735 = call "General - Error Log eFGV.vi"("eFGV States"=eFGV_States."Write", "error in (no error)"=w1977, "Error In"=w1974) -> ("error out"=w1976:errorcluster)  [unwired: 6 in, 2 out]
        n736 = Wait (ms)(milliseconds to wait=u32 100) -> ()  [unwired: 1 out]
      }
    }
    "5" <- w1837
    "loop 5" <- w1831
  }
  n737 = while {
    shift-right: [w1994] -> _
    shift-left: errorcluster {"status"=FALSE, "code"=0, "source"=""} ("error IO") -> [w1995]
    shift-right: [w1992] -> _
    shift-left: Communications_-_State."Init" -> [w1993]
    shift-right: [w1990] -> _
    shift-left: _ -> [w1989]
    tunnel: 7 ("index") -> [w1988]
    shift-right: [w1986] -> _
    shift-left: _ -> [w1985]
    i -> [w1987]
    stop <- w1991 stop-if-true
    # "Queue Command Processing Loop"
    n738 = case shown="No Error" w1995 {
      selector: w1995 -> [w2004 w2137]
      tunnel: [w2005 w2131] -> w1994
      tunnel: w1993 -> [w2003 _]
      tunnel: [w2002 Communications_-_State."Idle"] -> w1992
      tunnel: [w2001 _] -> w1991
      tunnel: [w2000 w2139] -> w1990
      tunnel: w1989 -> [w1999 w2139]
      tunnel: w1988 -> [w1998 w2128]
      tunnel: [w1997 w2127] -> w1986
      tunnel: w1985 -> [w1996 w2127]
      frame No Error {
        n739 = case shown="\"Command\"" w2003 {
          tunnel: [w2009 w2029 w2064 w2121] -> w2005
          tunnel: w2004 -> [w2014 w2028 w2067 w2120]
          tunnel: [Communications_-_State."Idle" w2017 Communications_-_State."Idle" Communications_-_State."Close"] -> w2002
          tunnel: [_ _ _ TRUE] -> w2001
          tunnel: [w2011 w2027 w2066 w2124] -> w2000
          tunnel: w1999 -> [_ w2026 w2066 w2124]
          tunnel: w1998 -> [_ w2021 w2053 w2119]
          tunnel: [0 w2016 w2051 0] -> w1997
          tunnel: w1996 -> [_ w2016 w2050 _]
          frame "Init", Default {
            n740 = call "Communication - UDP Command (eFGV).vi"("Action"=eFGV_States."Read", "error in"=w2014) -> ("error out"=w2010:errorcluster, "UDP Ref"=w2008:refnum<user-event>)  [unwired: 7 in, 1 out]
            n741 = register-events(error in=w2010, w2008) -> (reference out=w2007:refnum<event-registration>, error out=w2009:errorcluster)  [unwired: 1 in]
            n742 = Bundle By Name(cluster=T6 {"UDP CMD"={"IP"="", "CMD"=enum."Stop", "Port"="", "Datalog?"=FALSE, "Float"=0.0}, "Unit?"=FALSE, "Read Unit"=[], "Trig?"=FALSE, "UDP Info"=[], "DataLogger"=[], "VISA Ref"=refnum, "Float"=0.0, "Data"={"Test"={"Target Load"=0.0, "Target Disp"=0.0, "Rate"=0.0, "Speed"=0.0}, "Sensor"={"Name"=[], "Unit"=[], "Decimal Point"=[], "Ch Log"=[], "H Alarm"=[], "L Alarm"=[], "H Limit"=[], "L Limit"=[], "Filter"=[], "Gain"=[], "Calib Type"=[]}, "PID"={"SP"=-2.7823365e-08, "PV"=-3.023652e-13, "kP"=8.5432666e-24, "kI"=2.29252e-41, "kD"=1.570387e-38, "FF"=25.0, "Err Band"=0.0, "Max"=15, "Min"=-7, "Ts"=1886611780, "Out"=0, "Mode"=0}, "ADC"={"Active Ch"=[255, 255, 255, 0, 0, 0, 0, 0], "Filter Type"=2, "Post Filter"=[1, 1, 1, 1, 0, 200, 66, 184], "Gain"=[0, 0, 0, 0, 0, 122, 68, 0], "FS"=32, "IntOC"=0, "IntFC"=255, "SysOC"=255, "Cofficient"=[1.0, 1.0, 1.0, 1.0, 1.0, 1.0, 1.0, 1.0], "K"=[1.2450000047683716, 1.2450000047683716], "Max"=1048576}, "System"={"Out Type"=0, "Inverse"=0, "Monitor"=0, "Reserve"=0, "ACC Time"=0, "Pulse Rev"=0, "Stroke"=0, "Auto Off"=0, "Gear Ratio"=0.0, "Pitch"=0.0, "Max Speed"=0, "Jog Speed"=0, "Disp Coff"=0.0, "Max Load"=0}, "Index"=enum."Ch1", "Datalog"=enum."Empty"}, "UDP Event Ref"=refnum, "UDP ref"=refnum, "Read Sensor"=0}, "UDP Event Ref"=w2007) -> (w2011:T6)
          }
          frame "Idle" {
            n743 = Unbundle By Name(w2026) -> ("UDP Event Ref"=w2030:refnum<event-registration>)
            n744 = event shown="[0] Timeout" {
              selector: w2030 -> [_ _]
              dyn-events: _ -> [_ _]
              timeout: 3000 -> [_ _]
              tunnel: [w2036 w2039] -> w2024
              tunnel: [w2033 _] -> w2029
              tunnel: w2028 -> [w2033 _]
              tunnel: [w2031 w2048] -> w2027
              tunnel: w2026 -> [w2031 w2047]
              tunnel: w2021 -> [_ w2037]
              event Timeout {
                n745 = event-data() -> ()  [unwired: 1 in, 1 out]
                n746 = local read "Stop"() -> (w2035:bool)
                n747 = Select(t=Communications_-_State."Close", s=w2035, f=Communications_-_State."Idle") -> (s? t:f=w2036:T2)
              }
              event User Event {
                n748 = event-data() -> ("IP"=w2042:string, "CMD"=w2046:T1, "Data"=w2045:T7)  [unwired: 1 in]
                n749 = global read "Global - IP Address.vi" "IP"() -> (w2044:string[])
                n750 = Index Array(array=w2044, index=w2037) -> (element=w2043:string)
                n751 = Equal?(x=w2043, y=w2042) -> (x = y?=w2041:bool)
                n752 = Bundle By Name(cluster=w2047, "UDP CMD.IP"=w2042, "UDP CMD.CMD"=w2046, "Data"=w2045) -> (w2048:T6)
                n753 = Select(t=Communications_-_State."Command" ("f"), s=w2041, f=Communications_-_State."Idle") -> (s? t:f=w2039:T2)
              }
            }
            n754 = global read "Global - Hold.vi" "Hold"() -> (w2025:bool)
            n755 = Select(t=Communications_-_State."Idle", s=w2025, f=w2024) -> (s? t:f=w2018:T2)
            n756 = local read "Stop"() -> (w2019:bool)
            n757 = Select(t=Communications_-_State."Close", s=w2019, f=w2018) -> (s? t:f=w2017:T2)
          }
          frame "Command" {
            n758 = Unbundle By Name(w2066) -> ("UDP CMD.CMD"=w2063:T1, "Data"=w2065:T7, "UDP CMD.IP"=w2049:string)
            "7" <- w2063
            n759 = global read "Global - Handle V1.vi" "Handle"() -> (w2057:refnum<visa-resource-name>[])
            n760 = global read "Global - IP Address.vi" "IP"() -> (w2058:string[])
            n761 = Search 1D Array(1D array=w2058, element=w2049) -> ()  [unwired: 1 in, 1 out]
            n762 = Index Array(array=w2057, index=w2053) -> (element=w2059:refnum<visa-resource-name>)
            n763 = call "VISA - Write CMD.vi"("Index"=w2053, "error in"=w2067, "Data"=w2065, "Action"=w2063, "VISA ref"=w2059) -> ("error out"=w2055:errorcluster, "Data Unit"=w2061:T12, "Data Channel"=w2062:T13, "Success"=w2060:bool, "Prev Data?"=→"Prev 7":bool)  [unwired: 2 out]
            "Success7" <- w2060
            n764 = flat-sequence {
              tunnel: w2053 -> [w2073]
              tunnel: [w2070] -> w2056
              tunnel: w2055 -> [w2070]
              frame #0 {
                n765 = global read "Global - Done.vi" "Done"() -> (w2072:bool[])
                n766 = Replace Array Subset(array=w2072, new element=TRUE, index=w2073) -> (w2071:bool[])
                n767 = global write "Global - Done.vi" "Done"(w2071) -> ()
              }
            }
            n768 = global write "Global - Data UDP.vi" "Loop 8"(TRUE ("Loop 4")) -> ()
            n769 = case shown="False" w2060 {
              tunnel: w2056 -> [w2077 w2092]
              tunnel: [w2078 w2091] -> w2064
              tunnel: w2063 -> [_ w2093]
              tunnel: w2062 -> [_ w2090]
              tunnel: w2061 -> [_ w2089]
              tunnel: w2053 -> [_ w2088]
              tunnel: [w2074 0] -> w2051
              tunnel: w2050 -> [w2079 _]
              tunnel: w2049 -> [w2076 _]
              frame False {
                n770 = Increment(x=w2079) -> (x+1=w2075:i32)
                n771 = case shown="5" w2075 {
                  selector: w2075 -> [w2080 _]
                  tunnel: [w2081 w2085] -> w2078
                  tunnel: w2077 -> [w2081 w2084]
                  tunnel: w2076 -> [_ w2083]
                  tunnel: [w2080 0] -> w2074
                  frame 0, Default {
                  }
                  frame 5 {
                    n772 = call "Communication - Reconnect eFGV.vi"("eFGV States"=eFGV_States."Write", "error in (no error)"=w2084, "Reconnect In"=w2083) -> ("error out"=w2085:errorcluster)  [unwired: 6 in, 2 out]
                  }
                }
              }
              frame True {
                n773 = case shown="\"Read Ch Data\"" w2093 {
                  tunnel: w2092 -> [w2094 w2101 w2116]
                  tunnel: [w2094 w2101 w2116] -> w2091
                  tunnel: w2090 -> [_ w2099 _]
                  tunnel: w2089 -> [_ _ w2112]
                  tunnel: w2088 -> [_ w2103 w2117]
                  frame "Stop", Default {
                  }
                  frame "Read Ch Data" {
                    n774 = Unbundle By Name(w2099) -> ("Ch1 Data"=w2098:sgl, "Ch2 Data"=w2097:sgl)
                    n775 = global read "Global - Channel.vi" "Data"() -> (w2102:T14)
                    n776 = Bundle By Name(cluster=T10 {"Channels"={"Ch1"=0.0, "Ch2"=0.0, "Ch3"=0.0, "Ch4"=0.0, "Ch5"=0.0, "Ch6"=0.0, "Ch7"=0.0, "Ch8"=0.0, "Ch9"=0.0, "Ch10"=0.0, "Ch11"=0.0, "Ch12"=0.0, "Ch13"=0.0, "Ch14"=0.0, "Ch15"=0.0, "Ch16"=0.0}, "Event"=0, "Status"=0, "IP"=""} ("Data Channel"), "Channels.Ch1"=w2098, "Channels.Ch2"=w2097) -> (w2096:T10)
                    n777 = Replace Array Subset(array=w2102, new element=w2096, index=w2103) -> (w2100:T14)
                    n778 = global write "Global - Channel.vi" "Data"(w2100) -> ()
                  }
                  frame "Read Sensor" {
                    n779 = Unbundle By Name(w2112) -> ("Ch1 Unit"=w2111:string, "Ch2 Unit"=w2110:string, "Ch1 Decimal"=w2109:u8, "Ch2 Decimal"=w2108:u8)
                    n780 = global read "Global - Unit.vi" "Unit"() -> (w2114:T15)
                    n781 = Build Array(w2111, w2110) -> (w2107:string[])
                    n782 = Build Array(w2109, w2108) -> (w2106:u8[])
                    n783 = Bundle By Name(cluster=T11 {"Name"=[], "Unit"=[], "Decimal Point"=[], "Ch Log"=[], "H Alarm"=[], "L Alarm"=[], "H Limit"=[], "L Limit"=[], "Filter"=[], "Gain"=[], "Calib Type"=[]} ("Sensor"), "Name"=string[] ["Load", "Displacement"], "Unit"=w2107, "Decimal Point"=w2106) -> (w2105:T11)
                    n784 = Replace Array Subset(array=w2114, new element=w2105, index=w2117) -> (w2115:T15)
                    n785 = global write "Global - Unit.vi" "Unit"(w2115) -> ()
                  }
                }
              }
            }
          }
          frame "Close" {
            n786 = global read "Global - Handle V1.vi" "Handle"() -> (w2123:refnum<visa-resource-name>[])
            n787 = Index Array(array=w2123, index=w2119) -> (element=w2122:refnum<visa-resource-name>)
            n788 = VISA Close(VISA resource name=w2122, error in (no error)=w2120) -> (error out=w2121:errorcluster)
          }
        }
      }
      frame Error {
        n789 = global read "Global - IP Address.vi" "IP"() -> (w2136:string[])
        n790 = Unbundle By Name(w2137) -> ("source"=w2133:string)
        n791 = Index Array(array=w2136, index=w2128) -> (element=w2135:string)
        n792 = Concatenate Strings(w2135, " - " ("string"), w2133) -> (w2129:string)
        n793 = call <vilib>:"Clear Errors.vi"("error in (no error)"=w2137) -> ("error out"=w2132:errorcluster)  [unwired: 5 in, 1 out]
        n794 = call "General - Error Log eFGV.vi"("eFGV States"=eFGV_States."Write", "error in (no error)"=w2132, "Error In"=w2129) -> ("error out"=w2131:errorcluster)  [unwired: 6 in, 2 out]
        n795 = Wait (ms)(milliseconds to wait=u32 100) -> ()  [unwired: 1 out]
      }
    }
    "7" <- w1993
    "loop 7" <- w1987
  }
  n796 = while {
    shift-right: [w2150] -> _
    shift-left: errorcluster {"status"=FALSE, "code"=0, "source"=""} ("error IO") -> [w2151]
    shift-right: [w2148] -> _
    shift-left: Communications_-_State."Init" -> [w2149]
    shift-right: [w2146] -> _
    shift-left: _ -> [w2145]
    tunnel: 9 ("index") -> [w2144]
    shift-right: [w2142] -> _
    shift-left: _ -> [w2141]
    i -> [w2143]
    stop <- w2147 stop-if-true
    # "Queue Command Processing Loop"
    n797 = case shown="No Error" w2151 {
      selector: w2151 -> [w2160 w2293]
      tunnel: [w2161 w2288] -> w2150
      tunnel: w2149 -> [w2159 _]
      tunnel: [w2158 Communications_-_State."Idle"] -> w2148
      tunnel: [w2157 _] -> w2147
      tunnel: [w2156 w2295] -> w2146
      tunnel: w2145 -> [w2155 w2295]
      tunnel: w2144 -> [w2154 w2285]
      tunnel: [w2153 w2283] -> w2142
      tunnel: w2141 -> [w2152 w2283]
      frame No Error {
        n798 = case shown="\"Command\"" w2159 {
          tunnel: [w2165 w2185 w2220 w2277] -> w2161
          tunnel: w2160 -> [w2170 w2184 w2223 w2276]
          tunnel: [Communications_-_State."Idle" w2173 Communications_-_State."Idle" Communications_-_State."Close"] -> w2158
          tunnel: [_ _ _ TRUE] -> w2157
          tunnel: [w2167 w2183 w2222 w2280] -> w2156
          tunnel: w2155 -> [_ w2182 w2222 w2280]
          tunnel: w2154 -> [_ w2177 w2209 w2275]
          tunnel: [0 w2172 w2207 0] -> w2153
          tunnel: w2152 -> [_ w2172 w2206 _]
          frame "Init", Default {
            n799 = call "Communication - UDP Command (eFGV).vi"("Action"=eFGV_States."Read", "error in"=w2170) -> ("error out"=w2166:errorcluster, "UDP Ref"=w2164:refnum<user-event>)  [unwired: 7 in, 1 out]
            n800 = register-events(error in=w2166, w2164) -> (reference out=w2163:refnum<event-registration>, error out=w2165:errorcluster)  [unwired: 1 in]
            n801 = Bundle By Name(cluster=T6 {"UDP CMD"={"IP"="", "CMD"=enum."Stop", "Port"="", "Datalog?"=FALSE, "Float"=0.0}, "Unit?"=FALSE, "Read Unit"=[], "Trig?"=FALSE, "UDP Info"=[], "DataLogger"=[], "VISA Ref"=refnum, "Float"=0.0, "Data"={"Test"={"Target Load"=0.0, "Target Disp"=0.0, "Rate"=0.0, "Speed"=0.0}, "Sensor"={"Name"=[], "Unit"=[], "Decimal Point"=[], "Ch Log"=[], "H Alarm"=[], "L Alarm"=[], "H Limit"=[], "L Limit"=[], "Filter"=[], "Gain"=[], "Calib Type"=[]}, "PID"={"SP"=-2.7823365e-08, "PV"=-3.023652e-13, "kP"=8.5432666e-24, "kI"=2.29252e-41, "kD"=1.570387e-38, "FF"=25.0, "Err Band"=0.0, "Max"=15, "Min"=-7, "Ts"=1886611780, "Out"=0, "Mode"=0}, "ADC"={"Active Ch"=[255, 255, 255, 0, 0, 0, 0, 0], "Filter Type"=2, "Post Filter"=[1, 1, 1, 1, 0, 200, 66, 184], "Gain"=[0, 0, 0, 0, 0, 122, 68, 0], "FS"=32, "IntOC"=0, "IntFC"=255, "SysOC"=255, "Cofficient"=[1.0, 1.0, 1.0, 1.0, 1.0, 1.0, 1.0, 1.0], "K"=[1.2450000047683716, 1.2450000047683716], "Max"=1048576}, "System"={"Out Type"=0, "Inverse"=0, "Monitor"=0, "Reserve"=0, "ACC Time"=0, "Pulse Rev"=0, "Stroke"=0, "Auto Off"=0, "Gear Ratio"=0.0, "Pitch"=0.0, "Max Speed"=0, "Jog Speed"=0, "Disp Coff"=0.0, "Max Load"=0}, "Index"=enum."Ch1", "Datalog"=enum."Empty"}, "UDP Event Ref"=refnum, "UDP ref"=refnum, "Read Sensor"=0}, "UDP Event Ref"=w2163) -> (w2167:T6)
          }
          frame "Idle" {
            n802 = Unbundle By Name(w2182) -> ("UDP Event Ref"=w2186:refnum<event-registration>)
            n803 = event shown="[1] <UDP Ref>: User Event" {
              selector: w2186 -> [_ _]
              dyn-events: _ -> [_ _]
              timeout: 3000 -> [_ _]
              tunnel: [w2192 w2195] -> w2180
              tunnel: [w2189 _] -> w2185
              tunnel: w2184 -> [w2189 _]
              tunnel: [w2187 w2204] -> w2183
              tunnel: w2182 -> [w2187 w2203]
              tunnel: w2177 -> [_ w2193]
              event Timeout {
                n804 = event-data() -> ()  [unwired: 1 in, 1 out]
                n805 = local read "Stop"() -> (w2191:bool)
                n806 = Select(t=Communications_-_State."Close", s=w2191, f=Communications_-_State."Idle") -> (s? t:f=w2192:T2)
              }
              event User Event {
                n807 = event-data() -> ("IP"=w2198:string, "CMD"=w2202:T1, "Data"=w2201:T7)  [unwired: 1 in]
                n808 = global read "Global - IP Address.vi" "IP"() -> (w2200:string[])
                n809 = Index Array(array=w2200, index=w2193) -> (element=w2199:string)
                n810 = Equal?(x=w2199, y=w2198) -> (x = y?=w2197:bool)
                n811 = Bundle By Name(cluster=w2203, "UDP CMD.IP"=w2198, "UDP CMD.CMD"=w2202, "Data"=w2201) -> (w2204:T6)
                n812 = Select(t=Communications_-_State."Command" ("f"), s=w2197, f=Communications_-_State."Idle") -> (s? t:f=w2195:T2)
              }
            }
            n813 = global read "Global - Hold.vi" "Hold"() -> (w2181:bool)
            n814 = Select(t=Communications_-_State."Idle", s=w2181, f=w2180) -> (s? t:f=w2174:T2)
            n815 = local read "Stop"() -> (w2175:bool)
            n816 = Select(t=Communications_-_State."Close", s=w2175, f=w2174) -> (s? t:f=w2173:T2)
          }
          frame "Command" {
            n817 = Unbundle By Name(w2222) -> ("UDP CMD.CMD"=w2219:T1, "Data"=w2221:T7, "UDP CMD.IP"=w2205:string)
            "9" <- w2219
            n818 = global read "Global - Handle V1.vi" "Handle"() -> (w2213:refnum<visa-resource-name>[])
            n819 = global read "Global - IP Address.vi" "IP"() -> (w2214:string[])
            n820 = Search 1D Array(1D array=w2214, element=w2205) -> ()  [unwired: 1 in, 1 out]
            n821 = Index Array(array=w2213, index=w2209) -> (element=w2215:refnum<visa-resource-name>)
            n822 = call "VISA - Write CMD.vi"("Index"=w2209, "error in"=w2223, "Data"=w2221, "Action"=w2219, "VISA ref"=w2215) -> ("error out"=w2211:errorcluster, "Data Unit"=w2217:T12, "Data Channel"=w2218:T13, "Success"=w2216:bool, "Prev Data?"=→"Prev 9":bool)  [unwired: 2 out]
            "Success9" <- w2216
            n823 = flat-sequence {
              tunnel: w2209 -> [w2229]
              tunnel: [w2226] -> w2212
              tunnel: w2211 -> [w2226]
              frame #0 {
                n824 = global read "Global - Done.vi" "Done"() -> (w2228:bool[])
                n825 = Replace Array Subset(array=w2228, new element=TRUE, index=w2229) -> (w2227:bool[])
                n826 = global write "Global - Done.vi" "Done"(w2227) -> ()
              }
            }
            n827 = global write "Global - Data UDP.vi" "Loop 10"(TRUE ("Loop 2")) -> ()
            n828 = case shown="False" w2216 {
              tunnel: w2212 -> [w2233 w2248]
              tunnel: [w2234 w2247] -> w2220
              tunnel: w2219 -> [_ w2249]
              tunnel: w2218 -> [_ w2246]
              tunnel: w2217 -> [_ w2245]
              tunnel: w2209 -> [_ w2244]
              tunnel: [w2230 0] -> w2207
              tunnel: w2206 -> [w2235 _]
              tunnel: w2205 -> [w2232 _]
              frame False {
                n829 = Increment(x=w2235) -> (x+1=w2231:i32)
                n830 = case shown="5" w2231 {
                  selector: w2231 -> [w2236 _]
                  tunnel: [w2237 w2241] -> w2234
                  tunnel: w2233 -> [w2237 w2240]
                  tunnel: w2232 -> [_ w2239]
                  tunnel: [w2236 0] -> w2230
                  frame 0, Default {
                  }
                  frame 5 {
                    n831 = call "Communication - Reconnect eFGV.vi"("eFGV States"=eFGV_States."Write", "error in (no error)"=w2240, "Reconnect In"=w2239) -> ("error out"=w2241:errorcluster)  [unwired: 6 in, 2 out]
                  }
                }
              }
              frame True {
                n832 = case shown="\"Read Ch Data\"" w2249 {
                  tunnel: w2248 -> [w2250 w2257 w2272]
                  tunnel: [w2250 w2257 w2272] -> w2247
                  tunnel: w2246 -> [_ w2255 _]
                  tunnel: w2245 -> [_ _ w2268]
                  tunnel: w2244 -> [_ w2259 w2273]
                  frame "Stop", Default {
                  }
                  frame "Read Ch Data" {
                    n833 = Unbundle By Name(w2255) -> ("Ch1 Data"=w2254:sgl, "Ch2 Data"=w2253:sgl)
                    n834 = global read "Global - Channel.vi" "Data"() -> (w2258:T14)
                    n835 = Bundle By Name(cluster=T10 {"Channels"={"Ch1"=0.0, "Ch2"=0.0, "Ch3"=0.0, "Ch4"=0.0, "Ch5"=0.0, "Ch6"=0.0, "Ch7"=0.0, "Ch8"=0.0, "Ch9"=0.0, "Ch10"=0.0, "Ch11"=0.0, "Ch12"=0.0, "Ch13"=0.0, "Ch14"=0.0, "Ch15"=0.0, "Ch16"=0.0}, "Event"=0, "Status"=0, "IP"=""} ("Data Channel"), "Channels.Ch1"=w2254, "Channels.Ch2"=w2253) -> (w2252:T10)
                    n836 = Replace Array Subset(array=w2258, new element=w2252, index=w2259) -> (w2256:T14)
                    n837 = global write "Global - Channel.vi" "Data"(w2256) -> ()
                  }
                  frame "Read Sensor" {
                    n838 = Unbundle By Name(w2268) -> ("Ch1 Unit"=w2267:string, "Ch2 Unit"=w2266:string, "Ch1 Decimal"=w2265:u8, "Ch2 Decimal"=w2264:u8)
                    n839 = global read "Global - Unit.vi" "Unit"() -> (w2270:T15)
                    n840 = Build Array(w2267, w2266) -> (w2263:string[])
                    n841 = Build Array(w2265, w2264) -> (w2262:u8[])
                    n842 = Bundle By Name(cluster=T11 {"Name"=[], "Unit"=[], "Decimal Point"=[], "Ch Log"=[], "H Alarm"=[], "L Alarm"=[], "H Limit"=[], "L Limit"=[], "Filter"=[], "Gain"=[], "Calib Type"=[]} ("Sensor"), "Name"=string[] ["Load", "Displacement"], "Unit"=w2263, "Decimal Point"=w2262) -> (w2261:T11)
                    n843 = Replace Array Subset(array=w2270, new element=w2261, index=w2273) -> (w2271:T15)
                    n844 = global write "Global - Unit.vi" "Unit"(w2271) -> ()
                  }
                }
              }
            }
          }
          frame "Close" {
            n845 = global read "Global - Handle V1.vi" "Handle"() -> (w2279:refnum<visa-resource-name>[])
            n846 = Index Array(array=w2279, index=w2275) -> (element=w2278:refnum<visa-resource-name>)
            n847 = VISA Close(VISA resource name=w2278, error in (no error)=w2276) -> (error out=w2277:errorcluster)
          }
        }
      }
      frame Error {
        n848 = global read "Global - IP Address.vi" "IP"() -> (w2292:string[])
        n849 = Unbundle By Name(w2293) -> ("source"=w2290:string)
        n850 = Index Array(array=w2292, index=w2285) -> (element=w2291:string)
        n851 = Concatenate Strings(w2291, " - " ("string"), w2290) -> (w2286:string)
        n852 = call <vilib>:"Clear Errors.vi"("error in (no error)"=w2293) -> ("error out"=w2289:errorcluster)  [unwired: 5 in, 1 out]
        n853 = call "General - Error Log eFGV.vi"("eFGV States"=eFGV_States."Write", "error in (no error)"=w2289, "Error In"=w2286) -> ("error out"=w2288:errorcluster)  [unwired: 6 in, 2 out]
        n854 = Wait (ms)(milliseconds to wait=u32 100) -> ()  [unwired: 1 out]
      }
    }
    "9" <- w2149
    "loop 9" <- w2143
  }
  n855 = while {
    shift-right: [w2306] -> _
    shift-left: errorcluster {"status"=FALSE, "code"=0, "source"=""} ("error IO") -> [w2307]
    shift-right: [w2304] -> _
    shift-left: Communications_-_State."Init" -> [w2305]
    shift-right: [w2302] -> _
    shift-left: _ -> [w2301]
    tunnel: 11 ("index") -> [w2300]
    shift-right: [w2298] -> _
    shift-left: _ -> [w2297]
    i -> [w2299]
    stop <- w2303 stop-if-true
    # "Queue Command Processing Loop"
    n856 = case shown="No Error" w2307 {
      selector: w2307 -> [w2316 w2449]
      tunnel: [w2317 w2443] -> w2306
      tunnel: w2305 -> [w2315 _]
      tunnel: [w2314 Communications_-_State."Idle"] -> w2304
      tunnel: [w2313 _] -> w2303
      tunnel: [w2312 w2451] -> w2302
      tunnel: w2301 -> [w2311 w2451]
      tunnel: w2300 -> [w2310 w2440]
      tunnel: [w2309 w2439] -> w2298
      tunnel: w2297 -> [w2308 w2439]
      frame No Error {
        n857 = case shown="\"Command\"" w2315 {
          tunnel: [w2321 w2341 w2376 w2433] -> w2317
          tunnel: w2316 -> [w2326 w2340 w2379 w2432]
          tunnel: [Communications_-_State."Idle" w2329 Communications_-_State."Idle" Communications_-_State."Close"] -> w2314
          tunnel: [_ _ _ TRUE] -> w2313
          tunnel: [w2323 w2339 w2378 w2436] -> w2312
          tunnel: w2311 -> [_ w2338 w2378 w2436]
          tunnel: w2310 -> [_ w2333 w2365 w2431]
          tunnel: [0 w2328 w2363 0] -> w2309
          tunnel: w2308 -> [_ w2328 w2362 _]
          frame "Init", Default {
            n858 = call "Communication - UDP Command (eFGV).vi"("Action"=eFGV_States."Read", "error in"=w2326) -> ("error out"=w2322:errorcluster, "UDP Ref"=w2320:refnum<user-event>)  [unwired: 7 in, 1 out]
            n859 = register-events(error in=w2322, w2320) -> (reference out=w2319:refnum<event-registration>, error out=w2321:errorcluster)  [unwired: 1 in]
            n860 = Bundle By Name(cluster=T6 {"UDP CMD"={"IP"="", "CMD"=enum."Stop", "Port"="", "Datalog?"=FALSE, "Float"=0.0}, "Unit?"=FALSE, "Read Unit"=[], "Trig?"=FALSE, "UDP Info"=[], "DataLogger"=[], "VISA Ref"=refnum, "Float"=0.0, "Data"={"Test"={"Target Load"=0.0, "Target Disp"=0.0, "Rate"=0.0, "Speed"=0.0}, "Sensor"={"Name"=[], "Unit"=[], "Decimal Point"=[], "Ch Log"=[], "H Alarm"=[], "L Alarm"=[], "H Limit"=[], "L Limit"=[], "Filter"=[], "Gain"=[], "Calib Type"=[]}, "PID"={"SP"=-2.7823365e-08, "PV"=-3.023652e-13, "kP"=8.5432666e-24, "kI"=2.29252e-41, "kD"=1.570387e-38, "FF"=25.0, "Err Band"=0.0, "Max"=15, "Min"=-7, "Ts"=1886611780, "Out"=0, "Mode"=0}, "ADC"={"Active Ch"=[255, 255, 255, 0, 0, 0, 0, 0], "Filter Type"=2, "Post Filter"=[1, 1, 1, 1, 0, 200, 66, 184], "Gain"=[0, 0, 0, 0, 0, 122, 68, 0], "FS"=32, "IntOC"=0, "IntFC"=255, "SysOC"=255, "Cofficient"=[1.0, 1.0, 1.0, 1.0, 1.0, 1.0, 1.0, 1.0], "K"=[1.2450000047683716, 1.2450000047683716], "Max"=1048576}, "System"={"Out Type"=0, "Inverse"=0, "Monitor"=0, "Reserve"=0, "ACC Time"=0, "Pulse Rev"=0, "Stroke"=0, "Auto Off"=0, "Gear Ratio"=0.0, "Pitch"=0.0, "Max Speed"=0, "Jog Speed"=0, "Disp Coff"=0.0, "Max Load"=0}, "Index"=enum."Ch1", "Datalog"=enum."Empty"}, "UDP Event Ref"=refnum, "UDP ref"=refnum, "Read Sensor"=0}, "UDP Event Ref"=w2319) -> (w2323:T6)
          }
          frame "Idle" {
            n861 = Unbundle By Name(w2338) -> ("UDP Event Ref"=w2342:refnum<event-registration>)
            n862 = event shown="[0] Timeout" {
              selector: w2342 -> [_ _]
              dyn-events: _ -> [_ _]
              timeout: 3000 -> [_ _]
              tunnel: [w2348 w2351] -> w2336
              tunnel: [w2345 _] -> w2341
              tunnel: w2340 -> [w2345 _]
              tunnel: [w2343 w2360] -> w2339
              tunnel: w2338 -> [w2343 w2359]
              tunnel: w2333 -> [_ w2349]
              event Timeout {
                n863 = event-data() -> ()  [unwired: 1 in, 1 out]
                n864 = local read "Stop"() -> (w2347:bool)
                n865 = Select(t=Communications_-_State."Close", s=w2347, f=Communications_-_State."Idle") -> (s? t:f=w2348:T2)
              }
              event User Event {
                n866 = event-data() -> ("IP"=w2354:string, "CMD"=w2358:T1, "Data"=w2357:T7)  [unwired: 1 in]
                n867 = global read "Global - IP Address.vi" "IP"() -> (w2356:string[])
                n868 = Index Array(array=w2356, index=w2349) -> (element=w2355:string)
                n869 = Equal?(x=w2355, y=w2354) -> (x = y?=w2353:bool)
                n870 = Bundle By Name(cluster=w2359, "UDP CMD.IP"=w2354, "UDP CMD.CMD"=w2358, "Data"=w2357) -> (w2360:T6)
                n871 = Select(t=Communications_-_State."Command" ("f"), s=w2353, f=Communications_-_State."Idle") -> (s? t:f=w2351:T2)
              }
            }
            n872 = global read "Global - Hold.vi" "Hold"() -> (w2337:bool)
            n873 = Select(t=Communications_-_State."Idle", s=w2337, f=w2336) -> (s? t:f=w2330:T2)
            n874 = local read "Stop"() -> (w2331:bool)
            n875 = Select(t=Communications_-_State."Close", s=w2331, f=w2330) -> (s? t:f=w2329:T2)
          }
          frame "Command" {
            n876 = Unbundle By Name(w2378) -> ("UDP CMD.CMD"=w2375:T1, "Data"=w2377:T7, "UDP CMD.IP"=w2361:string)
            "11" <- w2375
            n877 = global read "Global - Handle V1.vi" "Handle"() -> (w2369:refnum<visa-resource-name>[])
            n878 = global read "Global - IP Address.vi" "IP"() -> (w2370:string[])
            n879 = Search 1D Array(1D array=w2370, element=w2361) -> ()  [unwired: 1 in, 1 out]
            n880 = Index Array(array=w2369, index=w2365) -> (element=w2371:refnum<visa-resource-name>)
            n881 = call "VISA - Write CMD.vi"("Index"=w2365, "error in"=w2379, "Data"=w2377, "Action"=w2375, "VISA ref"=w2371) -> ("error out"=w2367:errorcluster, "Data Unit"=w2373:T12, "Data Channel"=w2374:T13, "Success"=w2372:bool, "Prev Data?"=→"Prev 11":bool)  [unwired: 2 out]
            "Success11" <- w2372
            n882 = flat-sequence {
              tunnel: w2365 -> [w2385]
              tunnel: [w2382] -> w2368
              tunnel: w2367 -> [w2382]
              frame #0 {
                n883 = global read "Global - Done.vi" "Done"() -> (w2384:bool[])
                n884 = Replace Array Subset(array=w2384, new element=TRUE, index=w2385) -> (w2383:bool[])
                n885 = global write "Global - Done.vi" "Done"(w2383) -> ()
              }
            }
            n886 = global write "Global - Data UDP.vi" "Loop 12"(TRUE ("Loop 4")) -> ()
            n887 = case shown="False" w2372 {
              tunnel: w2368 -> [w2389 w2404]
              tunnel: [w2390 w2403] -> w2376
              tunnel: w2375 -> [_ w2405]
              tunnel: w2374 -> [_ w2402]
              tunnel: w2373 -> [_ w2401]
              tunnel: w2365 -> [_ w2400]
              tunnel: [w2386 0] -> w2363
              tunnel: w2362 -> [w2391 _]
              tunnel: w2361 -> [w2388 _]
              frame False {
                n888 = Increment(x=w2391) -> (x+1=w2387:i32)
                n889 = case shown="5" w2387 {
                  selector: w2387 -> [w2392 _]
                  tunnel: [w2393 w2397] -> w2390
                  tunnel: w2389 -> [w2393 w2396]
                  tunnel: w2388 -> [_ w2395]
                  tunnel: [w2392 0] -> w2386
                  frame 0, Default {
                  }
                  frame 5 {
                    n890 = call "Communication - Reconnect eFGV.vi"("eFGV States"=eFGV_States."Write", "error in (no error)"=w2396, "Reconnect In"=w2395) -> ("error out"=w2397:errorcluster)  [unwired: 6 in, 2 out]
                  }
                }
              }
              frame True {
                n891 = case shown="\"Read Ch Data\"" w2405 {
                  tunnel: w2404 -> [w2406 w2413 w2428]
                  tunnel: [w2406 w2413 w2428] -> w2403
                  tunnel: w2402 -> [_ w2411 _]
                  tunnel: w2401 -> [_ _ w2424]
                  tunnel: w2400 -> [_ w2415 w2429]
                  frame "Stop", Default {
                  }
                  frame "Read Ch Data" {
                    n892 = Unbundle By Name(w2411) -> ("Ch1 Data"=w2410:sgl, "Ch2 Data"=w2409:sgl)
                    n893 = global read "Global - Channel.vi" "Data"() -> (w2414:T14)
                    n894 = Bundle By Name(cluster=T10 {"Channels"={"Ch1"=0.0, "Ch2"=0.0, "Ch3"=0.0, "Ch4"=0.0, "Ch5"=0.0, "Ch6"=0.0, "Ch7"=0.0, "Ch8"=0.0, "Ch9"=0.0, "Ch10"=0.0, "Ch11"=0.0, "Ch12"=0.0, "Ch13"=0.0, "Ch14"=0.0, "Ch15"=0.0, "Ch16"=0.0}, "Event"=0, "Status"=0, "IP"=""} ("Data Channel"), "Channels.Ch1"=w2410, "Channels.Ch2"=w2409) -> (w2408:T10)
                    n895 = Replace Array Subset(array=w2414, new element=w2408, index=w2415) -> (w2412:T14)
                    n896 = global write "Global - Channel.vi" "Data"(w2412) -> ()
                  }
                  frame "Read Sensor" {
                    n897 = Unbundle By Name(w2424) -> ("Ch1 Unit"=w2423:string, "Ch2 Unit"=w2422:string, "Ch1 Decimal"=w2421:u8, "Ch2 Decimal"=w2420:u8)
                    n898 = global read "Global - Unit.vi" "Unit"() -> (w2426:T15)
                    n899 = Build Array(w2423, w2422) -> (w2419:string[])
                    n900 = Build Array(w2421, w2420) -> (w2418:u8[])
                    n901 = Bundle By Name(cluster=T11 {"Name"=[], "Unit"=[], "Decimal Point"=[], "Ch Log"=[], "H Alarm"=[], "L Alarm"=[], "H Limit"=[], "L Limit"=[], "Filter"=[], "Gain"=[], "Calib Type"=[]} ("Sensor"), "Name"=string[] ["Load", "Displacement"], "Unit"=w2419, "Decimal Point"=w2418) -> (w2417:T11)
                    n902 = Replace Array Subset(array=w2426, new element=w2417, index=w2429) -> (w2427:T15)
                    n903 = global write "Global - Unit.vi" "Unit"(w2427) -> ()
                  }
                }
              }
            }
          }
          frame "Close" {
            n904 = global read "Global - Handle V1.vi" "Handle"() -> (w2435:refnum<visa-resource-name>[])
            n905 = Index Array(array=w2435, index=w2431) -> (element=w2434:refnum<visa-resource-name>)
            n906 = VISA Close(VISA resource name=w2434, error in (no error)=w2432) -> (error out=w2433:errorcluster)
          }
        }
      }
      frame Error {
        n907 = global read "Global - IP Address.vi" "IP"() -> (w2448:string[])
        n908 = Unbundle By Name(w2449) -> ("source"=w2445:string)
        n909 = Index Array(array=w2448, index=w2440) -> (element=w2447:string)
        n910 = Concatenate Strings(w2447, " - " ("string"), w2445) -> (w2441:string)
        n911 = call <vilib>:"Clear Errors.vi"("error in (no error)"=w2449) -> ("error out"=w2444:errorcluster)  [unwired: 5 in, 1 out]
        n912 = call "General - Error Log eFGV.vi"("eFGV States"=eFGV_States."Write", "error in (no error)"=w2444, "Error In"=w2441) -> ("error out"=w2443:errorcluster)  [unwired: 6 in, 2 out]
        n913 = Wait (ms)(milliseconds to wait=u32 100) -> ()  [unwired: 1 out]
      }
    }
    "11" <- w2305
    "loop 11" <- w2299
  }
  n914 = while {
    shift-right: [w2462] -> _
    shift-left: errorcluster {"status"=FALSE, "code"=0, "source"=""} ("error IO") -> [w2463]
    shift-right: [w2460] -> _
    shift-left: Communications_-_State."Init" -> [w2461]
    shift-right: [w2458] -> _
    shift-left: _ -> [w2457]
    tunnel: 13 ("index") -> [w2456]
    shift-right: [w2454] -> _
    shift-left: _ -> [w2453]
    i -> [w2455]
    stop <- w2459 stop-if-true
    # "Queue Command Processing Loop"
    n915 = case shown="No Error" w2463 {
      selector: w2463 -> [w2472 w2605]
      tunnel: [w2473 w2600] -> w2462
      tunnel: w2461 -> [w2471 _]
      tunnel: [w2470 Communications_-_State."Idle"] -> w2460
      tunnel: [w2469 _] -> w2459
      tunnel: [w2468 w2607] -> w2458
      tunnel: w2457 -> [w2467 w2607]
      tunnel: w2456 -> [w2466 w2597]
      tunnel: [w2465 w2595] -> w2454
      tunnel: w2453 -> [w2464 w2595]
      frame No Error {
        n916 = case shown="\"Command\"" w2471 {
          tunnel: [w2477 w2497 w2532 w2589] -> w2473
          tunnel: w2472 -> [w2482 w2496 w2535 w2588]
          tunnel: [Communications_-_State."Idle" w2485 Communications_-_State."Idle" Communications_-_State."Close"] -> w2470
          tunnel: [_ _ _ TRUE] -> w2469
          tunnel: [w2479 w2495 w2534 w2592] -> w2468
          tunnel: w2467 -> [_ w2494 w2534 w2592]
          tunnel: w2466 -> [_ w2489 w2521 w2587]
          tunnel: [0 w2484 w2519 0] -> w2465
          tunnel: w2464 -> [_ w2484 w2518 _]
          frame "Init", Default {
            n917 = call "Communication - UDP Command (eFGV).vi"("Action"=eFGV_States."Read", "error in"=w2482) -> ("error out"=w2478:errorcluster, "UDP Ref"=w2476:refnum<user-event>)  [unwired: 7 in, 1 out]
            n918 = register-events(error in=w2478, w2476) -> (reference out=w2475:refnum<event-registration>, error out=w2477:errorcluster)  [unwired: 1 in]
            n919 = Bundle By Name(cluster=T6 {"UDP CMD"={"IP"="", "CMD"=enum."Stop", "Port"="", "Datalog?"=FALSE, "Float"=0.0}, "Unit?"=FALSE, "Read Unit"=[], "Trig?"=FALSE, "UDP Info"=[], "DataLogger"=[], "VISA Ref"=refnum, "Float"=0.0, "Data"={"Test"={"Target Load"=0.0, "Target Disp"=0.0, "Rate"=0.0, "Speed"=0.0}, "Sensor"={"Name"=[], "Unit"=[], "Decimal Point"=[], "Ch Log"=[], "H Alarm"=[], "L Alarm"=[], "H Limit"=[], "L Limit"=[], "Filter"=[], "Gain"=[], "Calib Type"=[]}, "PID"={"SP"=-2.7823365e-08, "PV"=-3.023652e-13, "kP"=8.5432666e-24, "kI"=2.29252e-41, "kD"=1.570387e-38, "FF"=25.0, "Err Band"=0.0, "Max"=15, "Min"=-7, "Ts"=1886611780, "Out"=0, "Mode"=0}, "ADC"={"Active Ch"=[255, 255, 255, 0, 0, 0, 0, 0], "Filter Type"=2, "Post Filter"=[1, 1, 1, 1, 0, 200, 66, 184], "Gain"=[0, 0, 0, 0, 0, 122, 68, 0], "FS"=32, "IntOC"=0, "IntFC"=255, "SysOC"=255, "Cofficient"=[1.0, 1.0, 1.0, 1.0, 1.0, 1.0, 1.0, 1.0], "K"=[1.2450000047683716, 1.2450000047683716], "Max"=1048576}, "System"={"Out Type"=0, "Inverse"=0, "Monitor"=0, "Reserve"=0, "ACC Time"=0, "Pulse Rev"=0, "Stroke"=0, "Auto Off"=0, "Gear Ratio"=0.0, "Pitch"=0.0, "Max Speed"=0, "Jog Speed"=0, "Disp Coff"=0.0, "Max Load"=0}, "Index"=enum."Ch1", "Datalog"=enum."Empty"}, "UDP Event Ref"=refnum, "UDP ref"=refnum, "Read Sensor"=0}, "UDP Event Ref"=w2475) -> (w2479:T6)
          }
          frame "Idle" {
            n920 = Unbundle By Name(w2494) -> ("UDP Event Ref"=w2498:refnum<event-registration>)
            n921 = event shown="[1] <UDP Ref>: User Event" {
              selector: w2498 -> [_ _]
              dyn-events: _ -> [_ _]
              timeout: 3000 -> [_ _]
              tunnel: [w2504 w2507] -> w2492
              tunnel: [w2501 _] -> w2497
              tunnel: w2496 -> [w2501 _]
              tunnel: [w2499 w2516] -> w2495
              tunnel: w2494 -> [w2499 w2515]
              tunnel: w2489 -> [_ w2505]
              event Timeout {
                n922 = event-data() -> ()  [unwired: 1 in, 1 out]
                n923 = local read "Stop"() -> (w2503:bool)
                n924 = Select(t=Communications_-_State."Close", s=w2503, f=Communications_-_State."Idle") -> (s? t:f=w2504:T2)
              }
              event User Event {
                n925 = event-data() -> ("IP"=w2510:string, "CMD"=w2514:T1, "Data"=w2513:T7)  [unwired: 1 in]
                n926 = global read "Global - IP Address.vi" "IP"() -> (w2512:string[])
                n927 = Index Array(array=w2512, index=w2505) -> (element=w2511:string)
                n928 = Equal?(x=w2511, y=w2510) -> (x = y?=w2509:bool)
                n929 = Bundle By Name(cluster=w2515, "UDP CMD.IP"=w2510, "UDP CMD.CMD"=w2514, "Data"=w2513) -> (w2516:T6)
                n930 = Select(t=Communications_-_State."Command" ("f"), s=w2509, f=Communications_-_State."Idle") -> (s? t:f=w2507:T2)
              }
            }
            n931 = global read "Global - Hold.vi" "Hold"() -> (w2493:bool)
            n932 = Select(t=Communications_-_State."Idle", s=w2493, f=w2492) -> (s? t:f=w2486:T2)
            n933 = local read "Stop"() -> (w2487:bool)
            n934 = Select(t=Communications_-_State."Close", s=w2487, f=w2486) -> (s? t:f=w2485:T2)
          }
          frame "Command" {
            n935 = Unbundle By Name(w2534) -> ("UDP CMD.CMD"=w2531:T1, "Data"=w2533:T7, "UDP CMD.IP"=w2517:string)
            "13" <- w2531
            n936 = global read "Global - Handle V1.vi" "Handle"() -> (w2525:refnum<visa-resource-name>[])
            n937 = global read "Global - IP Address.vi" "IP"() -> (w2526:string[])
            n938 = Search 1D Array(1D array=w2526, element=w2517) -> ()  [unwired: 1 in, 1 out]
            n939 = Index Array(array=w2525, index=w2521) -> (element=w2527:refnum<visa-resource-name>)
            n940 = call "VISA - Write CMD.vi"("Index"=w2521, "error in"=w2535, "Data"=w2533, "Action"=w2531, "VISA ref"=w2527) -> ("error out"=w2523:errorcluster, "Data Unit"=w2529:T12, "Data Channel"=w2530:T13, "Success"=w2528:bool, "Prev Data?"=→"Prev 13":bool)  [unwired: 2 out]
            "Success13" <- w2528
            n941 = flat-sequence {
              tunnel: w2521 -> [w2541]
              tunnel: [w2538] -> w2524
              tunnel: w2523 -> [w2538]
              frame #0 {
                n942 = global read "Global - Done.vi" "Done"() -> (w2540:bool[])
                n943 = Replace Array Subset(array=w2540, new element=TRUE, index=w2541) -> (w2539:bool[])
                n944 = global write "Global - Done.vi" "Done"(w2539) -> ()
              }
            }
            n945 = global write "Global - Data UDP.vi" "Loop 14"(TRUE ("Loop 2")) -> ()
            n946 = case shown="False" w2528 {
              tunnel: w2524 -> [w2545 w2560]
              tunnel: [w2546 w2559] -> w2532
              tunnel: w2531 -> [_ w2561]
              tunnel: w2530 -> [_ w2558]
              tunnel: w2529 -> [_ w2557]
              tunnel: w2521 -> [_ w2556]
              tunnel: [w2542 0] -> w2519
              tunnel: w2518 -> [w2547 _]
              tunnel: w2517 -> [w2544 _]
              frame False {
                n947 = Increment(x=w2547) -> (x+1=w2543:i32)
                n948 = case shown="5" w2543 {
                  selector: w2543 -> [w2548 _]
                  tunnel: [w2549 w2553] -> w2546
                  tunnel: w2545 -> [w2549 w2552]
                  tunnel: w2544 -> [_ w2551]
                  tunnel: [w2548 0] -> w2542
                  frame 0, Default {
                  }
                  frame 5 {
                    n949 = call "Communication - Reconnect eFGV.vi"("eFGV States"=eFGV_States."Write", "error in (no error)"=w2552, "Reconnect In"=w2551) -> ("error out"=w2553:errorcluster)  [unwired: 6 in, 2 out]
                  }
                }
              }
              frame True {
                n950 = case shown="\"Read Ch Data\"" w2561 {
                  tunnel: w2560 -> [w2562 w2569 w2584]
                  tunnel: [w2562 w2569 w2584] -> w2559
                  tunnel: w2558 -> [_ w2567 _]
                  tunnel: w2557 -> [_ _ w2580]
                  tunnel: w2556 -> [_ w2571 w2585]
                  frame "Stop", Default {
                  }
                  frame "Read Ch Data" {
                    n951 = Unbundle By Name(w2567) -> ("Ch1 Data"=w2566:sgl, "Ch2 Data"=w2565:sgl)
                    n952 = global read "Global - Channel.vi" "Data"() -> (w2570:T14)
                    n953 = Bundle By Name(cluster=T10 {"Channels"={"Ch1"=0.0, "Ch2"=0.0, "Ch3"=0.0, "Ch4"=0.0, "Ch5"=0.0, "Ch6"=0.0, "Ch7"=0.0, "Ch8"=0.0, "Ch9"=0.0, "Ch10"=0.0, "Ch11"=0.0, "Ch12"=0.0, "Ch13"=0.0, "Ch14"=0.0, "Ch15"=0.0, "Ch16"=0.0}, "Event"=0, "Status"=0, "IP"=""} ("Data Channel"), "Channels.Ch1"=w2566, "Channels.Ch2"=w2565) -> (w2564:T10)
                    n954 = Replace Array Subset(array=w2570, new element=w2564, index=w2571) -> (w2568:T14)
                    n955 = global write "Global - Channel.vi" "Data"(w2568) -> ()
                  }
                  frame "Read Sensor" {
                    n956 = Unbundle By Name(w2580) -> ("Ch1 Unit"=w2579:string, "Ch2 Unit"=w2578:string, "Ch1 Decimal"=w2577:u8, "Ch2 Decimal"=w2576:u8)
                    n957 = global read "Global - Unit.vi" "Unit"() -> (w2582:T15)
                    n958 = Build Array(w2579, w2578) -> (w2575:string[])
                    n959 = Build Array(w2577, w2576) -> (w2574:u8[])
                    n960 = Bundle By Name(cluster=T11 {"Name"=[], "Unit"=[], "Decimal Point"=[], "Ch Log"=[], "H Alarm"=[], "L Alarm"=[], "H Limit"=[], "L Limit"=[], "Filter"=[], "Gain"=[], "Calib Type"=[]} ("Sensor"), "Name"=string[] ["Load", "Displacement"], "Unit"=w2575, "Decimal Point"=w2574) -> (w2573:T11)
                    n961 = Replace Array Subset(array=w2582, new element=w2573, index=w2585) -> (w2583:T15)
                    n962 = global write "Global - Unit.vi" "Unit"(w2583) -> ()
                  }
                }
              }
            }
          }
          frame "Close" {
            n963 = global read "Global - Handle V1.vi" "Handle"() -> (w2591:refnum<visa-resource-name>[])
            n964 = Index Array(array=w2591, index=w2587) -> (element=w2590:refnum<visa-resource-name>)
            n965 = VISA Close(VISA resource name=w2590, error in (no error)=w2588) -> (error out=w2589:errorcluster)
          }
        }
      }
      frame Error {
        n966 = global read "Global - IP Address.vi" "IP"() -> (w2604:string[])
        n967 = Unbundle By Name(w2605) -> ("source"=w2602:string)
        n968 = Index Array(array=w2604, index=w2597) -> (element=w2603:string)
        n969 = Concatenate Strings(w2603, " - " ("string"), w2602) -> (w2598:string)
        n970 = call <vilib>:"Clear Errors.vi"("error in (no error)"=w2605) -> ("error out"=w2601:errorcluster)  [unwired: 5 in, 1 out]
        n971 = call "General - Error Log eFGV.vi"("eFGV States"=eFGV_States."Write", "error in (no error)"=w2601, "Error In"=w2598) -> ("error out"=w2600:errorcluster)  [unwired: 6 in, 2 out]
        n972 = Wait (ms)(milliseconds to wait=u32 100) -> ()  [unwired: 1 out]
      }
    }
    "13" <- w2461
    "loop 13" <- w2455
  }
  n973 = while {
    shift-right: [w2618] -> _
    shift-left: errorcluster {"status"=FALSE, "code"=0, "source"=""} ("error IO") -> [w2619]
    shift-right: [w2616] -> _
    shift-left: Communications_-_State."Init" -> [w2617]
    shift-right: [w2614] -> _
    shift-left: _ -> [w2613]
    tunnel: 15 ("index") -> [w2612]
    shift-right: [w2610] -> _
    shift-left: _ -> [w2609]
    i -> [w2611]
    stop <- w2615 stop-if-true
    # "Queue Command Processing Loop"
    n974 = case shown="No Error" w2619 {
      selector: w2619 -> [w2628 w2761]
      tunnel: [w2629 w2755] -> w2618
      tunnel: w2617 -> [w2627 _]
      tunnel: [w2626 Communications_-_State."Idle"] -> w2616
      tunnel: [w2625 _] -> w2615
      tunnel: [w2624 w2763] -> w2614
      tunnel: w2613 -> [w2623 w2763]
      tunnel: w2612 -> [w2622 w2752]
      tunnel: [w2621 w2751] -> w2610
      tunnel: w2609 -> [w2620 w2751]
      frame No Error {
        n975 = case shown="\"Command\"" w2627 {
          tunnel: [w2633 w2653 w2688 w2745] -> w2629
          tunnel: w2628 -> [w2638 w2652 w2691 w2744]
          tunnel: [Communications_-_State."Idle" w2641 Communications_-_State."Idle" Communications_-_State."Close"] -> w2626
          tunnel: [_ _ _ TRUE] -> w2625
          tunnel: [w2635 w2651 w2690 w2748] -> w2624
          tunnel: w2623 -> [_ w2650 w2690 w2748]
          tunnel: w2622 -> [_ w2645 w2677 w2743]
          tunnel: [0 w2640 w2675 0] -> w2621
          tunnel: w2620 -> [_ w2640 w2674 _]
          frame "Init", Default {
            n976 = call "Communication - UDP Command (eFGV).vi"("Action"=eFGV_States."Read", "error in"=w2638) -> ("error out"=w2634:errorcluster, "UDP Ref"=w2632:refnum<user-event>)  [unwired: 7 in, 1 out]
            n977 = register-events(error in=w2634, w2632) -> (reference out=w2631:refnum<event-registration>, error out=w2633:errorcluster)  [unwired: 1 in]
            n978 = Bundle By Name(cluster=T6 {"UDP CMD"={"IP"="", "CMD"=enum."Stop", "Port"="", "Datalog?"=FALSE, "Float"=0.0}, "Unit?"=FALSE, "Read Unit"=[], "Trig?"=FALSE, "UDP Info"=[], "DataLogger"=[], "VISA Ref"=refnum, "Float"=0.0, "Data"={"Test"={"Target Load"=0.0, "Target Disp"=0.0, "Rate"=0.0, "Speed"=0.0}, "Sensor"={"Name"=[], "Unit"=[], "Decimal Point"=[], "Ch Log"=[], "H Alarm"=[], "L Alarm"=[], "H Limit"=[], "L Limit"=[], "Filter"=[], "Gain"=[], "Calib Type"=[]}, "PID"={"SP"=-2.7823365e-08, "PV"=-3.023652e-13, "kP"=8.5432666e-24, "kI"=2.29252e-41, "kD"=1.570387e-38, "FF"=25.0, "Err Band"=0.0, "Max"=15, "Min"=-7, "Ts"=1886611780, "Out"=0, "Mode"=0}, "ADC"={"Active Ch"=[255, 255, 255, 0, 0, 0, 0, 0], "Filter Type"=2, "Post Filter"=[1, 1, 1, 1, 0, 200, 66, 184], "Gain"=[0, 0, 0, 0, 0, 122, 68, 0], "FS"=32, "IntOC"=0, "IntFC"=255, "SysOC"=255, "Cofficient"=[1.0, 1.0, 1.0, 1.0, 1.0, 1.0, 1.0, 1.0], "K"=[1.2450000047683716, 1.2450000047683716], "Max"=1048576}, "System"={"Out Type"=0, "Inverse"=0, "Monitor"=0, "Reserve"=0, "ACC Time"=0, "Pulse Rev"=0, "Stroke"=0, "Auto Off"=0, "Gear Ratio"=0.0, "Pitch"=0.0, "Max Speed"=0, "Jog Speed"=0, "Disp Coff"=0.0, "Max Load"=0}, "Index"=enum."Ch1", "Datalog"=enum."Empty"}, "UDP Event Ref"=refnum, "UDP ref"=refnum, "Read Sensor"=0}, "UDP Event Ref"=w2631) -> (w2635:T6)
          }
          frame "Idle" {
            n979 = Unbundle By Name(w2650) -> ("UDP Event Ref"=w2654:refnum<event-registration>)
            n980 = event shown="[0] Timeout" {
              selector: w2654 -> [_ _]
              dyn-events: _ -> [_ _]
              timeout: 3000 -> [_ _]
              tunnel: [w2660 w2663] -> w2648
              tunnel: [w2657 _] -> w2653
              tunnel: w2652 -> [w2657 _]
              tunnel: [w2655 w2672] -> w2651
              tunnel: w2650 -> [w2655 w2671]
              tunnel: w2645 -> [_ w2661]
              event Timeout {
                n981 = event-data() -> ()  [unwired: 1 in, 1 out]
                n982 = local read "Stop"() -> (w2659:bool)
                n983 = Select(t=Communications_-_State."Close", s=w2659, f=Communications_-_State."Idle") -> (s? t:f=w2660:T2)
              }
              event User Event {
                n984 = event-data() -> ("IP"=w2666:string, "CMD"=w2670:T1, "Data"=w2669:T7)  [unwired: 1 in]
                n985 = global read "Global - IP Address.vi" "IP"() -> (w2668:string[])
                n986 = Index Array(array=w2668, index=w2661) -> (element=w2667:string)
                n987 = Equal?(x=w2667, y=w2666) -> (x = y?=w2665:bool)
                n988 = Bundle By Name(cluster=w2671, "UDP CMD.IP"=w2666, "UDP CMD.CMD"=w2670, "Data"=w2669) -> (w2672:T6)
                n989 = Select(t=Communications_-_State."Command" ("f"), s=w2665, f=Communications_-_State."Idle") -> (s? t:f=w2663:T2)
              }
            }
            n990 = global read "Global - Hold.vi" "Hold"() -> (w2649:bool)
            n991 = Select(t=Communications_-_State."Idle", s=w2649, f=w2648) -> (s? t:f=w2642:T2)
            n992 = local read "Stop"() -> (w2643:bool)
            n993 = Select(t=Communications_-_State."Close", s=w2643, f=w2642) -> (s? t:f=w2641:T2)
          }
          frame "Command" {
            n994 = Unbundle By Name(w2690) -> ("UDP CMD.CMD"=w2687:T1, "Data"=w2689:T7, "UDP CMD.IP"=w2673:string)
            "15" <- w2687
            n995 = global read "Global - Handle V1.vi" "Handle"() -> (w2681:refnum<visa-resource-name>[])
            n996 = global read "Global - IP Address.vi" "IP"() -> (w2682:string[])
            n997 = Search 1D Array(1D array=w2682, element=w2673) -> ()  [unwired: 1 in, 1 out]
            n998 = Index Array(array=w2681, index=w2677) -> (element=w2683:refnum<visa-resource-name>)
            n999 = call "VISA - Write CMD.vi"("Index"=w2677, "error in"=w2691, "Data"=w2689, "Action"=w2687, "VISA ref"=w2683) -> ("error out"=w2679:errorcluster, "Data Unit"=w2685:T12, "Data Channel"=w2686:T13, "Success"=w2684:bool, "Prev Data?"=→"Prev15":bool)  [unwired: 2 out]
            "Success15" <- w2684
            n1000 = flat-sequence {
              tunnel: w2677 -> [w2697]
              tunnel: [w2694] -> w2680
              tunnel: w2679 -> [w2694]
              frame #0 {
                n1001 = global read "Global - Done.vi" "Done"() -> (w2696:bool[])
                n1002 = Replace Array Subset(array=w2696, new element=TRUE, index=w2697) -> (w2695:bool[])
                n1003 = global write "Global - Done.vi" "Done"(w2695) -> ()
              }
            }
            n1004 = global write "Global - Data UDP.vi" "Loop 16"(TRUE ("Loop 4")) -> ()
            n1005 = case shown="False" w2684 {
              tunnel: w2680 -> [w2701 w2716]
              tunnel: [w2702 w2715] -> w2688
              tunnel: w2687 -> [_ w2717]
              tunnel: w2686 -> [_ w2714]
              tunnel: w2685 -> [_ w2713]
              tunnel: w2677 -> [_ w2712]
              tunnel: [w2698 0] -> w2675
              tunnel: w2674 -> [w2703 _]
              tunnel: w2673 -> [w2700 _]
              frame False {
                n1006 = Increment(x=w2703) -> (x+1=w2699:i32)
                n1007 = case shown="5" w2699 {
                  selector: w2699 -> [w2704 _]
                  tunnel: [w2705 w2709] -> w2702
                  tunnel: w2701 -> [w2705 w2708]
                  tunnel: w2700 -> [_ w2707]
                  tunnel: [w2704 0] -> w2698
                  frame 0, Default {
                  }
                  frame 5 {
                    n1008 = call "Communication - Reconnect eFGV.vi"("eFGV States"=eFGV_States."Write", "error in (no error)"=w2708, "Reconnect In"=w2707) -> ("error out"=w2709:errorcluster)  [unwired: 6 in, 2 out]
                  }
                }
              }
              frame True {
                n1009 = case shown="\"Read Ch Data\"" w2717 {
                  tunnel: w2716 -> [w2718 w2725 w2740]
                  tunnel: [w2718 w2725 w2740] -> w2715
                  tunnel: w2714 -> [_ w2723 _]
                  tunnel: w2713 -> [_ _ w2736]
                  tunnel: w2712 -> [_ w2727 w2741]
                  frame "Stop", Default {
                  }
                  frame "Read Ch Data" {
                    n1010 = Unbundle By Name(w2723) -> ("Ch1 Data"=w2722:sgl, "Ch2 Data"=w2721:sgl)
                    n1011 = global read "Global - Channel.vi" "Data"() -> (w2726:T14)
                    n1012 = Bundle By Name(cluster=T10 {"Channels"={"Ch1"=0.0, "Ch2"=0.0, "Ch3"=0.0, "Ch4"=0.0, "Ch5"=0.0, "Ch6"=0.0, "Ch7"=0.0, "Ch8"=0.0, "Ch9"=0.0, "Ch10"=0.0, "Ch11"=0.0, "Ch12"=0.0, "Ch13"=0.0, "Ch14"=0.0, "Ch15"=0.0, "Ch16"=0.0}, "Event"=0, "Status"=0, "IP"=""} ("Data Channel"), "Channels.Ch1"=w2722, "Channels.Ch2"=w2721) -> (w2720:T10)
                    n1013 = Replace Array Subset(array=w2726, new element=w2720, index=w2727) -> (w2724:T14)
                    n1014 = global write "Global - Channel.vi" "Data"(w2724) -> ()
                  }
                  frame "Read Sensor" {
                    n1015 = Unbundle By Name(w2736) -> ("Ch1 Unit"=w2735:string, "Ch2 Unit"=w2734:string, "Ch1 Decimal"=w2733:u8, "Ch2 Decimal"=w2732:u8)
                    n1016 = global read "Global - Unit.vi" "Unit"() -> (w2738:T15)
                    n1017 = Build Array(w2735, w2734) -> (w2731:string[])
                    n1018 = Build Array(w2733, w2732) -> (w2730:u8[])
                    n1019 = Bundle By Name(cluster=T11 {"Name"=[], "Unit"=[], "Decimal Point"=[], "Ch Log"=[], "H Alarm"=[], "L Alarm"=[], "H Limit"=[], "L Limit"=[], "Filter"=[], "Gain"=[], "Calib Type"=[]} ("Sensor"), "Name"=string[] ["Load", "Displacement"], "Unit"=w2731, "Decimal Point"=w2730) -> (w2729:T11)
                    n1020 = Replace Array Subset(array=w2738, new element=w2729, index=w2741) -> (w2739:T15)
                    n1021 = global write "Global - Unit.vi" "Unit"(w2739) -> ()
                  }
                }
              }
            }
          }
          frame "Close" {
            n1022 = global read "Global - Handle V1.vi" "Handle"() -> (w2747:refnum<visa-resource-name>[])
            n1023 = Index Array(array=w2747, index=w2743) -> (element=w2746:refnum<visa-resource-name>)
            n1024 = VISA Close(VISA resource name=w2746, error in (no error)=w2744) -> (error out=w2745:errorcluster)
          }
        }
      }
      frame Error {
        n1025 = global read "Global - IP Address.vi" "IP"() -> (w2760:string[])
        n1026 = Unbundle By Name(w2761) -> ("source"=w2757:string)
        n1027 = Index Array(array=w2760, index=w2752) -> (element=w2759:string)
        n1028 = Concatenate Strings(w2759, " - " ("string"), w2757) -> (w2753:string)
        n1029 = call <vilib>:"Clear Errors.vi"("error in (no error)"=w2761) -> ("error out"=w2756:errorcluster)  [unwired: 5 in, 1 out]
        n1030 = call "General - Error Log eFGV.vi"("eFGV States"=eFGV_States."Write", "error in (no error)"=w2756, "Error In"=w2753) -> ("error out"=w2755:errorcluster)  [unwired: 6 in, 2 out]
        n1031 = Wait (ms)(milliseconds to wait=u32 100) -> ()  [unwired: 1 out]
      }
    }
    "15" <- w2617
    "loop 15" <- w2611
  }
  n1032 = control-ref of="This VI"() -> (w2:refnum<vi>)
  n1033 = invoke class="VI" method="FP.Open"(reference=w2, error in=w1, "Activate"=TRUE ("Activate?"), "State"=T3."Closed") -> ()  [unwired: 1 in, 5 out]
